vi "PRAT Test Setup.vi"(0 "Station Input":string="A", 1 "Test Sequence Input":T21[](array[typedef]) {"Time" format="%<%H:%M:%S>t"}, 3 "Washer Controls In":T9={"Test Fixture Hardware"={"Power "={"Yokogawa"={"WT210"={"Sample Rate (1: 0.25s)"=1, "A Range (12: 20A)"=12, "V Range (6: 600V)"=4, "Power VISA Yokogawa WT210"="WT210"}, "WT500"={"Power VISA Yokogawa WT500"="WT500", "V Range (8: 1000V)"=0, "I Range (7: 40A)"=0, "Update Rate (3: 500ms)"=2}, "WT310_2"={"Sample Rate (1: 0.25s)"=1, "A Range (12: 20A)"=11, "V Range (6: 600V)"=4, "Power VISA Yokogawa WT310_2"="WT310_2"}, "WT310_3"={"Sample Rate (1: 0.25s)"=1, "A Range (12: 20A)"=11, "V Range (6: 600V)"=4, "Power VISA Yokogawa WT310_3"="WT310_3"}}, "Aplus"={"Aplus IP Address"="192.168.1.101", "Remote Port"=502, "Instrument"="APLUS", "Instr Driver Revision"="1.03.0053"}, "Power Limits"={"Crest Factor"={"Upper Limit"=1.49, "Lower Limit"=1.34}, "Harmonic Content"={"Uthd"=2.0}, "Voltage"={"% Error"=2.0}, "Stability"={"<1 Watt "={"Wattage"=1.0, "Slope (mW/H)"=10.0}, ">1 Watt"={"1%Power/Hour"=1.0}}}, "Nominal Voltage"=120, "Time Limit (s)"=10800.0, "Power Variation Limit (%)"=50.0, "Power Supply"={"Chroma 61605"="CHROMA", "Use Chroma?"=FALSE}}, "Weight Scale"={"Com Options"={"IND560Scale VISA"="IND560", "IP Address"="192.168.1.50", "Remote Port"=502, "Setra Scale VISA"="COM3", "GSE 350"="GSE350"}, "Select Scale"=""}, "Flow Rates"={"Laurel Cold IP Address"="", "Laurel Hot IP Address"="34972A_2", "Hot Water Laurel VISA"="LaurelMeter_Hot", "Cold Water Laurel VISA"="LaurelMeter_Cold", "Remote Port"=0, "Laurel Communication Type"="", "Meters To Collect (Hot Cold)"="", "HOT Laurel Reference"=refnum, "COLD Laurel Reference"=refnum}, "Analog Data"={"Agilent"={"Agilent 34972_1"="34972A_1", "Agilent 34972_2"="34972A_2", "Agilent 34972_3"="34972A_3", "Agilent 34972_4"="34972A_4", "Agilent 34972_5"="34972A_5", "Agilent 34972_6"="34972A_6", "Agilent Gain"=0.0, "TC Type (K,J,T)"="", "Instrument IDN?"="", "TC Channels-List"="", "Analog Channels-List"="", "Agilent Cluster Array"=[], "TC Channels-List 2"="", "Analog Channels-List 2"=""}, "Yokogawa"={"MW100"="MW100", "Intellifaucet"=FALSE}, "Select Analog"="", "TC Coefficients"={"TC Coefficients 1"=[], "TC Coefficients 2"=[], "TC Coefficients 3"=[], "TC Coefficients 4"=[], "TC Coefficients 5"=[], "TC Coefficients 6"=[], "TC Coefficients 7"=[]}, "NI Tasks (Dryer DOE)"=["TC Temps-Module 1", "TC Temps-Module 2", "TC Temps-Module 3", "TC Temps-Module 4", "TC Temps-Module 5", "Gas and Temp-Module 6", "AC_DC Events-Module 7"], "Laurel Analog"={"Laurel IP (Water Temp)"="", "Laurel IP (Pressure)"=""}}, "ITHX-Temp Humidity"={"IP Address 1"="", "Remote Port"=0, "IP Address 2"="", "IP Address 3"=""}, "Gas Meter COM Ports"={"Gas Meter 1"="COM3", "Gas Meter 2"="COM4", "Gas Meter 3"="COM5", "Gas Meter 4"="COM6", "Gas Meter 5"="COM7", "Gas Meter 6"="COM8"}, "Barometric Pressure"={"HEISE 901A"="HEISE", "Use Barometer?"=FALSE}}, "GEA2"={"Address"=35, "Source"=228, "Viper/Hawk"=0}, "DOE Capacity Measurments"={"Weight 1"=35.0, "Model Number 1"="", "Temp 1"=0.0, "Serial Number 1"="", "Lab Number 1"="", "Lab Number 2"="", "Serial Number 2"="", "Temp 2"=0.0, "Model Number 2"="", "Weight 2"=0.0, "Lab Number 3"="", "Serial Number 3"="", "Temp 3"=0.0, "Model Number 3"="", "Weight 3"=0.0, "Lab Number 4"="", "Serial Number 4"="", "Temp 4"=0.0, "Model Number 4"="", "Weight 4"=0.0, "Capacity Measurment Output String"=[]}, "Initialize.Washer In"={"Appliance Details"={"FileVersionInfo"={"FileVersion"="", "ProductName"="", "InternalName"="", "CompanyName"="", "LegalCopyright"="", "FileDescription"=""}, "Dishwasher Info"={"Open Cup Weight (gm):"=0.0, "Auto Cup Weight (gm):"=0.0, "Detergent-Dish:"="", "Inlet Temperature-Dish:"="", "Cycle Mode-Dish:"="", "Unit Control-Dish:"="", "Manufacturer-Dish:"=""}, "Washer Info"={"Hot Water Temperature (Fahrenheit):"="", "Cold Water Temperature (Fahrenheit):"="", "Capacity (cu.ft):"=0.0, "Initial Cloth Weight:"=0.0, "Cloth Lot:"=60, "Model Family:"="", "Program Name:"="", "Cycle Selection:"="", "Wash Temperature:"="", "Rinse Temperature:"="", "Load Size:"=""}, "File Name Output Array"=[], "Calibration Output Array"=[], "Appliance Common"={"Engineer:"="", "Model Number:"="", "Serial Number:"="", "Comments:"="", "Station ID:"="", "Technician:"="", "TR Number:"="", "Lab ID:"="", "Voltage:"="", "Water Pressure (PSI):"="", "Test Date:"="", "Computer Name:"="", "IP Address:"="", "Ambient RH:"="", "Frequency:"="", "Build:"="", "Filename:"="", "Test Type:"="", "Load Run #:"=17, "Ambient Temperature (F):"="", "File Path:"=path "", "Cycles Per Year"=0}, "Water Heater"={"Heating Mode:"=""}, "Dryer"={"Heat Setting:"="", "Washer Water Temperature (60 ± 5°F):"=7, "Water Hardness (PPM):"=7, "Dryness Setting:"="", "Dryer Type:"="", "Exhaust:"="", "Drying Cycle:"="", "Load Type:"="", "Nominal Load Weight"="", "Dryer Initial IMC Data"={"Measured IMC (lbs)"=100.0, "Actual Initial RMC (%)"=7.0, "RMC (Desired %)"=5.0, "Bone Dry Wt(lbs)"=60.0, "Tolerance(%)"=0.0, "Actual Final RMC (%)"=7.0, "CEF (lbf/kWh)"=0.0, "Minimum Weight (lbf)"=0.0, "Average Weight (lbf)"=0.0, "Maximum Weight (lbf)"=0.0, "Measured IMC In Range?"=FALSE, "Moisture Reduction Factor"=55.5, "Field Use Factor"=1.04, "Empty Dryer Cold Weigth"=0.0, "Energy Standard"=enum."D2-Automatic Dryer", "Weight Cloth (lbs)"=0.0, "Relative Moisture Content (%)"=0.0, "Relative Moisture Content - Avg (%)"=0.0}}}, "Display Data (RLT)"={"Status Color"=0, "Serial Number Display"="", "Cycle Count Display"=0, "Station Label Display"="", "Current Run Start Time Display"=0.0, "Board ID Display"="", "RPM Display"=0, "Current Display"=0.0, "Current Path Display"=path "", "Saving Display"=FALSE, "Unit Type Display"=enum."", "Total Time On Display"=0.0, "UI Button"=FALSE}}} {"Initialize.Washer In"."Display Data (RLT)"."Current Display" format="%.2f"; "Initialize.Washer In"."Display Data (RLT)"."Cycle Count Display" format="%04d"; "Initialize.Washer In"."Appliance Details"."Dryer"."Dryer Initial IMC Data"."Maximum Weight (lbf)" format="%03_6g"; "Initialize.Washer In"."Appliance Details"."Dryer"."Dryer Initial IMC Data"."Average Weight (lbf)" format="%03_6g"; "Initialize.Washer In"."Appliance Details"."Dryer"."Dryer Initial IMC Data"."Minimum Weight (lbf)" format="%03_6g"; "Initialize.Washer In"."Appliance Details"."Dryer"."Dryer Initial IMC Data"."CEF (lbf/kWh)" format="%03_6g"; "Initialize.Washer In"."Appliance Details"."Dryer"."Dryer Initial IMC Data"."Actual Final RMC (%)" format="%03_6g"; "Initialize.Washer In"."Appliance Details"."Dryer"."Dryer Initial IMC Data"."Tolerance(%)" format="%0#_6g"; "Initialize.Washer In"."Appliance Details"."Dryer"."Dryer Initial IMC Data"."Bone Dry Wt(lbs)" format="%03_6g"; "Initialize.Washer In"."Appliance Details"."Dryer"."Dryer Initial IMC Data"."RMC (Desired %)" format="%0#_6g"; "Initialize.Washer In"."Appliance Details"."Dryer"."Dryer Initial IMC Data"."Actual Initial RMC (%)" format="%03_6g"; "Initialize.Washer In"."Appliance Details"."Dryer"."Dryer Initial IMC Data"."Measured IMC (lbs)" format="%0#_6g"; "GEA2"."Address" format="%x"; "GEA2"."Source" format="%x"; "GEA2"."Viper/Hawk" items=["Viper", "Hawk"]; "Test Fixture Hardware"."Power"."Yokogawa"."WT310_3"."V Range (6: 600V)" items=["Auto", "15V", "30V", "60V", "150V", "300V", "600V"]; "Test Fixture Hardware"."Power"."Yokogawa"."WT310_3"."A Range (12: 20A)" items=["Auto", "5mA", "10mA", "20mA", "50mA", "100mA", "200mA", "0.5A", "1A", "2A", "5A", "10A", "20A", "50mV", "100mV", "200mV", "2.5V", "5V", "10V"]; "Test Fixture Hardware"."Power"."Yokogawa"."WT310_3"."Sample Rate (1: 0.25s)" items=["0.1s", "0.25s", "0.5s", "1s", "2s", "5s"]; "Test Fixture Hardware"."Power"."Yokogawa"."WT310_2"."V Range (6: 600V)" items=["Auto", "15V", "30V", "60V", "150V", "300V", "600V"]; "Test Fixture Hardware"."Power"."Yokogawa"."WT310_2"."A Range (12: 20A)" items=["Auto", "5mA", "10mA", "20mA", "50mA", "100mA", "200mA", "0.5A", "1A", "2A", "5A", "10A", "20A", "50mV", "100mV", "200mV", "2.5V", "5V", "10V"]; "Test Fixture Hardware"."Power"."Yokogawa"."WT310_2"."Sample Rate (1: 0.25s)" items=["0.1s", "0.25s", "0.5s", "1s", "2s", "5s"]; "Test Fixture Hardware"."Power"."Yokogawa"."WT500"."Update Rate (3: 500ms)" items=["-", "100ms", "200ms", "500ms", "1s", "2s", "5s"]; "Test Fixture Hardware"."Power"."Yokogawa"."WT500"."I Range (7: 40A)" items=["AUTO", "500 mA", "1 A", "2 A", "5 A", "10 A", "20 A", "40 A", "S-AUTO", "50 mV", "100 mV", "200 mV", "500 mV", "1 V", "2 V", "5 V", "10 V", "250 mA", "500 mA", "1 A", "2.5 A", "5 A", "10 A", "20 A", "25 mV", "50 mV", "100 mV", "250 mV", "500 mV", "1 V", "2.5 V", "5 V"]; "Test Fixture Hardware"."Power"."Yokogawa"."WT500"."V Range (8: 1000V)" items=["AUTO", "15", "30", "60", "100", "150", "300", "600", "1000", "7.5", "15", "30", "50", "75", "150", "300", "500"]; "Test Fixture Hardware"."Power"."Yokogawa"."WT210"."V Range (6: 600V)" items=["Auto", "15V", "30V", "60V", "150V", "300V", "600V"]; "Test Fixture Hardware"."Power"."Yokogawa"."WT210"."A Range (12: 20A)" items=["Auto", "5mA", "10mA", "20mA", "50mA", "100mA", "200mA", "0.5A", "1A", "2A", "5A", "10A", "20A", "50mV", "100mV", "200mV", "2.5V", "5V", "10V"]; "Test Fixture Hardware"."Power"."Yokogawa"."WT210"."Sample Rate (1: 0.25s)" items=["0.1s", "0.25s", "0.5s", "1s", "2s", "5s"]}, 4 "Filepath In":T7={"General Setup Paths"={"Calibration File Path"=path "", "DOE Capacity Path"=path "", "Data Folder Path"=path "", "RLT Backup Data Path"=path "", "Tool Base Path"=path "C:/GE/Washer DOE", "General Startup Config Path"=path "", "File Save Previous Run Path"=path "", "File Save Configuration Data Path"=path ""}, "Data File Paths"={"Data File Path"=path "", "Debug File Path"=path "", "Bus Log Path"=path "", "Current"=path "", "Summary"=path ""}, "New Summary Created"=FALSE, "Check Location Interval (Second)"=0}, 5 "Error In":errorcluster, 6 "LV Program":T32=enum."DOE Stand") -> (7 "Cutout Delay (sec)":dbl=240.0, 9 "Unit Setpoint Out":i32, 10 "Appliance Details":T1={"FileVersionInfo"={"FileVersion"="", "ProductName"="", "InternalName"="", "CompanyName"="", "LegalCopyright"="", "FileDescription"=""}, "Dishwasher Info"={"Open Cup Weight (gm):"=0.0, "Auto Cup Weight (gm):"=0.0, "Detergent-Dish:"="", "Inlet Temperature-Dish:"="", "Cycle Mode-Dish:"="", "Unit Control-Dish:"="", "Manufacturer-Dish:"=""}, "Washer Info"={"Hot Water Temperature (Fahrenheit):"="", "Cold Water Temperature (Fahrenheit):"="", "Capacity (cu.ft):"=0.0, "Initial Cloth Weight:"=0.0, "Cloth Lot:"=0, "Model Family:"="", "Program Name:"="", "Cycle Selection:"="", "Wash Temperature:"="", "Rinse Temperature:"="", "Load Size:"=""}, "File Name Output Array"=[], "Calibration Output Array"=[], "Appliance Common"={"Engineer:"="", "Model Number:"="", "Serial Number:"="", "Comments:"="", "Station ID:"="", "Technician:"="", "TR Number:"="", "Lab ID:"="", "Voltage:"="", "Water Pressure (PSI):"="", "Test Date:"="", "Computer Name:"="", "IP Address:"="", "Ambient RH:"="", "Frequency:"="", "Build:"="", "Filename:"="", "Test Type:"="", "Load Run #:"=0, "Ambient Temperature (F):"="", "File Path:"=path "", "Cycles Per Year"=60}, "Water Heater"={"Heating Mode:"=""}, "Dryer"={"Heat Setting:"="", "Washer Water Temperature (60 ± 5°F):"=60, "Water Hardness (PPM):"=17, "Dryness Setting:"="", "Dryer Type:"="", "Exhaust:"="", "Drying Cycle:"="", "Load Type:"="", "Nominal Load Weight"="", "Dryer Initial IMC Data"={"Measured IMC (lbs)"=7.0, "Actual Initial RMC (%)"=7.0, "RMC (Desired %)"=100.0, "Bone Dry Wt(lbs)"=7.0, "Tolerance(%)"=5.0, "Actual Final RMC (%)"=0.0, "CEF (lbf/kWh)"=0.0, "Minimum Weight (lbf)"=0.0, "Average Weight (lbf)"=0.0, "Maximum Weight (lbf)"=0.0, "Measured IMC In Range?"=FALSE, "Moisture Reduction Factor"=55.5, "Field Use Factor"=1.04, "Empty Dryer Cold Weigth"=0.0, "Energy Standard"=enum."D2-Automatic Dryer", "Weight Cloth (lbs)"=0.0, "Relative Moisture Content (%)"=0.0, "Relative Moisture Content - Avg (%)"=0.0}}} {"Dryer"."Dryer Initial IMC Data"."Maximum Weight (lbf)" format="%03_6g"; "Dryer"."Dryer Initial IMC Data"."Average Weight (lbf)" format="%03_6g"; "Dryer"."Dryer Initial IMC Data"."Minimum Weight (lbf)" format="%03_6g"; "Dryer"."Dryer Initial IMC Data"."CEF (lbf/kWh)" format="%03_6g"; "Dryer"."Dryer Initial IMC Data"."Actual Final RMC (%)" format="%03_6g"; "Dryer"."Dryer Initial IMC Data"."Tolerance(%)" format="%0#_6g"; "Dryer"."Dryer Initial IMC Data"."Bone Dry Wt(lbs)" format="%03_6g"; "Dryer"."Dryer Initial IMC Data"."RMC (Desired %)" format="%0#_6g"; "Dryer"."Dryer Initial IMC Data"."Actual Initial RMC (%)" format="%03_6g"; "Dryer"."Dryer Initial IMC Data"."Measured IMC (lbs)" format="%0#_6g"}, 11 "Filepath Out":T7, 12 "Station ID":T31=enum."A", 13 "Log Data Output":bool, 14 "Final Output":T21[](array[typedef]) {"Time" format="%<%H:%M:%S>t"}, 15 "Cancel Output":bool, 16 "Test Procedure":string, 17 "Reset Cycle Count":bool, 18 "New Cycle Count Out":i32, 19 "Error Out":errorcluster)   [LabVIEW 2016]
uses:
  Type Definitions/PRAT Test.ctl
  Utility/Save File/File Setup (Public)/Type Definition/Save File HEWH Heating Control Mode.ctl
  Draw Water Specific/Type Definitions/Terminate Draw Conditions.ctl
  Type Definitions/HEWH Start Conditions.ctl
  Draw Water Specific/Type Definitions/Check Special Condtions.ctl
  Draw Water Specific/Type Definitions/HEWH Special Condition Check.ctl
  Type Definitions/HEWH Draw Flag ENUM.ctl
  Utility/Custom Pallet Controls/Custom Pallet String.ctl
  Custom Instrument Control/MW100/Type Definitions/Station ID Selector.ctl
  Utility/Save File/File Setup (Public)/Type Definition/Save File DOE File Path Control.ctl
  Utility/Save File/File Setup (Public)/Type Definition/Save File DOE Data Save Filepaths.ctl
  Utility/Save File/File Setup (Public)/Type Definition/Save File DOE LabView Program.ctl
  Washer DOE/Type Definitions/DOE Main Control.ctl
  Washer DOE/Type Definitions/DOE Test Fixture Hardware.ctl
  Utility/Type Definitions/UTILITY Power Inputs Control.ctl
  Drivers/IND560 Scale Monitor/Type Definitions/IND560 Configuration.ctl
  Type Definitions/HEWH Agilent Cluster.ctl
  Utility/Type Definitions/UTILITY TC Coefficients.ctl
  Drivers/Omega FMA-1600A Series Gas Flow Meter/Type Definitions/FMA1600A COM Ports.ctl
  Washer DOE/Configuration/GEA2.ctl
  Washer DOE/Type Definitions/DOE Capacity Measurments.ctl
  Utility/Save File/Public/Type Definitions/Save File Washer.ctl
  Utility/Save File/File Setup (Public)/Type Definition/Save File DISH Dishwasher Details.ctl
  <vilib>/Platform/fileVersionInfo.llb/FileVersionInformation.ctl
  Washer DOE/Type Definitions/DOE Appliance Common.ctl
  Utility/Save File/File Setup (Public)/Type Definition/DPT IMC Data.ctl
  Washer DOE/Type Definitions/DOE Dryer Standard.ctl
  Utility/Save File/Public/Type Definitions/Save File Appliance Display.ctl
  Utility/Save File/Public/Type Definitions/Save File Unit Type.ctl
  Draw Water Specific/Type Definitions/Unit Type.ctl
  Utility/Save File/File Setup (Public)/Type Definition/Save File DOE Configuration State.ctl
  Utility/Save File/File Setup.lvlib
  Utility/Save File/Save File.lvlib
panel:
  in  "Test Data Path":path
  in  "Log Data":bool
  out "Save File Path":path
  in  "Test Sequence Output":T21[](array[typedef])=[{"Sequence #"=1.0, "Cycles"=35, "Mode Setting"="", "Flow Rate (GPM)"=0.0, "Temperature (F)"=0.0, "Reset Timer"=FALSE, "Use Temp Decline Method"=FALSE, "Terminate Condition"=enum."C1-Terminate Draw @ Gallon Mark", "Condition Value #1"=0.0, "UE"=FALSE, "LE"=FALSE, "Comp"=FALSE, "Fan"=FALSE, "Test End Time (Sec)"=0.0, "Purge Until Cutout"=FALSE, "Start Conditions"=enum."Heat Source Cutout", "Condition Value #2"=0.0, "Remove Power"=FALSE, "Time"=0.0, "Check Special Cond."=enum."SC2-Check Heat Source (On-C2/Off-C1)", "Condition#"=enum."C1", "Draw Flags"=enum."N/A", "Data Processing Delay (FHD 15sec, UEF 5 Sec)"=0.0, "Test Complete"=FALSE}, {"Sequence #"=2.0, "Cycles"=15, "Mode Setting"="", "Flow Rate (GPM)"=0.0, "Temperature (F)"=0.0, "Reset Timer"=FALSE, "Use Temp Decline Method"=FALSE, "Terminate Condition"=enum."C1-Terminate Draw @ Gallon Mark", "Condition Value #1"=0.0, "UE"=FALSE, "LE"=FALSE, "Comp"=FALSE, "Fan"=FALSE, "Test End Time (Sec)"=0.0, "Purge Until Cutout"=FALSE, "Start Conditions"=enum."Heat Source Cutout", "Condition Value #2"=0.0, "Remove Power"=FALSE, "Time"=0.0, "Check Special Cond."=enum."SC2-Check Heat Source (On-C2/Off-C1)", "Condition#"=enum."C1", "Draw Flags"=enum."N/A", "Data Processing Delay (FHD 15sec, UEF 5 Sec)"=0.0, "Test Complete"=FALSE}, {"Sequence #"=3.0, "Cycles"=35, "Mode Setting"="", "Flow Rate (GPM)"=0.0, "Temperature (F)"=0.0, "Reset Timer"=FALSE, "Use Temp Decline Method"=FALSE, "Terminate Condition"=enum."C1-Terminate Draw @ Gallon Mark", "Condition Value #1"=0.0, "UE"=FALSE, "LE"=FALSE, "Comp"=FALSE, "Fan"=FALSE, "Test End Time (Sec)"=0.0, "Purge Until Cutout"=FALSE, "Start Conditions"=enum."Heat Source Cutout", "Condition Value #2"=0.0, "Remove Power"=FALSE, "Time"=0.0, "Check Special Cond."=enum."SC2-Check Heat Source (On-C2/Off-C1)", "Condition#"=enum."C1", "Draw Flags"=enum."N/A", "Data Processing Delay (FHD 15sec, UEF 5 Sec)"=0.0, "Test Complete"=FALSE}, {"Sequence #"=4.0, "Cycles"=15, "Mode Setting"="", "Flow Rate (GPM)"=0.0, "Temperature (F)"=0.0, "Reset Timer"=FALSE, "Use Temp Decline Method"=FALSE, "Terminate Condition"=enum."C1-Terminate Draw @ Gallon Mark", "Condition Value #1"=0.0, "UE"=FALSE, "LE"=FALSE, "Comp"=FALSE, "Fan"=FALSE, "Test End Time (Sec)"=0.0, "Purge Until Cutout"=FALSE, "Start Conditions"=enum."Heat Source Cutout", "Condition Value #2"=0.0, "Remove Power"=FALSE, "Time"=0.0, "Check Special Cond."=enum."SC2-Check Heat Source (On-C2/Off-C1)", "Condition#"=enum."C1", "Draw Flags"=enum."N/A", "Data Processing Delay (FHD 15sec, UEF 5 Sec)"=0.0, "Test Complete"=FALSE}, {"Sequence #"=5.0, "Cycles"=35, "Mode Setting"="", "Flow Rate (GPM)"=0.0, "Temperature (F)"=0.0, "Reset Timer"=FALSE, "Use Temp Decline Method"=FALSE, "Terminate Condition"=enum."C1-Terminate Draw @ Gallon Mark", "Condition Value #1"=0.0, "UE"=FALSE, "LE"=FALSE, "Comp"=FALSE, "Fan"=FALSE, "Test End Time (Sec)"=0.0, "Purge Until Cutout"=FALSE, "Start Conditions"=enum."Heat Source Cutout", "Condition Value #2"=0.0, "Remove Power"=FALSE, "Time"=0.0, "Check Special Cond."=enum."SC2-Check Heat Source (On-C2/Off-C1)", "Condition#"=enum."C1", "Draw Flags"=enum."N/A", "Data Processing Delay (FHD 15sec, UEF 5 Sec)"=0.0, "Test Complete"=FALSE}, {"Sequence #"=6.0, "Cycles"=15, "Mode Setting"="", "Flow Rate (GPM)"=0.0, "Temperature (F)"=0.0, "Reset Timer"=FALSE, "Use Temp Decline Method"=FALSE, "Terminate Condition"=enum."C1-Terminate Draw @ Gallon Mark", "Condition Value #1"=0.0, "UE"=FALSE, "LE"=FALSE, "Comp"=FALSE, "Fan"=FALSE, "Test End Time (Sec)"=0.0, "Purge Until Cutout"=FALSE, "Start Conditions"=enum."Heat Source Cutout", "Condition Value #2"=0.0, "Remove Power"=FALSE, "Time"=0.0, "Check Special Cond."=enum."SC2-Check Heat Source (On-C2/Off-C1)", "Condition#"=enum."C1", "Draw Flags"=enum."N/A", "Data Processing Delay (FHD 15sec, UEF 5 Sec)"=0.0, "Test Complete"=FALSE}, {"Sequence #"=7.0, "Cycles"=35, "Mode Setting"="", "Flow Rate (GPM)"=0.0, "Temperature (F)"=0.0, "Reset Timer"=FALSE, "Use Temp Decline Method"=FALSE, "Terminate Condition"=enum."C1-Terminate Draw @ Gallon Mark", "Condition Value #1"=0.0, "UE"=FALSE, "LE"=FALSE, "Comp"=FALSE, "Fan"=FALSE, "Test End Time (Sec)"=0.0, "Purge Until Cutout"=FALSE, "Start Conditions"=enum."Heat Source Cutout", "Condition Value #2"=0.0, "Remove Power"=FALSE, "Time"=0.0, "Check Special Cond."=enum."SC2-Check Heat Source (On-C2/Off-C1)", "Condition#"=enum."C1", "Draw Flags"=enum."N/A", "Data Processing Delay (FHD 15sec, UEF 5 Sec)"=0.0, "Test Complete"=FALSE}, {"Sequence #"=8.0, "Cycles"=15, "Mode Setting"="", "Flow Rate (GPM)"=0.0, "Temperature (F)"=0.0, "Reset Timer"=FALSE, "Use Temp Decline Method"=FALSE, "Terminate Condition"=enum."C1-Terminate Draw @ Gallon Mark", "Condition Value #1"=0.0, "UE"=FALSE, "LE"=FALSE, "Comp"=FALSE, "Fan"=FALSE, "Test End Time (Sec)"=0.0, "Purge Until Cutout"=FALSE, "Start Conditions"=enum."Heat Source Cutout", "Condition Value #2"=0.0, "Remove Power"=FALSE, "Time"=0.0, "Check Special Cond."=enum."SC2-Check Heat Source (On-C2/Off-C1)", "Condition#"=enum."C1", "Draw Flags"=enum."N/A", "Data Processing Delay (FHD 15sec, UEF 5 Sec)"=0.0, "Test Complete"=FALSE}] {"Time" format="%<%H:%M:%S>t"}
  in  "Cancel":bool
  in  "Complete/Update":bool
  out "Message":T4="Test Setup"
  in  "Tab Control 3":T28(tab)
  in  "Write 11":bool caption="Write"
  in  "Write 10":bool caption="Write"
  in  "Write 9":bool caption="Write"
  in  "Write 8":bool caption="Write"
  in  "Write 7":bool caption="Write"
  in  "Write 6":bool caption="Write"
  in  "Write 5":bool caption="Write"
  in  "Write 4":bool caption="Write"
  in  "Write 3":bool caption="Write"
  in  "Write 2":bool caption="Write"
  in  "Write":bool
  in  "24Hr High Thermostat Test":bool
  in  "24Hr Med Thermostat Test":bool
  in  "Unit Setpoint":i32=125
  in  "Unit Type":T29
  in  "Heating Mode":string(combo)="Hybrid"
  in  "Temperature Decrease (°F)":dbl=15.0 format="%#_13g"
  in  "Update":bool
  in  "1st Hour DOE":bool
  in  "Read Previous Cycle Count":bool
  in  "24 Hour DOE - Low Usage":bool
  in  "24 Hour DOE - Medium Usage":bool
  in  "24 Hour DOE - High Usage":bool
  in  "24 Hour DOE - Standard":bool
  in  "RLT":bool
  in  "PRAT 1 Year Equiv":bool
  in  "PRAT 2.5 Year Equiv":bool
  in  "Update for Northern Climate":bool
  in  "Northern Climate\nInlet Temperature (°F)":dbl=50.0 format="%#_13g"
  in  "Update Cycle Count":bool
  in  "New Cycle Count":i32
  in  "Standard Heat-Up":bool
  in  "Heat-Up Audit Test":bool
  in  "Custom Test":T21[](array[typedef])=[{"Sequence #"=1.0, "Cycles"=10, "Mode Setting"="", "Flow Rate (GPM)"=1.0, "Temperature (F)"=58.0, "Reset Timer"=FALSE, "Use Temp Decline Method"=FALSE, "Terminate Condition"=enum."C1-Terminate Draw @ Gallon Mark", "Condition Value #1"=1.0, "UE"=FALSE, "LE"=FALSE, "Comp"=FALSE, "Fan"=FALSE, "Test End Time (Sec)"=0.0, "Purge Until Cutout"=FALSE, "Start Conditions"=enum."Every X (Seconds)", "Condition Value #2"=30.0, "Remove Power"=FALSE, "Time"=0.0, "Check Special Cond."=enum."SC2-Check Heat Source (On-C2/Off-C1)", "Condition#"=enum."N/A", "Draw Flags"=enum."N/A", "Data Processing Delay (FHD 15sec, UEF 5 Sec)"=0.0, "Test Complete"=FALSE}] {"Time" format="%<%H:%M:%S>t"}
  in  "Custom Test":bool
  out "Seconds Conv2":i32 caption="Seconds"
  in  "Time Conv2":i32 caption="Time" format="%<%H:%M:%S>t"
  in  "Seconds":dbl
  out "Time":string
  in  "Enable Standard Test Override":bool
  in  "Tab Control 2":T30(tab)
  in  "24Hr High Thermostat Test Profile":T21[](array[typedef])=[{"Sequence #"=1.0, "Cycles"=1, "Mode Setting"="", "Flow Rate (GPM)"=3.0, "Temperature (F)"=58.0, "Reset Timer"=FALSE, "Use Temp Decline Method"=FALSE, "Terminate Condition"=enum."C9-Do Nothing", "Condition Value #1"=0.0, "UE"=FALSE, "LE"=FALSE, "Comp"=FALSE, "Fan"=FALSE, "Test End Time (Sec)"=0.0, "Purge Until Cutout"=FALSE, "Start Conditions"=enum."Heat Source Cutout", "Condition Value #2"=0.0, "Remove Power"=FALSE, "Time"=82800.0, "Check Special Cond."=enum."SC1-Do Nothing", "Condition#"=enum."N/A", "Draw Flags"=enum."N/A", "Data Processing Delay (FHD 15sec, UEF 5 Sec)"=5.0, "Test Complete"=FALSE}, {"Sequence #"=2.0, "Cycles"=1, "Mode Setting"="", "Flow Rate (GPM)"=3.0, "Temperature (F)"=58.0, "Reset Timer"=FALSE, "Use Temp Decline Method"=FALSE, "Terminate Condition"=enum."C9-Do Nothing", "Condition Value #1"=0.0, "UE"=FALSE, "LE"=FALSE, "Comp"=FALSE, "Fan"=FALSE, "Test End Time (Sec)"=0.0, "Purge Until Cutout"=FALSE, "Start Conditions"=enum."Heat Source Cutout", "Condition Value #2"=0.0, "Remove Power"=FALSE, "Time"=82800.0, "Check Special Cond."=enum."SC1-Do Nothing", "Condition#"=enum."N/A", "Draw Flags"=enum."N/A", "Data Processing Delay (FHD 15sec, UEF 5 Sec)"=5.0, "Test Complete"=FALSE}, {"Sequence #"=3.0, "Cycles"=1, "Mode Setting"="", "Flow Rate (GPM)"=3.0, "Temperature (F)"=58.0, "Reset Timer"=FALSE, "Use Temp Decline Method"=FALSE, "Terminate Condition"=enum."C9-Do Nothing", "Condition Value #1"=0.0, "UE"=FALSE, "LE"=FALSE, "Comp"=FALSE, "Fan"=FALSE, "Test End Time (Sec)"=0.0, "Purge Until Cutout"=FALSE, "Start Conditions"=enum."Every X (Seconds)", "Condition Value #2"=3600.0, "Remove Power"=FALSE, "Time"=82800.0, "Check Special Cond."=enum."SC1-Do Nothing", "Condition#"=enum."N/A", "Draw Flags"=enum."N/A", "Data Processing Delay (FHD 15sec, UEF 5 Sec)"=5.0, "Test Complete"=FALSE}, {"Sequence #"=4.0, "Cycles"=1, "Mode Setting"="", "Flow Rate (GPM)"=3.0, "Temperature (F)"=58.0, "Reset Timer"=TRUE, "Use Temp Decline Method"=TRUE, "Terminate Condition"=enum."C1-Terminate Draw @ Gallon Mark", "Condition Value #1"=27.0, "UE"=FALSE, "LE"=FALSE, "Comp"=FALSE, "Fan"=FALSE, "Test End Time (Sec)"=0.0, "Purge Until Cutout"=FALSE, "Start Conditions"=enum."At Time (Seconds)", "Condition Value #2"=0.0, "Remove Power"=FALSE, "Time"=82800.0, "Check Special Cond."=enum."SC1-Do Nothing", "Condition#"=enum."N/A", "Draw Flags"=enum."N/A", "Data Processing Delay (FHD 15sec, UEF 5 Sec)"=5.0, "Test Complete"=FALSE}, {"Sequence #"=5.0, "Cycles"=1, "Mode Setting"="", "Flow Rate (GPM)"=1.0, "Temperature (F)"=58.0, "Reset Timer"=FALSE, "Use Temp Decline Method"=FALSE, "Terminate Condition"=enum."C1-Terminate Draw @ Gallon Mark", "Condition Value #1"=2.0, "UE"=FALSE, "LE"=FALSE, "Comp"=FALSE, "Fan"=FALSE, "Test End Time (Sec)"=0.0, "Purge Until Cutout"=FALSE, "Start Conditions"=enum."At Time (Seconds)", "Condition Value #2"=1800.0, "Remove Power"=FALSE, "Time"=82800.0, "Check Special Cond."=enum."SC1-Do Nothing", "Condition#"=enum."N/A", "Draw Flags"=enum."N/A", "Data Processing Delay (FHD 15sec, UEF 5 Sec)"=5.0, "Test Complete"=FALSE}, {"Sequence #"=6.0, "Cycles"=1, "Mode Setting"="", "Flow Rate (GPM)"=1.0, "Temperature (F)"=58.0, "Reset Timer"=FALSE, "Use Temp Decline Method"=FALSE, "Terminate Condition"=enum."C1-Terminate Draw @ Gallon Mark", "Condition Value #1"=1.0, "UE"=FALSE, "LE"=FALSE, "Comp"=FALSE, "Fan"=FALSE, "Test End Time (Sec)"=0.0, "Purge Until Cutout"=FALSE, "Start Conditions"=enum."At Time (Seconds)", "Condition Value #2"=2400.0, "Remove Power"=FALSE, "Time"=82800.0, "Check Special Cond."=enum."SC1-Do Nothing", "Condition#"=enum."N/A", "Draw Flags"=enum."N/A", "Data Processing Delay (FHD 15sec, UEF 5 Sec)"=5.0, "Test Complete"=FALSE}, {"Sequence #"=7.0, "Cycles"=1, "Mode Setting"="", "Flow Rate (GPM)"=1.7, "Temperature (F)"=58.0, "Reset Timer"=FALSE, "Use Temp Decline Method"=FALSE, "Terminate Condition"=enum."C1-Terminate Draw @ Gallon Mark", "Condition Value #1"=9.0, "UE"=FALSE, "LE"=FALSE, "Comp"=FALSE, "Fan"=FALSE, "Test End Time (Sec)"=0.0, "Purge Until Cutout"=FALSE, "Start Conditions"=enum."At Time (Seconds)", "Condition Value #2"=6000.0, "Remove Power"=TRUE, "Time"=5700.0, "Check Special Cond."=enum."SC1-Do Nothing", "Condition#"=enum."N/A", "Draw Flags"=enum."N/A", "Data Processing Delay (FHD 15sec, UEF 5 Sec)"=5.0, "Test Complete"=FALSE}, {"Sequence #"=8.0, "Cycles"=1, "Mode Setting"="", "Flow Rate (GPM)"=3.0, "Temperature (F)"=58.0, "Reset Timer"=FALSE, "Use Temp Decline Method"=FALSE, "Terminate Condition"=enum."C1-Terminate Draw @ Gallon Mark", "Condition Value #1"=15.0, "UE"=FALSE, "LE"=FALSE, "Comp"=FALSE, "Fan"=FALSE, "Test End Time (Sec)"=0.0, "Purge Until Cutout"=FALSE, "Start Conditions"=enum."At Time (Seconds)", "Condition Value #2"=37800.0, "Remove Power"=FALSE, "Time"=37500.0, "Check Special Cond."=enum."SC1-Do Nothing", "Condition#"=enum."N/A", "Draw Flags"=enum."N/A", "Data Processing Delay (FHD 15sec, UEF 5 Sec)"=5.0, "Test Complete"=FALSE}, {"Sequence #"=9.0, "Cycles"=1, "Mode Setting"="", "Flow Rate (GPM)"=1.7, "Temperature (F)"=58.0, "Reset Timer"=FALSE, "Use Temp Decline Method"=FALSE, "Terminate Condition"=enum."C1-Terminate Draw @ Gallon Mark", "Condition Value #1"=5.0, "UE"=FALSE, "LE"=FALSE, "Comp"=FALSE, "Fan"=FALSE, "Test End Time (Sec)"=0.0, "Purge Until Cutout"=FALSE, "Start Conditions"=enum."At Time (Seconds)", "Condition Value #2"=41400.0, "Remove Power"=TRUE, "Time"=41100.0, "Check Special Cond."=enum."SC1-Do Nothing", "Condition#"=enum."N/A", "Draw Flags"=enum."N/A", "Data Processing Delay (FHD 15sec, UEF 5 Sec)"=5.0, "Test Complete"=FALSE}, {"Sequence #"=10.0, "Cycles"=1, "Mode Setting"="", "Flow Rate (GPM)"=1.0, "Temperature (F)"=58.0, "Reset Timer"=FALSE, "Use Temp Decline Method"=FALSE, "Terminate Condition"=enum."C1-Terminate Draw @ Gallon Mark", "Condition Value #1"=1.0, "UE"=FALSE, "LE"=FALSE, "Comp"=FALSE, "Fan"=FALSE, "Test End Time (Sec)"=0.0, "Purge Until Cutout"=FALSE, "Start Conditions"=enum."At Time (Seconds)", "Condition Value #2"=43200.0, "Remove Power"=TRUE, "Time"=0.0, "Check Special Cond."=enum."SC1-Do Nothing", "Condition#"=enum."N/A", "Draw Flags"=enum."N/A", "Data Processing Delay (FHD 15sec, UEF 5 Sec)"=5.0, "Test Complete"=FALSE}, {"Sequence #"=11.0, "Cycles"=1, "Mode Setting"="", "Flow Rate (GPM)"=1.0, "Temperature (F)"=58.0, "Reset Timer"=FALSE, "Use Temp Decline Method"=FALSE, "Terminate Condition"=enum."C1-Terminate Draw @ Gallon Mark", "Condition Value #1"=1.0, "UE"=FALSE, "LE"=FALSE, "Comp"=FALSE, "Fan"=FALSE, "Test End Time (Sec)"=0.0, "Purge Until Cutout"=FALSE, "Start Conditions"=enum."At Time (Seconds)", "Condition Value #2"=45900.0, "Remove Power"=TRUE, "Time"=0.0, "Check Special Cond."=enum."SC1-Do Nothing", "Condition#"=enum."N/A", "Draw Flags"=enum."N/A", "Data Processing Delay (FHD 15sec, UEF 5 Sec)"=5.0, "Test Complete"=FALSE}, {"Sequence #"=12.0, "Cycles"=1, "Mode Setting"="", "Flow Rate (GPM)"=1.0, "Temperature (F)"=58.0, "Reset Timer"=FALSE, "Use Temp Decline Method"=FALSE, "Terminate Condition"=enum."C1-Terminate Draw @ Gallon Mark", "Condition Value #1"=1.0, "UE"=FALSE, "LE"=FALSE, "Comp"=FALSE, "Fan"=FALSE, "Test End Time (Sec)"=0.0, "Purge Until Cutout"=FALSE, "Start Conditions"=enum."At Time (Seconds)", "Condition Value #2"=46200.0, "Remove Power"=TRUE, "Time"=0.0, "Check Special Cond."=enum."SC1-Do Nothing", "Condition#"=enum."N/A", "Draw Flags"=enum."N/A", "Data Processing Delay (FHD 15sec, UEF 5 Sec)"=5.0, "Test Complete"=FALSE}, {"Sequence #"=13.0, "Cycles"=1, "Mode Setting"="", "Flow Rate (GPM)"=1.0, "Temperature (F)"=58.0, "Reset Timer"=FALSE, "Use Temp Decline Method"=FALSE, "Terminate Condition"=enum."C1-Terminate Draw @ Gallon Mark", "Condition Value #1"=2.0, "UE"=FALSE, "LE"=FALSE, "Comp"=FALSE, "Fan"=FALSE, "Test End Time (Sec)"=0.0, "Purge Until Cutout"=FALSE, "Start Conditions"=enum."At Time (Seconds)", "Condition Value #2"=57600.0, "Remove Power"=TRUE, "Time"=0.0, "Check Special Cond."=enum."SC1-Do Nothing", "Condition#"=enum."N/A", "Draw Flags"=enum."N/A", "Data Processing Delay (FHD 15sec, UEF 5 Sec)"=5.0, "Test Complete"=FALSE}, {"Sequence #"=14.0, "Cycles"=1, "Mode Setting"="", "Flow Rate (GPM)"=1.0, "Temperature (F)"=58.0, "Reset Timer"=FALSE, "Use Temp Decline Method"=FALSE, "Terminate Condition"=enum."C1-Terminate Draw @ Gallon Mark", "Condition Value #1"=2.0, "UE"=FALSE, "LE"=FALSE, "Comp"=FALSE, "Fan"=FALSE, "Test End Time (Sec)"=0.0, "Purge Until Cutout"=FALSE, "Start Conditions"=enum."At Time (Seconds)", "Condition Value #2"=58500.0, "Remove Power"=TRUE, "Time"=0.0, "Check Special Cond."=enum."SC1-Do Nothing", "Condition#"=enum."N/A", "Draw Flags"=enum."N/A", "Data Processing Delay (FHD 15sec, UEF 5 Sec)"=5.0, "Test Complete"=FALSE}, {"Sequence #"=15.0, "Cycles"=1, "Mode Setting"="", "Flow Rate (GPM)"=1.7, "Temperature (F)"=58.0, "Reset Timer"=FALSE, "Use Temp Decline Method"=FALSE, "Terminate Condition"=enum."C1-Terminate Draw @ Gallon Mark", "Condition Value #1"=2.0, "UE"=FALSE, "LE"=FALSE, "Comp"=FALSE, "Fan"=FALSE, "Test End Time (Sec)"=0.0, "Purge Until Cutout"=FALSE, "Start Conditions"=enum."At Time (Seconds)", "Condition Value #2"=59400.0, "Remove Power"=FALSE, "Time"=59100.0, "Check Special Cond."=enum."SC1-Do Nothing", "Condition#"=enum."N/A", "Draw Flags"=enum."N/A", "Data Processing Delay (FHD 15sec, UEF 5 Sec)"=5.0, "Test Complete"=FALSE}, {"Sequence #"=16.0, "Cycles"=1, "Mode Setting"="", "Flow Rate (GPM)"=1.7, "Temperature (F)"=58.0, "Reset Timer"=FALSE, "Use Temp Decline Method"=FALSE, "Terminate Condition"=enum."C1-Terminate Draw @ Gallon Mark", "Condition Value #1"=2.0, "UE"=FALSE, "LE"=FALSE, "Comp"=FALSE, "Fan"=FALSE, "Test End Time (Sec)"=0.0, "Purge Until Cutout"=FALSE, "Start Conditions"=enum."At Time (Seconds)", "Condition Value #2"=60300.0, "Remove Power"=FALSE, "Time"=0.0, "Check Special Cond."=enum."SC1-Do Nothing", "Condition#"=enum."N/A", "Draw Flags"=enum."N/A", "Data Processing Delay (FHD 15sec, UEF 5 Sec)"=5.0, "Test Complete"=FALSE}, {"Sequence #"=17.0, "Cycles"=1, "Mode Setting"="", "Flow Rate (GPM)"=3.0, "Temperature (F)"=58.0, "Reset Timer"=FALSE, "Use Temp Decline Method"=FALSE, "Terminate Condition"=enum."C1-Terminate Draw @ Gallon Mark", "Condition Value #1"=14.0, "UE"=FALSE, "LE"=FALSE, "Comp"=FALSE, "Fan"=FALSE, "Test End Time (Sec)"=86400.0, "Purge Until Cutout"=FALSE, "Start Conditions"=enum."At Time (Seconds)", "Condition Value #2"=61200.0, "Remove Power"=TRUE, "Time"=68400.0, "Check Special Cond."=enum."SC1-Do Nothing", "Condition#"=enum."N/A", "Draw Flags"=enum."N/A", "Data Processing Delay (FHD 15sec, UEF 5 Sec)"=5.0, "Test Complete"=FALSE}] {"Time" format="%<%H:%M:%S>t"}
  in  "24HR Medium Thermostat Test":T21[](array[typedef])=[{"Sequence #"=1.0, "Cycles"=1, "Mode Setting"="", "Flow Rate (GPM)"=3.0, "Temperature (F)"=58.0, "Reset Timer"=FALSE, "Use Temp Decline Method"=FALSE, "Terminate Condition"=enum."C9-Do Nothing", "Condition Value #1"=0.0, "UE"=FALSE, "LE"=FALSE, "Comp"=FALSE, "Fan"=FALSE, "Test End Time (Sec)"=0.0, "Purge Until Cutout"=FALSE, "Start Conditions"=enum."Heat Source Cutout", "Condition Value #2"=0.0, "Remove Power"=FALSE, "Time"=0.0, "Check Special Cond."=enum."SC1-Do Nothing", "Condition#"=enum."N/A", "Draw Flags"=enum."N/A", "Data Processing Delay (FHD 15sec, UEF 5 Sec)"=5.0, "Test Complete"=FALSE}, {"Sequence #"=2.0, "Cycles"=1, "Mode Setting"="", "Flow Rate (GPM)"=3.0, "Temperature (F)"=58.0, "Reset Timer"=FALSE, "Use Temp Decline Method"=FALSE, "Terminate Condition"=enum."C9-Do Nothing", "Condition Value #1"=0.0, "UE"=FALSE, "LE"=FALSE, "Comp"=FALSE, "Fan"=FALSE, "Test End Time (Sec)"=0.0, "Purge Until Cutout"=FALSE, "Start Conditions"=enum."Heat Source Cutout", "Condition Value #2"=0.0, "Remove Power"=FALSE, "Time"=0.0, "Check Special Cond."=enum."SC1-Do Nothing", "Condition#"=enum."N/A", "Draw Flags"=enum."N/A", "Data Processing Delay (FHD 15sec, UEF 5 Sec)"=5.0, "Test Complete"=FALSE}, {"Sequence #"=3.0, "Cycles"=1, "Mode Setting"="", "Flow Rate (GPM)"=3.0, "Temperature (F)"=58.0, "Reset Timer"=FALSE, "Use Temp Decline Method"=FALSE, "Terminate Condition"=enum."C9-Do Nothing", "Condition Value #1"=0.0, "UE"=FALSE, "LE"=FALSE, "Comp"=FALSE, "Fan"=FALSE, "Test End Time (Sec)"=0.0, "Purge Until Cutout"=FALSE, "Start Conditions"=enum."Every X (Seconds)", "Condition Value #2"=3600.0, "Remove Power"=FALSE, "Time"=0.0, "Check Special Cond."=enum."SC1-Do Nothing", "Condition#"=enum."N/A", "Draw Flags"=enum."N/A", "Data Processing Delay (FHD 15sec, UEF 5 Sec)"=5.0, "Test Complete"=FALSE}, {"Sequence #"=4.0, "Cycles"=1, "Mode Setting"="", "Flow Rate (GPM)"=1.7, "Temperature (F)"=58.0, "Reset Timer"=TRUE, "Use Temp Decline Method"=TRUE, "Terminate Condition"=enum."C1-Terminate Draw @ Gallon Mark", "Condition Value #1"=15.0, "UE"=FALSE, "LE"=FALSE, "Comp"=FALSE, "Fan"=FALSE, "Test End Time (Sec)"=0.0, "Purge Until Cutout"=FALSE, "Start Conditions"=enum."At Time (Seconds)", "Condition Value #2"=0.0, "Remove Power"=FALSE, "Time"=0.0, "Check Special Cond."=enum."SC1-Do Nothing", "Condition#"=enum."N/A", "Draw Flags"=enum."N/A", "Data Processing Delay (FHD 15sec, UEF 5 Sec)"=5.0, "Test Complete"=FALSE}, {"Sequence #"=5.0, "Cycles"=1, "Mode Setting"="", "Flow Rate (GPM)"=1.0, "Temperature (F)"=58.0, "Reset Timer"=FALSE, "Use Temp Decline Method"=FALSE, "Terminate Condition"=enum."C1-Terminate Draw @ Gallon Mark", "Condition Value #1"=2.0, "UE"=FALSE, "LE"=FALSE, "Comp"=FALSE, "Fan"=FALSE, "Test End Time (Sec)"=0.0, "Purge Until Cutout"=FALSE, "Start Conditions"=enum."At Time (Seconds)", "Condition Value #2"=1800.0, "Remove Power"=FALSE, "Time"=1800.0, "Check Special Cond."=enum."SC1-Do Nothing", "Condition#"=enum."N/A", "Draw Flags"=enum."N/A", "Data Processing Delay (FHD 15sec, UEF 5 Sec)"=5.0, "Test Complete"=FALSE}, {"Sequence #"=6.0, "Cycles"=1, "Mode Setting"="", "Flow Rate (GPM)"=1.7, "Temperature (F)"=58.0, "Reset Timer"=FALSE, "Use Temp Decline Method"=FALSE, "Terminate Condition"=enum."C1-Terminate Draw @ Gallon Mark", "Condition Value #1"=9.0, "UE"=FALSE, "LE"=FALSE, "Comp"=FALSE, "Fan"=FALSE, "Test End Time (Sec)"=0.0, "Purge Until Cutout"=FALSE, "Start Conditions"=enum."At Time (Seconds)", "Condition Value #2"=6000.0, "Remove Power"=TRUE, "Time"=5700.0, "Check Special Cond."=enum."SC1-Do Nothing", "Condition#"=enum."N/A", "Draw Flags"=enum."N/A", "Data Processing Delay (FHD 15sec, UEF 5 Sec)"=5.0, "Test Complete"=FALSE}, {"Sequence #"=7.0, "Cycles"=1, "Mode Setting"="", "Flow Rate (GPM)"=1.7, "Temperature (F)"=58.0, "Reset Timer"=FALSE, "Use Temp Decline Method"=FALSE, "Terminate Condition"=enum."C1-Terminate Draw @ Gallon Mark", "Condition Value #1"=9.0, "UE"=FALSE, "LE"=FALSE, "Comp"=FALSE, "Fan"=FALSE, "Test End Time (Sec)"=0.0, "Purge Until Cutout"=FALSE, "Start Conditions"=enum."At Time (Seconds)", "Condition Value #2"=37800.0, "Remove Power"=FALSE, "Time"=37800.0, "Check Special Cond."=enum."SC1-Do Nothing", "Condition#"=enum."N/A", "Draw Flags"=enum."N/A", "Data Processing Delay (FHD 15sec, UEF 5 Sec)"=5.0, "Test Complete"=FALSE}, {"Sequence #"=8.0, "Cycles"=1, "Mode Setting"="", "Flow Rate (GPM)"=1.7, "Temperature (F)"=58.0, "Reset Timer"=FALSE, "Use Temp Decline Method"=FALSE, "Terminate Condition"=enum."C1-Terminate Draw @ Gallon Mark", "Condition Value #1"=5.0, "UE"=FALSE, "LE"=FALSE, "Comp"=FALSE, "Fan"=FALSE, "Test End Time (Sec)"=0.0, "Purge Until Cutout"=FALSE, "Start Conditions"=enum."At Time (Seconds)", "Condition Value #2"=41400.0, "Remove Power"=TRUE, "Time"=41280.0, "Check Special Cond."=enum."SC1-Do Nothing", "Condition#"=enum."N/A", "Draw Flags"=enum."N/A", "Data Processing Delay (FHD 15sec, UEF 5 Sec)"=5.0, "Test Complete"=FALSE}, {"Sequence #"=9.0, "Cycles"=1, "Mode Setting"="", "Flow Rate (GPM)"=1.0, "Temperature (F)"=58.0, "Reset Timer"=FALSE, "Use Temp Decline Method"=FALSE, "Terminate Condition"=enum."C1-Terminate Draw @ Gallon Mark", "Condition Value #1"=1.0, "UE"=FALSE, "LE"=FALSE, "Comp"=FALSE, "Fan"=FALSE, "Test End Time (Sec)"=0.0, "Purge Until Cutout"=FALSE, "Start Conditions"=enum."At Time (Seconds)", "Condition Value #2"=43200.0, "Remove Power"=TRUE, "Time"=0.0, "Check Special Cond."=enum."SC1-Do Nothing", "Condition#"=enum."N/A", "Draw Flags"=enum."N/A", "Data Processing Delay (FHD 15sec, UEF 5 Sec)"=5.0, "Test Complete"=FALSE}, {"Sequence #"=10.0, "Cycles"=1, "Mode Setting"="", "Flow Rate (GPM)"=1.0, "Temperature (F)"=58.0, "Reset Timer"=FALSE, "Use Temp Decline Method"=FALSE, "Terminate Condition"=enum."C1-Terminate Draw @ Gallon Mark", "Condition Value #1"=1.0, "UE"=FALSE, "LE"=FALSE, "Comp"=FALSE, "Fan"=FALSE, "Test End Time (Sec)"=0.0, "Purge Until Cutout"=FALSE, "Start Conditions"=enum."At Time (Seconds)", "Condition Value #2"=45900.0, "Remove Power"=TRUE, "Time"=0.0, "Check Special Cond."=enum."SC1-Do Nothing", "Condition#"=enum."N/A", "Draw Flags"=enum."N/A", "Data Processing Delay (FHD 15sec, UEF 5 Sec)"=5.0, "Test Complete"=FALSE}, {"Sequence #"=11.0, "Cycles"=1, "Mode Setting"="", "Flow Rate (GPM)"=1.0, "Temperature (F)"=58.0, "Reset Timer"=FALSE, "Use Temp Decline Method"=FALSE, "Terminate Condition"=enum."C1-Terminate Draw @ Gallon Mark", "Condition Value #1"=1.0, "UE"=FALSE, "LE"=FALSE, "Comp"=FALSE, "Fan"=FALSE, "Test End Time (Sec)"=0.0, "Purge Until Cutout"=FALSE, "Start Conditions"=enum."At Time (Seconds)", "Condition Value #2"=46200.0, "Remove Power"=TRUE, "Time"=0.0, "Check Special Cond."=enum."SC1-Do Nothing", "Condition#"=enum."N/A", "Draw Flags"=enum."N/A", "Data Processing Delay (FHD 15sec, UEF 5 Sec)"=5.0, "Test Complete"=FALSE}, {"Sequence #"=12.0, "Cycles"=1, "Mode Setting"="", "Flow Rate (GPM)"=1.0, "Temperature (F)"=58.0, "Reset Timer"=FALSE, "Use Temp Decline Method"=FALSE, "Terminate Condition"=enum."C1-Terminate Draw @ Gallon Mark", "Condition Value #1"=1.0, "UE"=FALSE, "LE"=FALSE, "Comp"=FALSE, "Fan"=FALSE, "Test End Time (Sec)"=0.0, "Purge Until Cutout"=FALSE, "Start Conditions"=enum."At Time (Seconds)", "Condition Value #2"=57600.0, "Remove Power"=TRUE, "Time"=0.0, "Check Special Cond."=enum."SC1-Do Nothing", "Condition#"=enum."N/A", "Draw Flags"=enum."N/A", "Data Processing Delay (FHD 15sec, UEF 5 Sec)"=5.0, "Test Complete"=FALSE}, {"Sequence #"=13.0, "Cycles"=1, "Mode Setting"="", "Flow Rate (GPM)"=1.0, "Temperature (F)"=58.0, "Reset Timer"=FALSE, "Use Temp Decline Method"=FALSE, "Terminate Condition"=enum."C1-Terminate Draw @ Gallon Mark", "Condition Value #1"=2.0, "UE"=FALSE, "LE"=FALSE, "Comp"=FALSE, "Fan"=FALSE, "Test End Time (Sec)"=0.0, "Purge Until Cutout"=FALSE, "Start Conditions"=enum."At Time (Seconds)", "Condition Value #2"=58500.0, "Remove Power"=TRUE, "Time"=0.0, "Check Special Cond."=enum."SC1-Do Nothing", "Condition#"=enum."N/A", "Draw Flags"=enum."N/A", "Data Processing Delay (FHD 15sec, UEF 5 Sec)"=5.0, "Test Complete"=FALSE}, {"Sequence #"=14.0, "Cycles"=1, "Mode Setting"="", "Flow Rate (GPM)"=1.7, "Temperature (F)"=58.0, "Reset Timer"=FALSE, "Use Temp Decline Method"=FALSE, "Terminate Condition"=enum."C1-Terminate Draw @ Gallon Mark", "Condition Value #1"=2.0, "UE"=FALSE, "LE"=FALSE, "Comp"=FALSE, "Fan"=FALSE, "Test End Time (Sec)"=0.0, "Purge Until Cutout"=FALSE, "Start Conditions"=enum."At Time (Seconds)", "Condition Value #2"=60300.0, "Remove Power"=TRUE, "Time"=0.0, "Check Special Cond."=enum."SC1-Do Nothing", "Condition#"=enum."N/A", "Draw Flags"=enum."N/A", "Data Processing Delay (FHD 15sec, UEF 5 Sec)"=5.0, "Test Complete"=FALSE}, {"Sequence #"=15.0, "Cycles"=1, "Mode Setting"="", "Flow Rate (GPM)"=1.7, "Temperature (F)"=58.0, "Reset Timer"=FALSE, "Use Temp Decline Method"=FALSE, "Terminate Condition"=enum."C1-Terminate Draw @ Gallon Mark", "Condition Value #1"=7.0, "UE"=FALSE, "LE"=FALSE, "Comp"=FALSE, "Fan"=FALSE, "Test End Time (Sec)"=0.0, "Purge Until Cutout"=FALSE, "Start Conditions"=enum."At Time (Seconds)", "Condition Value #2"=61200.0, "Remove Power"=FALSE, "Time"=60780.0, "Check Special Cond."=enum."SC1-Do Nothing", "Condition#"=enum."N/A", "Draw Flags"=enum."N/A", "Data Processing Delay (FHD 15sec, UEF 5 Sec)"=5.0, "Test Complete"=FALSE}, {"Sequence #"=16.0, "Cycles"=1, "Mode Setting"="", "Flow Rate (GPM)"=1.7, "Temperature (F)"=58.0, "Reset Timer"=FALSE, "Use Temp Decline Method"=FALSE, "Terminate Condition"=enum."C9-Do Nothing", "Condition Value #1"=0.0, "UE"=FALSE, "LE"=FALSE, "Comp"=FALSE, "Fan"=FALSE, "Test End Time (Sec)"=86400.0, "Purge Until Cutout"=FALSE, "Start Conditions"=enum."Every X (Seconds)", "Condition Value #2"=86400.0, "Remove Power"=TRUE, "Time"=68400.0, "Check Special Cond."=enum."SC1-Do Nothing", "Condition#"=enum."N/A", "Draw Flags"=enum."N/A", "Data Processing Delay (FHD 15sec, UEF 5 Sec)"=5.0, "Test Complete"=FALSE}] {"Time" format="%<%H:%M:%S>t"}
  in  "24HR Test - Standard":T21[](array[typedef])=[{"Sequence #"=1.0, "Cycles"=1, "Mode Setting"="", "Flow Rate (GPM)"=3.0, "Temperature (F)"=58.0, "Reset Timer"=FALSE, "Use Temp Decline Method"=FALSE, "Terminate Condition"=enum."C9-Do Nothing", "Condition Value #1"=0.0, "UE"=FALSE, "LE"=FALSE, "Comp"=FALSE, "Fan"=FALSE, "Test End Time (Sec)"=0.0, "Purge Until Cutout"=FALSE, "Start Conditions"=enum."Heat Source Cutout", "Condition Value #2"=0.0, "Remove Power"=FALSE, "Time"=82800.0, "Check Special Cond."=enum."SC1-Do Nothing", "Condition#"=enum."N/A", "Draw Flags"=enum."N/A", "Data Processing Delay (FHD 15sec, UEF 5 Sec)"=5.0, "Test Complete"=FALSE}, {"Sequence #"=2.0, "Cycles"=1, "Mode Setting"="", "Flow Rate (GPM)"=3.0, "Temperature (F)"=58.0, "Reset Timer"=TRUE, "Use Temp Decline Method"=TRUE, "Terminate Condition"=enum."C1-Terminate Draw @ Gallon Mark", "Condition Value #1"=10.72, "UE"=FALSE, "LE"=FALSE, "Comp"=FALSE, "Fan"=FALSE, "Test End Time (Sec)"=0.0, "Purge Until Cutout"=FALSE, "Start Conditions"=enum."At Time (Seconds)", "Condition Value #2"=0.0, "Remove Power"=FALSE, "Time"=82800.0, "Check Special Cond."=enum."SC1-Do Nothing", "Condition#"=enum."N/A", "Draw Flags"=enum."N/A", "Data Processing Delay (FHD 15sec, UEF 5 Sec)"=5.0, "Test Complete"=FALSE}, {"Sequence #"=3.0, "Cycles"=1, "Mode Setting"="", "Flow Rate (GPM)"=3.0, "Temperature (F)"=58.0, "Reset Timer"=FALSE, "Use Temp Decline Method"=FALSE, "Terminate Condition"=enum."C1-Terminate Draw @ Gallon Mark", "Condition Value #1"=10.72, "UE"=FALSE, "LE"=FALSE, "Comp"=FALSE, "Fan"=FALSE, "Test End Time (Sec)"=0.0, "Purge Until Cutout"=FALSE, "Start Conditions"=enum."At Time (Seconds)", "Condition Value #2"=3600.0, "Remove Power"=FALSE, "Time"=82800.0, "Check Special Cond."=enum."SC1-Do Nothing", "Condition#"=enum."N/A", "Draw Flags"=enum."N/A", "Data Processing Delay (FHD 15sec, UEF 5 Sec)"=5.0, "Test Complete"=FALSE}, {"Sequence #"=4.0, "Cycles"=1, "Mode Setting"="", "Flow Rate (GPM)"=3.0, "Temperature (F)"=58.0, "Reset Timer"=FALSE, "Use Temp Decline Method"=FALSE, "Terminate Condition"=enum."C1-Terminate Draw @ Gallon Mark", "Condition Value #1"=10.72, "UE"=FALSE, "LE"=FALSE, "Comp"=FALSE, "Fan"=FALSE, "Test End Time (Sec)"=0.0, "Purge Until Cutout"=FALSE, "Start Conditions"=enum."At Time (Seconds)", "Condition Value #2"=7200.0, "Remove Power"=FALSE, "Time"=82800.0, "Check Special Cond."=enum."SC1-Do Nothing", "Condition#"=enum."N/A", "Draw Flags"=enum."N/A", "Data Processing Delay (FHD 15sec, UEF 5 Sec)"=5.0, "Test Complete"=FALSE}, {"Sequence #"=5.0, "Cycles"=1, "Mode Setting"="", "Flow Rate (GPM)"=3.0, "Temperature (F)"=58.0, "Reset Timer"=FALSE, "Use Temp Decline Method"=FALSE, "Terminate Condition"=enum."C1-Terminate Draw @ Gallon Mark", "Condition Value #1"=10.72, "UE"=FALSE, "LE"=FALSE, "Comp"=FALSE, "Fan"=FALSE, "Test End Time (Sec)"=0.0, "Purge Until Cutout"=FALSE, "Start Conditions"=enum."At Time (Seconds)", "Condition Value #2"=10800.0, "Remove Power"=FALSE, "Time"=82800.0, "Check Special Cond."=enum."SC1-Do Nothing", "Condition#"=enum."N/A", "Draw Flags"=enum."N/A", "Data Processing Delay (FHD 15sec, UEF 5 Sec)"=5.0, "Test Complete"=FALSE}, {"Sequence #"=6.0, "Cycles"=1, "Mode Setting"="", "Flow Rate (GPM)"=3.0, "Temperature (F)"=58.0, "Reset Timer"=FALSE, "Use Temp Decline Method"=FALSE, "Terminate Condition"=enum."C1-Terminate Draw @ Gallon Mark", "Condition Value #1"=10.72, "UE"=FALSE, "LE"=FALSE, "Comp"=FALSE, "Fan"=FALSE, "Test End Time (Sec)"=0.0, "Purge Until Cutout"=FALSE, "Start Conditions"=enum."At Time (Seconds)", "Condition Value #2"=14400.0, "Remove Power"=FALSE, "Time"=82800.0, "Check Special Cond."=enum."SC1-Do Nothing", "Condition#"=enum."N/A", "Draw Flags"=enum."N/A", "Data Processing Delay (FHD 15sec, UEF 5 Sec)"=5.0, "Test Complete"=FALSE}, {"Sequence #"=7.0, "Cycles"=1, "Mode Setting"="", "Flow Rate (GPM)"=3.0, "Temperature (F)"=58.0, "Reset Timer"=FALSE, "Use Temp Decline Method"=FALSE, "Terminate Condition"=enum."C1-Terminate Draw @ Gallon Mark", "Condition Value #1"=10.72, "UE"=FALSE, "LE"=FALSE, "Comp"=FALSE, "Fan"=FALSE, "Test End Time (Sec)"=86400.0, "Purge Until Cutout"=FALSE, "Start Conditions"=enum."At Time (Seconds)", "Condition Value #2"=18000.0, "Remove Power"=TRUE, "Time"=82800.0, "Check Special Cond."=enum."SC1-Do Nothing", "Condition#"=enum."N/A", "Draw Flags"=enum."N/A", "Data Processing Delay (FHD 15sec, UEF 5 Sec)"=5.0, "Test Complete"=FALSE}] {"Time" format="%<%H:%M:%S>t"}
  in  "1st HR Test":T21[](array[typedef])=[{"Sequence #"=1.0, "Cycles"=1, "Mode Setting"="", "Flow Rate (GPM)"=3.0, "Temperature (F)"=58.0, "Reset Timer"=FALSE, "Use Temp Decline Method"=FALSE, "Terminate Condition"=enum."C7-Until Any Heat Source", "Condition Value #1"=0.0, "UE"=FALSE, "LE"=FALSE, "Comp"=FALSE, "Fan"=FALSE, "Test End Time (Sec)"=0.0, "Purge Until Cutout"=FALSE, "Start Conditions"=enum."Heat Source Cutout", "Condition Value #2"=0.0, "Remove Power"=FALSE, "Time"=3600.0, "Check Special Cond."=enum."SC1-Do Nothing", "Condition#"=enum."N/A", "Draw Flags"=enum."N/A", "Data Processing Delay (FHD 15sec, UEF 5 Sec)"=15.0, "Test Complete"=FALSE}, {"Sequence #"=2.0, "Cycles"=1, "Mode Setting"="", "Flow Rate (GPM)"=3.0, "Temperature (F)"=58.0, "Reset Timer"=TRUE, "Use Temp Decline Method"=TRUE, "Terminate Condition"=enum."C5-Decrease RTD Out (Deg F)", "Condition Value #1"=15.0, "UE"=FALSE, "LE"=FALSE, "Comp"=FALSE, "Fan"=FALSE, "Test End Time (Sec)"=0.0, "Purge Until Cutout"=FALSE, "Start Conditions"=enum."Heat Source Cutout", "Condition Value #2"=0.0, "Remove Power"=FALSE, "Time"=3600.0, "Check Special Cond."=enum."SC1-Do Nothing", "Condition#"=enum."N/A", "Draw Flags"=enum."N/A", "Data Processing Delay (FHD 15sec, UEF 5 Sec)"=15.0, "Test Complete"=FALSE}, {"Sequence #"=3.0, "Cycles"=5, "Mode Setting"="", "Flow Rate (GPM)"=3.0, "Temperature (F)"=58.0, "Reset Timer"=FALSE, "Use Temp Decline Method"=FALSE, "Terminate Condition"=enum."C5-Decrease RTD Out (Deg F)", "Condition Value #1"=15.0, "UE"=TRUE, "LE"=TRUE, "Comp"=FALSE, "Fan"=FALSE, "Test End Time (Sec)"=0.0, "Purge Until Cutout"=TRUE, "Start Conditions"=enum."T2 >= X° Below Setpoint", "Condition Value #2"=8.0, "Remove Power"=FALSE, "Time"=3600.0, "Check Special Cond."=enum."SC1-Do Nothing", "Condition#"=enum."N/A", "Draw Flags"=enum."N/A", "Data Processing Delay (FHD 15sec, UEF 5 Sec)"=15.0, "Test Complete"=FALSE}, {"Sequence #"=4.0, "Cycles"=1, "Mode Setting"="", "Flow Rate (GPM)"=3.0, "Temperature (F)"=58.0, "Reset Timer"=FALSE, "Use Temp Decline Method"=FALSE, "Terminate Condition"=enum."C2-Special Last Draw (HU Test)", "Condition Value #1"=0.0, "UE"=FALSE, "LE"=FALSE, "Comp"=FALSE, "Fan"=FALSE, "Test End Time (Sec)"=3600.0, "Purge Until Cutout"=TRUE, "Start Conditions"=enum."Seconds From Complete", "Condition Value #2"=180.0, "Remove Power"=TRUE, "Time"=3600.0, "Check Special Cond."=enum."SC1-Do Nothing", "Condition#"=enum."N/A", "Draw Flags"=enum."N/A", "Data Processing Delay (FHD 15sec, UEF 5 Sec)"=15.0, "Test Complete"=FALSE}] {"Time" format="%<%H:%M:%S>t"}
  in  "24HR Test - High Usage":T21[](array[typedef])=[{"Sequence #"=1.0, "Cycles"=1, "Mode Setting"="", "Flow Rate (GPM)"=3.0, "Temperature (F)"=58.0, "Reset Timer"=FALSE, "Use Temp Decline Method"=FALSE, "Terminate Condition"=enum."C9-Do Nothing", "Condition Value #1"=0.0, "UE"=FALSE, "LE"=FALSE, "Comp"=FALSE, "Fan"=FALSE, "Test End Time (Sec)"=0.0, "Purge Until Cutout"=FALSE, "Start Conditions"=enum."Heat Source Cutout", "Condition Value #2"=0.0, "Remove Power"=FALSE, "Time"=82800.0, "Check Special Cond."=enum."SC1-Do Nothing", "Condition#"=enum."N/A", "Draw Flags"=enum."N/A", "Data Processing Delay (FHD 15sec, UEF 5 Sec)"=0.0, "Test Complete"=FALSE}, {"Sequence #"=2.0, "Cycles"=1, "Mode Setting"="", "Flow Rate (GPM)"=3.0, "Temperature (F)"=58.0, "Reset Timer"=FALSE, "Use Temp Decline Method"=FALSE, "Terminate Condition"=enum."C9-Do Nothing", "Condition Value #1"=0.0, "UE"=FALSE, "LE"=FALSE, "Comp"=FALSE, "Fan"=FALSE, "Test End Time (Sec)"=0.0, "Purge Until Cutout"=FALSE, "Start Conditions"=enum."Heat Source Cutout", "Condition Value #2"=0.0, "Remove Power"=FALSE, "Time"=82800.0, "Check Special Cond."=enum."SC1-Do Nothing", "Condition#"=enum."N/A", "Draw Flags"=enum."N/A", "Data Processing Delay (FHD 15sec, UEF 5 Sec)"=0.0, "Test Complete"=FALSE}, {"Sequence #"=3.0, "Cycles"=1, "Mode Setting"="", "Flow Rate (GPM)"=3.0, "Temperature (F)"=58.0, "Reset Timer"=FALSE, "Use Temp Decline Method"=FALSE, "Terminate Condition"=enum."C9-Do Nothing", "Condition Value #1"=0.0, "UE"=FALSE, "LE"=FALSE, "Comp"=FALSE, "Fan"=FALSE, "Test End Time (Sec)"=0.0, "Purge Until Cutout"=FALSE, "Start Conditions"=enum."Every X (Seconds)", "Condition Value #2"=3600.0, "Remove Power"=FALSE, "Time"=82800.0, "Check Special Cond."=enum."SC1-Do Nothing", "Condition#"=enum."N/A", "Draw Flags"=enum."N/A", "Data Processing Delay (FHD 15sec, UEF 5 Sec)"=0.0, "Test Complete"=FALSE}, {"Sequence #"=4.0, "Cycles"=1, "Mode Setting"="", "Flow Rate (GPM)"=3.0, "Temperature (F)"=58.0, "Reset Timer"=TRUE, "Use Temp Decline Method"=TRUE, "Terminate Condition"=enum."C1-Terminate Draw @ Gallon Mark", "Condition Value #1"=27.0, "UE"=FALSE, "LE"=FALSE, "Comp"=FALSE, "Fan"=FALSE, "Test End Time (Sec)"=0.0, "Purge Until Cutout"=FALSE, "Start Conditions"=enum."At Time (Seconds)", "Condition Value #2"=0.0, "Remove Power"=FALSE, "Time"=82800.0, "Check Special Cond."=enum."SC1-Do Nothing", "Condition#"=enum."N/A", "Draw Flags"=enum."N/A", "Data Processing Delay (FHD 15sec, UEF 5 Sec)"=0.0, "Test Complete"=FALSE}, {"Sequence #"=5.0, "Cycles"=1, "Mode Setting"="", "Flow Rate (GPM)"=1.0, "Temperature (F)"=58.0, "Reset Timer"=FALSE, "Use Temp Decline Method"=FALSE, "Terminate Condition"=enum."C1-Terminate Draw @ Gallon Mark", "Condition Value #1"=2.0, "UE"=FALSE, "LE"=FALSE, "Comp"=FALSE, "Fan"=FALSE, "Test End Time (Sec)"=0.0, "Purge Until Cutout"=FALSE, "Start Conditions"=enum."At Time (Seconds)", "Condition Value #2"=1800.0, "Remove Power"=FALSE, "Time"=82800.0, "Check Special Cond."=enum."SC1-Do Nothing", "Condition#"=enum."N/A", "Draw Flags"=enum."N/A", "Data Processing Delay (FHD 15sec, UEF 5 Sec)"=0.0, "Test Complete"=FALSE}, {"Sequence #"=6.0, "Cycles"=1, "Mode Setting"="", "Flow Rate (GPM)"=1.0, "Temperature (F)"=58.0, "Reset Timer"=FALSE, "Use Temp Decline Method"=FALSE, "Terminate Condition"=enum."C1-Terminate Draw @ Gallon Mark", "Condition Value #1"=1.0, "UE"=FALSE, "LE"=FALSE, "Comp"=FALSE, "Fan"=FALSE, "Test End Time (Sec)"=0.0, "Purge Until Cutout"=FALSE, "Start Conditions"=enum."At Time (Seconds)", "Condition Value #2"=2400.0, "Remove Power"=FALSE, "Time"=82800.0, "Check Special Cond."=enum."SC1-Do Nothing", "Condition#"=enum."N/A", "Draw Flags"=enum."N/A", "Data Processing Delay (FHD 15sec, UEF 5 Sec)"=0.0, "Test Complete"=FALSE}, {"Sequence #"=7.0, "Cycles"=1, "Mode Setting"="", "Flow Rate (GPM)"=1.7, "Temperature (F)"=58.0, "Reset Timer"=FALSE, "Use Temp Decline Method"=FALSE, "Terminate Condition"=enum."C1-Terminate Draw @ Gallon Mark", "Condition Value #1"=9.0, "UE"=FALSE, "LE"=FALSE, "Comp"=FALSE, "Fan"=FALSE, "Test End Time (Sec)"=0.0, "Purge Until Cutout"=FALSE, "Start Conditions"=enum."At Time (Seconds)", "Condition Value #2"=6000.0, "Remove Power"=FALSE, "Time"=82800.0, "Check Special Cond."=enum."SC1-Do Nothing", "Condition#"=enum."N/A", "Draw Flags"=enum."N/A", "Data Processing Delay (FHD 15sec, UEF 5 Sec)"=0.0, "Test Complete"=FALSE}, {"Sequence #"=8.0, "Cycles"=1, "Mode Setting"="", "Flow Rate (GPM)"=3.0, "Temperature (F)"=58.0, "Reset Timer"=FALSE, "Use Temp Decline Method"=FALSE, "Terminate Condition"=enum."C1-Terminate Draw @ Gallon Mark", "Condition Value #1"=15.0, "UE"=FALSE, "LE"=FALSE, "Comp"=FALSE, "Fan"=FALSE, "Test End Time (Sec)"=0.0, "Purge Until Cutout"=FALSE, "Start Conditions"=enum."At Time (Seconds)", "Condition Value #2"=37800.0, "Remove Power"=FALSE, "Time"=82800.0, "Check Special Cond."=enum."SC1-Do Nothing", "Condition#"=enum."N/A", "Draw Flags"=enum."N/A", "Data Processing Delay (FHD 15sec, UEF 5 Sec)"=0.0, "Test Complete"=FALSE}, {"Sequence #"=9.0, "Cycles"=1, "Mode Setting"="", "Flow Rate (GPM)"=1.7, "Temperature (F)"=58.0, "Reset Timer"=FALSE, "Use Temp Decline Method"=FALSE, "Terminate Condition"=enum."C1-Terminate Draw @ Gallon Mark", "Condition Value #1"=5.0, "UE"=FALSE, "LE"=FALSE, "Comp"=FALSE, "Fan"=FALSE, "Test End Time (Sec)"=0.0, "Purge Until Cutout"=FALSE, "Start Conditions"=enum."At Time (Seconds)", "Condition Value #2"=41400.0, "Remove Power"=FALSE, "Time"=82800.0, "Check Special Cond."=enum."SC1-Do Nothing", "Condition#"=enum."N/A", "Draw Flags"=enum."N/A", "Data Processing Delay (FHD 15sec, UEF 5 Sec)"=0.0, "Test Complete"=FALSE}, {"Sequence #"=10.0, "Cycles"=1, "Mode Setting"="", "Flow Rate (GPM)"=1.0, "Temperature (F)"=58.0, "Reset Timer"=FALSE, "Use Temp Decline Method"=FALSE, "Terminate Condition"=enum."C1-Terminate Draw @ Gallon Mark", "Condition Value #1"=1.0, "UE"=FALSE, "LE"=FALSE, "Comp"=FALSE, "Fan"=FALSE, "Test End Time (Sec)"=0.0, "Purge Until Cutout"=FALSE, "Start Conditions"=enum."At Time (Seconds)", "Condition Value #2"=43200.0, "Remove Power"=FALSE, "Time"=82800.0, "Check Special Cond."=enum."SC1-Do Nothing", "Condition#"=enum."N/A", "Draw Flags"=enum."N/A", "Data Processing Delay (FHD 15sec, UEF 5 Sec)"=0.0, "Test Complete"=FALSE}, {"Sequence #"=11.0, "Cycles"=1, "Mode Setting"="", "Flow Rate (GPM)"=1.0, "Temperature (F)"=58.0, "Reset Timer"=FALSE, "Use Temp Decline Method"=FALSE, "Terminate Condition"=enum."C1-Terminate Draw @ Gallon Mark", "Condition Value #1"=1.0, "UE"=FALSE, "LE"=FALSE, "Comp"=FALSE, "Fan"=FALSE, "Test End Time (Sec)"=0.0, "Purge Until Cutout"=FALSE, "Start Conditions"=enum."At Time (Seconds)", "Condition Value #2"=45900.0, "Remove Power"=FALSE, "Time"=82800.0, "Check Special Cond."=enum."SC1-Do Nothing", "Condition#"=enum."N/A", "Draw Flags"=enum."N/A", "Data Processing Delay (FHD 15sec, UEF 5 Sec)"=0.0, "Test Complete"=FALSE}, {"Sequence #"=12.0, "Cycles"=1, "Mode Setting"="", "Flow Rate (GPM)"=1.0, "Temperature (F)"=58.0, "Reset Timer"=FALSE, "Use Temp Decline Method"=FALSE, "Terminate Condition"=enum."C1-Terminate Draw @ Gallon Mark", "Condition Value #1"=1.0, "UE"=FALSE, "LE"=FALSE, "Comp"=FALSE, "Fan"=FALSE, "Test End Time (Sec)"=0.0, "Purge Until Cutout"=FALSE, "Start Conditions"=enum."At Time (Seconds)", "Condition Value #2"=46200.0, "Remove Power"=FALSE, "Time"=82800.0, "Check Special Cond."=enum."SC1-Do Nothing", "Condition#"=enum."N/A", "Draw Flags"=enum."N/A", "Data Processing Delay (FHD 15sec, UEF 5 Sec)"=0.0, "Test Complete"=FALSE}, {"Sequence #"=13.0, "Cycles"=1, "Mode Setting"="", "Flow Rate (GPM)"=1.0, "Temperature (F)"=58.0, "Reset Timer"=FALSE, "Use Temp Decline Method"=FALSE, "Terminate Condition"=enum."C1-Terminate Draw @ Gallon Mark", "Condition Value #1"=2.0, "UE"=FALSE, "LE"=FALSE, "Comp"=FALSE, "Fan"=FALSE, "Test End Time (Sec)"=0.0, "Purge Until Cutout"=FALSE, "Start Conditions"=enum."At Time (Seconds)", "Condition Value #2"=57600.0, "Remove Power"=FALSE, "Time"=82800.0, "Check Special Cond."=enum."SC1-Do Nothing", "Condition#"=enum."N/A", "Draw Flags"=enum."N/A", "Data Processing Delay (FHD 15sec, UEF 5 Sec)"=0.0, "Test Complete"=FALSE}, {"Sequence #"=14.0, "Cycles"=1, "Mode Setting"="", "Flow Rate (GPM)"=1.0, "Temperature (F)"=58.0, "Reset Timer"=FALSE, "Use Temp Decline Method"=FALSE, "Terminate Condition"=enum."C1-Terminate Draw @ Gallon Mark", "Condition Value #1"=2.0, "UE"=FALSE, "LE"=FALSE, "Comp"=FALSE, "Fan"=FALSE, "Test End Time (Sec)"=0.0, "Purge Until Cutout"=FALSE, "Start Conditions"=enum."At Time (Seconds)", "Condition Value #2"=58500.0, "Remove Power"=FALSE, "Time"=82800.0, "Check Special Cond."=enum."SC1-Do Nothing", "Condition#"=enum."N/A", "Draw Flags"=enum."N/A", "Data Processing Delay (FHD 15sec, UEF 5 Sec)"=0.0, "Test Complete"=FALSE}, {"Sequence #"=15.0, "Cycles"=1, "Mode Setting"="", "Flow Rate (GPM)"=1.7, "Temperature (F)"=58.0, "Reset Timer"=FALSE, "Use Temp Decline Method"=FALSE, "Terminate Condition"=enum."C1-Terminate Draw @ Gallon Mark", "Condition Value #1"=2.0, "UE"=FALSE, "LE"=FALSE, "Comp"=FALSE, "Fan"=FALSE, "Test End Time (Sec)"=0.0, "Purge Until Cutout"=FALSE, "Start Conditions"=enum."At Time (Seconds)", "Condition Value #2"=59400.0, "Remove Power"=FALSE, "Time"=82800.0, "Check Special Cond."=enum."SC1-Do Nothing", "Condition#"=enum."N/A", "Draw Flags"=enum."N/A", "Data Processing Delay (FHD 15sec, UEF 5 Sec)"=0.0, "Test Complete"=FALSE}, {"Sequence #"=16.0, "Cycles"=1, "Mode Setting"="", "Flow Rate (GPM)"=1.7, "Temperature (F)"=58.0, "Reset Timer"=FALSE, "Use Temp Decline Method"=FALSE, "Terminate Condition"=enum."C1-Terminate Draw @ Gallon Mark", "Condition Value #1"=2.0, "UE"=FALSE, "LE"=FALSE, "Comp"=FALSE, "Fan"=FALSE, "Test End Time (Sec)"=0.0, "Purge Until Cutout"=FALSE, "Start Conditions"=enum."At Time (Seconds)", "Condition Value #2"=60300.0, "Remove Power"=FALSE, "Time"=82800.0, "Check Special Cond."=enum."SC1-Do Nothing", "Condition#"=enum."N/A", "Draw Flags"=enum."N/A", "Data Processing Delay (FHD 15sec, UEF 5 Sec)"=0.0, "Test Complete"=FALSE}, {"Sequence #"=17.0, "Cycles"=1, "Mode Setting"="", "Flow Rate (GPM)"=3.0, "Temperature (F)"=58.0, "Reset Timer"=FALSE, "Use Temp Decline Method"=FALSE, "Terminate Condition"=enum."C1-Terminate Draw @ Gallon Mark", "Condition Value #1"=14.0, "UE"=FALSE, "LE"=FALSE, "Comp"=FALSE, "Fan"=FALSE, "Test End Time (Sec)"=86400.0, "Purge Until Cutout"=FALSE, "Start Conditions"=enum."At Time (Seconds)", "Condition Value #2"=61200.0, "Remove Power"=TRUE, "Time"=82800.0, "Check Special Cond."=enum."SC1-Do Nothing", "Condition#"=enum."N/A", "Draw Flags"=enum."N/A", "Data Processing Delay (FHD 15sec, UEF 5 Sec)"=0.0, "Test Complete"=FALSE}] {"Time" format="%<%H:%M:%S>t"}
  in  "24HR Test - Medium Usage":T21[](array[typedef])=[{"Sequence #"=1.0, "Cycles"=1, "Mode Setting"="", "Flow Rate (GPM)"=3.0, "Temperature (F)"=58.0, "Reset Timer"=FALSE, "Use Temp Decline Method"=FALSE, "Terminate Condition"=enum."C9-Do Nothing", "Condition Value #1"=0.0, "UE"=FALSE, "LE"=FALSE, "Comp"=FALSE, "Fan"=FALSE, "Test End Time (Sec)"=0.0, "Purge Until Cutout"=FALSE, "Start Conditions"=enum."Heat Source Cutout", "Condition Value #2"=0.0, "Remove Power"=FALSE, "Time"=82800.0, "Check Special Cond."=enum."SC1-Do Nothing", "Condition#"=enum."N/A", "Draw Flags"=enum."N/A", "Data Processing Delay (FHD 15sec, UEF 5 Sec)"=0.0, "Test Complete"=FALSE}, {"Sequence #"=2.0, "Cycles"=1, "Mode Setting"="", "Flow Rate (GPM)"=3.0, "Temperature (F)"=58.0, "Reset Timer"=FALSE, "Use Temp Decline Method"=FALSE, "Terminate Condition"=enum."C9-Do Nothing", "Condition Value #1"=0.0, "UE"=FALSE, "LE"=FALSE, "Comp"=FALSE, "Fan"=FALSE, "Test End Time (Sec)"=0.0, "Purge Until Cutout"=FALSE, "Start Conditions"=enum."Heat Source Cutout", "Condition Value #2"=0.0, "Remove Power"=FALSE, "Time"=82800.0, "Check Special Cond."=enum."SC1-Do Nothing", "Condition#"=enum."N/A", "Draw Flags"=enum."N/A", "Data Processing Delay (FHD 15sec, UEF 5 Sec)"=0.0, "Test Complete"=FALSE}, {"Sequence #"=3.0, "Cycles"=1, "Mode Setting"="", "Flow Rate (GPM)"=3.0, "Temperature (F)"=58.0, "Reset Timer"=FALSE, "Use Temp Decline Method"=FALSE, "Terminate Condition"=enum."C9-Do Nothing", "Condition Value #1"=0.0, "UE"=FALSE, "LE"=FALSE, "Comp"=FALSE, "Fan"=FALSE, "Test End Time (Sec)"=0.0, "Purge Until Cutout"=FALSE, "Start Conditions"=enum."Every X (Seconds)", "Condition Value #2"=3600.0, "Remove Power"=FALSE, "Time"=82800.0, "Check Special Cond."=enum."SC1-Do Nothing", "Condition#"=enum."N/A", "Draw Flags"=enum."N/A", "Data Processing Delay (FHD 15sec, UEF 5 Sec)"=0.0, "Test Complete"=FALSE}, {"Sequence #"=4.0, "Cycles"=1, "Mode Setting"="", "Flow Rate (GPM)"=1.7, "Temperature (F)"=58.0, "Reset Timer"=TRUE, "Use Temp Decline Method"=TRUE, "Terminate Condition"=enum."C1-Terminate Draw @ Gallon Mark", "Condition Value #1"=15.0, "UE"=FALSE, "LE"=FALSE, "Comp"=FALSE, "Fan"=FALSE, "Test End Time (Sec)"=0.0, "Purge Until Cutout"=FALSE, "Start Conditions"=enum."At Time (Seconds)", "Condition Value #2"=0.0, "Remove Power"=FALSE, "Time"=82800.0, "Check Special Cond."=enum."SC1-Do Nothing", "Condition#"=enum."N/A", "Draw Flags"=enum."N/A", "Data Processing Delay (FHD 15sec, UEF 5 Sec)"=0.0, "Test Complete"=FALSE}, {"Sequence #"=5.0, "Cycles"=1, "Mode Setting"="", "Flow Rate (GPM)"=1.0, "Temperature (F)"=58.0, "Reset Timer"=FALSE, "Use Temp Decline Method"=FALSE, "Terminate Condition"=enum."C1-Terminate Draw @ Gallon Mark", "Condition Value #1"=2.0, "UE"=FALSE, "LE"=FALSE, "Comp"=FALSE, "Fan"=FALSE, "Test End Time (Sec)"=0.0, "Purge Until Cutout"=FALSE, "Start Conditions"=enum."At Time (Seconds)", "Condition Value #2"=1800.0, "Remove Power"=FALSE, "Time"=82800.0, "Check Special Cond."=enum."SC1-Do Nothing", "Condition#"=enum."N/A", "Draw Flags"=enum."N/A", "Data Processing Delay (FHD 15sec, UEF 5 Sec)"=0.0, "Test Complete"=FALSE}, {"Sequence #"=6.0, "Cycles"=1, "Mode Setting"="", "Flow Rate (GPM)"=1.7, "Temperature (F)"=58.0, "Reset Timer"=FALSE, "Use Temp Decline Method"=FALSE, "Terminate Condition"=enum."C1-Terminate Draw @ Gallon Mark", "Condition Value #1"=9.0, "UE"=FALSE, "LE"=FALSE, "Comp"=FALSE, "Fan"=FALSE, "Test End Time (Sec)"=0.0, "Purge Until Cutout"=FALSE, "Start Conditions"=enum."At Time (Seconds)", "Condition Value #2"=6000.0, "Remove Power"=FALSE, "Time"=82800.0, "Check Special Cond."=enum."SC1-Do Nothing", "Condition#"=enum."N/A", "Draw Flags"=enum."N/A", "Data Processing Delay (FHD 15sec, UEF 5 Sec)"=0.0, "Test Complete"=FALSE}, {"Sequence #"=7.0, "Cycles"=1, "Mode Setting"="", "Flow Rate (GPM)"=1.7, "Temperature (F)"=58.0, "Reset Timer"=FALSE, "Use Temp Decline Method"=FALSE, "Terminate Condition"=enum."C1-Terminate Draw @ Gallon Mark", "Condition Value #1"=9.0, "UE"=FALSE, "LE"=FALSE, "Comp"=FALSE, "Fan"=FALSE, "Test End Time (Sec)"=0.0, "Purge Until Cutout"=FALSE, "Start Conditions"=enum."At Time (Seconds)", "Condition Value #2"=37800.0, "Remove Power"=FALSE, "Time"=82800.0, "Check Special Cond."=enum."SC1-Do Nothing", "Condition#"=enum."N/A", "Draw Flags"=enum."N/A", "Data Processing Delay (FHD 15sec, UEF 5 Sec)"=0.0, "Test Complete"=FALSE}, {"Sequence #"=8.0, "Cycles"=1, "Mode Setting"="", "Flow Rate (GPM)"=1.7, "Temperature (F)"=58.0, "Reset Timer"=FALSE, "Use Temp Decline Method"=FALSE, "Terminate Condition"=enum."C1-Terminate Draw @ Gallon Mark", "Condition Value #1"=5.0, "UE"=FALSE, "LE"=FALSE, "Comp"=FALSE, "Fan"=FALSE, "Test End Time (Sec)"=0.0, "Purge Until Cutout"=FALSE, "Start Conditions"=enum."At Time (Seconds)", "Condition Value #2"=41400.0, "Remove Power"=FALSE, "Time"=82800.0, "Check Special Cond."=enum."SC1-Do Nothing", "Condition#"=enum."N/A", "Draw Flags"=enum."N/A", "Data Processing Delay (FHD 15sec, UEF 5 Sec)"=0.0, "Test Complete"=FALSE}, {"Sequence #"=9.0, "Cycles"=1, "Mode Setting"="", "Flow Rate (GPM)"=1.0, "Temperature (F)"=58.0, "Reset Timer"=FALSE, "Use Temp Decline Method"=FALSE, "Terminate Condition"=enum."C1-Terminate Draw @ Gallon Mark", "Condition Value #1"=1.0, "UE"=FALSE, "LE"=FALSE, "Comp"=FALSE, "Fan"=FALSE, "Test End Time (Sec)"=0.0, "Purge Until Cutout"=FALSE, "Start Conditions"=enum."At Time (Seconds)", "Condition Value #2"=43200.0, "Remove Power"=FALSE, "Time"=82800.0, "Check Special Cond."=enum."SC1-Do Nothing", "Condition#"=enum."N/A", "Draw Flags"=enum."N/A", "Data Processing Delay (FHD 15sec, UEF 5 Sec)"=0.0, "Test Complete"=FALSE}, {"Sequence #"=10.0, "Cycles"=1, "Mode Setting"="", "Flow Rate (GPM)"=1.0, "Temperature (F)"=58.0, "Reset Timer"=FALSE, "Use Temp Decline Method"=FALSE, "Terminate Condition"=enum."C1-Terminate Draw @ Gallon Mark", "Condition Value #1"=1.0, "UE"=FALSE, "LE"=FALSE, "Comp"=FALSE, "Fan"=FALSE, "Test End Time (Sec)"=0.0, "Purge Until Cutout"=FALSE, "Start Conditions"=enum."At Time (Seconds)", "Condition Value #2"=45900.0, "Remove Power"=FALSE, "Time"=82800.0, "Check Special Cond."=enum."SC1-Do Nothing", "Condition#"=enum."N/A", "Draw Flags"=enum."N/A", "Data Processing Delay (FHD 15sec, UEF 5 Sec)"=0.0, "Test Complete"=FALSE}, {"Sequence #"=11.0, "Cycles"=1, "Mode Setting"="", "Flow Rate (GPM)"=1.0, "Temperature (F)"=58.0, "Reset Timer"=FALSE, "Use Temp Decline Method"=FALSE, "Terminate Condition"=enum."C1-Terminate Draw @ Gallon Mark", "Condition Value #1"=1.0, "UE"=FALSE, "LE"=FALSE, "Comp"=FALSE, "Fan"=FALSE, "Test End Time (Sec)"=0.0, "Purge Until Cutout"=FALSE, "Start Conditions"=enum."At Time (Seconds)", "Condition Value #2"=46200.0, "Remove Power"=FALSE, "Time"=82800.0, "Check Special Cond."=enum."SC1-Do Nothing", "Condition#"=enum."N/A", "Draw Flags"=enum."N/A", "Data Processing Delay (FHD 15sec, UEF 5 Sec)"=0.0, "Test Complete"=FALSE}, {"Sequence #"=12.0, "Cycles"=1, "Mode Setting"="", "Flow Rate (GPM)"=1.0, "Temperature (F)"=58.0, "Reset Timer"=FALSE, "Use Temp Decline Method"=FALSE, "Terminate Condition"=enum."C1-Terminate Draw @ Gallon Mark", "Condition Value #1"=1.0, "UE"=FALSE, "LE"=FALSE, "Comp"=FALSE, "Fan"=FALSE, "Test End Time (Sec)"=0.0, "Purge Until Cutout"=FALSE, "Start Conditions"=enum."At Time (Seconds)", "Condition Value #2"=57600.0, "Remove Power"=FALSE, "Time"=82800.0, "Check Special Cond."=enum."SC1-Do Nothing", "Condition#"=enum."N/A", "Draw Flags"=enum."N/A", "Data Processing Delay (FHD 15sec, UEF 5 Sec)"=0.0, "Test Complete"=FALSE}, {"Sequence #"=13.0, "Cycles"=1, "Mode Setting"="", "Flow Rate (GPM)"=1.0, "Temperature (F)"=58.0, "Reset Timer"=FALSE, "Use Temp Decline Method"=FALSE, "Terminate Condition"=enum."C1-Terminate Draw @ Gallon Mark", "Condition Value #1"=2.0, "UE"=FALSE, "LE"=FALSE, "Comp"=FALSE, "Fan"=FALSE, "Test End Time (Sec)"=0.0, "Purge Until Cutout"=FALSE, "Start Conditions"=enum."At Time (Seconds)", "Condition Value #2"=58500.0, "Remove Power"=FALSE, "Time"=82800.0, "Check Special Cond."=enum."SC1-Do Nothing", "Condition#"=enum."N/A", "Draw Flags"=enum."N/A", "Data Processing Delay (FHD 15sec, UEF 5 Sec)"=0.0, "Test Complete"=FALSE}, {"Sequence #"=14.0, "Cycles"=1, "Mode Setting"="", "Flow Rate (GPM)"=1.7, "Temperature (F)"=58.0, "Reset Timer"=FALSE, "Use Temp Decline Method"=FALSE, "Terminate Condition"=enum."C1-Terminate Draw @ Gallon Mark", "Condition Value #1"=2.0, "UE"=FALSE, "LE"=FALSE, "Comp"=FALSE, "Fan"=FALSE, "Test End Time (Sec)"=0.0, "Purge Until Cutout"=FALSE, "Start Conditions"=enum."At Time (Seconds)", "Condition Value #2"=60300.0, "Remove Power"=FALSE, "Time"=82800.0, "Check Special Cond."=enum."SC1-Do Nothing", "Condition#"=enum."N/A", "Draw Flags"=enum."N/A", "Data Processing Delay (FHD 15sec, UEF 5 Sec)"=0.0, "Test Complete"=FALSE}, {"Sequence #"=15.0, "Cycles"=1, "Mode Setting"="", "Flow Rate (GPM)"=1.7, "Temperature (F)"=58.0, "Reset Timer"=FALSE, "Use Temp Decline Method"=FALSE, "Terminate Condition"=enum."C1-Terminate Draw @ Gallon Mark", "Condition Value #1"=7.0, "UE"=FALSE, "LE"=FALSE, "Comp"=FALSE, "Fan"=FALSE, "Test End Time (Sec)"=86400.0, "Purge Until Cutout"=FALSE, "Start Conditions"=enum."At Time (Seconds)", "Condition Value #2"=61200.0, "Remove Power"=TRUE, "Time"=82800.0, "Check Special Cond."=enum."SC1-Do Nothing", "Condition#"=enum."N/A", "Draw Flags"=enum."N/A", "Data Processing Delay (FHD 15sec, UEF 5 Sec)"=0.0, "Test Complete"=FALSE}] {"Time" format="%<%H:%M:%S>t"}
  in  "24HR Test - Low Usage":T21[](array[typedef])=[{"Sequence #"=1.0, "Cycles"=1, "Mode Setting"="", "Flow Rate (GPM)"=3.0, "Temperature (F)"=58.0, "Reset Timer"=FALSE, "Use Temp Decline Method"=FALSE, "Terminate Condition"=enum."C9-Do Nothing", "Condition Value #1"=0.0, "UE"=FALSE, "LE"=FALSE, "Comp"=FALSE, "Fan"=FALSE, "Test End Time (Sec)"=0.0, "Purge Until Cutout"=FALSE, "Start Conditions"=enum."Heat Source Cutout", "Condition Value #2"=0.0, "Remove Power"=FALSE, "Time"=82800.0, "Check Special Cond."=enum."SC1-Do Nothing", "Condition#"=enum."N/A", "Draw Flags"=enum."N/A", "Data Processing Delay (FHD 15sec, UEF 5 Sec)"=0.0, "Test Complete"=FALSE}, {"Sequence #"=2.0, "Cycles"=1, "Mode Setting"="", "Flow Rate (GPM)"=3.0, "Temperature (F)"=58.0, "Reset Timer"=FALSE, "Use Temp Decline Method"=FALSE, "Terminate Condition"=enum."C9-Do Nothing", "Condition Value #1"=0.0, "UE"=FALSE, "LE"=FALSE, "Comp"=FALSE, "Fan"=FALSE, "Test End Time (Sec)"=0.0, "Purge Until Cutout"=FALSE, "Start Conditions"=enum."Heat Source Cutout", "Condition Value #2"=0.0, "Remove Power"=FALSE, "Time"=82800.0, "Check Special Cond."=enum."SC1-Do Nothing", "Condition#"=enum."N/A", "Draw Flags"=enum."N/A", "Data Processing Delay (FHD 15sec, UEF 5 Sec)"=0.0, "Test Complete"=FALSE}, {"Sequence #"=3.0, "Cycles"=1, "Mode Setting"="", "Flow Rate (GPM)"=3.0, "Temperature (F)"=58.0, "Reset Timer"=FALSE, "Use Temp Decline Method"=FALSE, "Terminate Condition"=enum."C9-Do Nothing", "Condition Value #1"=0.0, "UE"=FALSE, "LE"=FALSE, "Comp"=FALSE, "Fan"=FALSE, "Test End Time (Sec)"=0.0, "Purge Until Cutout"=FALSE, "Start Conditions"=enum."Every X (Seconds)", "Condition Value #2"=3600.0, "Remove Power"=FALSE, "Time"=82800.0, "Check Special Cond."=enum."SC1-Do Nothing", "Condition#"=enum."N/A", "Draw Flags"=enum."N/A", "Data Processing Delay (FHD 15sec, UEF 5 Sec)"=0.0, "Test Complete"=FALSE}, {"Sequence #"=4.0, "Cycles"=1, "Mode Setting"="", "Flow Rate (GPM)"=1.7, "Temperature (F)"=58.0, "Reset Timer"=TRUE, "Use Temp Decline Method"=TRUE, "Terminate Condition"=enum."C1-Terminate Draw @ Gallon Mark", "Condition Value #1"=15.0, "UE"=FALSE, "LE"=FALSE, "Comp"=FALSE, "Fan"=FALSE, "Test End Time (Sec)"=0.0, "Purge Until Cutout"=FALSE, "Start Conditions"=enum."At Time (Seconds)", "Condition Value #2"=0.0, "Remove Power"=FALSE, "Time"=82800.0, "Check Special Cond."=enum."SC1-Do Nothing", "Condition#"=enum."N/A", "Draw Flags"=enum."N/A", "Data Processing Delay (FHD 15sec, UEF 5 Sec)"=0.0, "Test Complete"=FALSE}, {"Sequence #"=5.0, "Cycles"=1, "Mode Setting"="", "Flow Rate (GPM)"=1.0, "Temperature (F)"=58.0, "Reset Timer"=FALSE, "Use Temp Decline Method"=FALSE, "Terminate Condition"=enum."C1-Terminate Draw @ Gallon Mark", "Condition Value #1"=2.0, "UE"=FALSE, "LE"=FALSE, "Comp"=FALSE, "Fan"=FALSE, "Test End Time (Sec)"=0.0, "Purge Until Cutout"=FALSE, "Start Conditions"=enum."At Time (Seconds)", "Condition Value #2"=1800.0, "Remove Power"=FALSE, "Time"=82800.0, "Check Special Cond."=enum."SC1-Do Nothing", "Condition#"=enum."N/A", "Draw Flags"=enum."N/A", "Data Processing Delay (FHD 15sec, UEF 5 Sec)"=0.0, "Test Complete"=FALSE}, {"Sequence #"=6.0, "Cycles"=1, "Mode Setting"="", "Flow Rate (GPM)"=1.0, "Temperature (F)"=58.0, "Reset Timer"=FALSE, "Use Temp Decline Method"=FALSE, "Terminate Condition"=enum."C1-Terminate Draw @ Gallon Mark", "Condition Value #1"=1.0, "UE"=FALSE, "LE"=FALSE, "Comp"=FALSE, "Fan"=FALSE, "Test End Time (Sec)"=0.0, "Purge Until Cutout"=FALSE, "Start Conditions"=enum."At Time (Seconds)", "Condition Value #2"=3600.0, "Remove Power"=FALSE, "Time"=82800.0, "Check Special Cond."=enum."SC1-Do Nothing", "Condition#"=enum."N/A", "Draw Flags"=enum."N/A", "Data Processing Delay (FHD 15sec, UEF 5 Sec)"=0.0, "Test Complete"=FALSE}, {"Sequence #"=7.0, "Cycles"=1, "Mode Setting"="", "Flow Rate (GPM)"=1.7, "Temperature (F)"=58.0, "Reset Timer"=FALSE, "Use Temp Decline Method"=FALSE, "Terminate Condition"=enum."C1-Terminate Draw @ Gallon Mark", "Condition Value #1"=6.0, "UE"=FALSE, "LE"=FALSE, "Comp"=FALSE, "Fan"=FALSE, "Test End Time (Sec)"=0.0, "Purge Until Cutout"=FALSE, "Start Conditions"=enum."At Time (Seconds)", "Condition Value #2"=37800.0, "Remove Power"=FALSE, "Time"=82800.0, "Check Special Cond."=enum."SC1-Do Nothing", "Condition#"=enum."N/A", "Draw Flags"=enum."N/A", "Data Processing Delay (FHD 15sec, UEF 5 Sec)"=0.0, "Test Complete"=FALSE}, {"Sequence #"=8.0, "Cycles"=1, "Mode Setting"="", "Flow Rate (GPM)"=1.7, "Temperature (F)"=58.0, "Reset Timer"=FALSE, "Use Temp Decline Method"=FALSE, "Terminate Condition"=enum."C1-Terminate Draw @ Gallon Mark", "Condition Value #1"=4.0, "UE"=FALSE, "LE"=FALSE, "Comp"=FALSE, "Fan"=FALSE, "Test End Time (Sec)"=0.0, "Purge Until Cutout"=FALSE, "Start Conditions"=enum."At Time (Seconds)", "Condition Value #2"=41400.0, "Remove Power"=FALSE, "Time"=82800.0, "Check Special Cond."=enum."SC1-Do Nothing", "Condition#"=enum."N/A", "Draw Flags"=enum."N/A", "Data Processing Delay (FHD 15sec, UEF 5 Sec)"=0.0, "Test Complete"=FALSE}, {"Sequence #"=9.0, "Cycles"=1, "Mode Setting"="", "Flow Rate (GPM)"=1.0, "Temperature (F)"=58.0, "Reset Timer"=FALSE, "Use Temp Decline Method"=FALSE, "Terminate Condition"=enum."C1-Terminate Draw @ Gallon Mark", "Condition Value #1"=1.0, "UE"=FALSE, "LE"=FALSE, "Comp"=FALSE, "Fan"=FALSE, "Test End Time (Sec)"=0.0, "Purge Until Cutout"=FALSE, "Start Conditions"=enum."At Time (Seconds)", "Condition Value #2"=43200.0, "Remove Power"=FALSE, "Time"=82800.0, "Check Special Cond."=enum."SC1-Do Nothing", "Condition#"=enum."N/A", "Draw Flags"=enum."N/A", "Data Processing Delay (FHD 15sec, UEF 5 Sec)"=0.0, "Test Complete"=FALSE}, {"Sequence #"=10.0, "Cycles"=1, "Mode Setting"="", "Flow Rate (GPM)"=1.0, "Temperature (F)"=58.0, "Reset Timer"=FALSE, "Use Temp Decline Method"=FALSE, "Terminate Condition"=enum."C1-Terminate Draw @ Gallon Mark", "Condition Value #1"=1.0, "UE"=FALSE, "LE"=FALSE, "Comp"=FALSE, "Fan"=FALSE, "Test End Time (Sec)"=0.0, "Purge Until Cutout"=FALSE, "Start Conditions"=enum."At Time (Seconds)", "Condition Value #2"=45900.0, "Remove Power"=FALSE, "Time"=82800.0, "Check Special Cond."=enum."SC1-Do Nothing", "Condition#"=enum."N/A", "Draw Flags"=enum."N/A", "Data Processing Delay (FHD 15sec, UEF 5 Sec)"=0.0, "Test Complete"=FALSE}, {"Sequence #"=11.0, "Cycles"=1, "Mode Setting"="", "Flow Rate (GPM)"=1.0, "Temperature (F)"=58.0, "Reset Timer"=FALSE, "Use Temp Decline Method"=FALSE, "Terminate Condition"=enum."C1-Terminate Draw @ Gallon Mark", "Condition Value #1"=1.0, "UE"=FALSE, "LE"=FALSE, "Comp"=FALSE, "Fan"=FALSE, "Test End Time (Sec)"=0.0, "Purge Until Cutout"=FALSE, "Start Conditions"=enum."At Time (Seconds)", "Condition Value #2"=46200.0, "Remove Power"=FALSE, "Time"=82800.0, "Check Special Cond."=enum."SC1-Do Nothing", "Condition#"=enum."N/A", "Draw Flags"=enum."N/A", "Data Processing Delay (FHD 15sec, UEF 5 Sec)"=0.0, "Test Complete"=FALSE}, {"Sequence #"=12.0, "Cycles"=1, "Mode Setting"="", "Flow Rate (GPM)"=1.0, "Temperature (F)"=58.0, "Reset Timer"=FALSE, "Use Temp Decline Method"=FALSE, "Terminate Condition"=enum."C1-Terminate Draw @ Gallon Mark", "Condition Value #1"=2.0, "UE"=FALSE, "LE"=FALSE, "Comp"=FALSE, "Fan"=FALSE, "Test End Time (Sec)"=0.0, "Purge Until Cutout"=FALSE, "Start Conditions"=enum."At Time (Seconds)", "Condition Value #2"=58500.0, "Remove Power"=FALSE, "Time"=82800.0, "Check Special Cond."=enum."SC1-Do Nothing", "Condition#"=enum."N/A", "Draw Flags"=enum."N/A", "Data Processing Delay (FHD 15sec, UEF 5 Sec)"=0.0, "Test Complete"=FALSE}, {"Sequence #"=13.0, "Cycles"=1, "Mode Setting"="", "Flow Rate (GPM)"=1.7, "Temperature (F)"=58.0, "Reset Timer"=FALSE, "Use Temp Decline Method"=FALSE, "Terminate Condition"=enum."C1-Terminate Draw @ Gallon Mark", "Condition Value #1"=2.0, "UE"=FALSE, "LE"=FALSE, "Comp"=FALSE, "Fan"=FALSE, "Test End Time (Sec)"=0.0, "Purge Until Cutout"=FALSE, "Start Conditions"=enum."At Time (Seconds)", "Condition Value #2"=60300.0, "Remove Power"=FALSE, "Time"=82800.0, "Check Special Cond."=enum."SC1-Do Nothing", "Condition#"=enum."N/A", "Draw Flags"=enum."N/A", "Data Processing Delay (FHD 15sec, UEF 5 Sec)"=0.0, "Test Complete"=FALSE}, {"Sequence #"=14.0, "Cycles"=1, "Mode Setting"="", "Flow Rate (GPM)"=1.7, "Temperature (F)"=58.0, "Reset Timer"=FALSE, "Use Temp Decline Method"=FALSE, "Terminate Condition"=enum."C1-Terminate Draw @ Gallon Mark", "Condition Value #1"=3.0, "UE"=FALSE, "LE"=FALSE, "Comp"=FALSE, "Fan"=FALSE, "Test End Time (Sec)"=86400.0, "Purge Until Cutout"=FALSE, "Start Conditions"=enum."At Time (Seconds)", "Condition Value #2"=61200.0, "Remove Power"=TRUE, "Time"=82800.0, "Check Special Cond."=enum."SC1-Do Nothing", "Condition#"=enum."N/A", "Draw Flags"=enum."N/A", "Data Processing Delay (FHD 15sec, UEF 5 Sec)"=0.0, "Test Complete"=FALSE}] {"Time" format="%<%H:%M:%S>t"}
  in  "Standard Heat-Up (80 Gallon) Heat Pump":T21[](array[typedef])=[{"Sequence #"=1.0, "Cycles"=1, "Mode Setting"="", "Flow Rate (GPM)"=3.0, "Temperature (F)"=58.0, "Reset Timer"=FALSE, "Use Temp Decline Method"=FALSE, "Terminate Condition"=enum."C7-Until Any Heat Source", "Condition Value #1"=0.0, "UE"=FALSE, "LE"=FALSE, "Comp"=FALSE, "Fan"=FALSE, "Test End Time (Sec)"=0.0, "Purge Until Cutout"=FALSE, "Start Conditions"=enum."Heat Source Cutout", "Condition Value #2"=0.0, "Remove Power"=FALSE, "Time"=0.0, "Check Special Cond."=enum."SC1-Do Nothing", "Condition#"=enum."N/A", "Draw Flags"=enum."N/A", "Data Processing Delay (FHD 15sec, UEF 5 Sec)"=15.0, "Test Complete"=FALSE}, {"Sequence #"=2.0, "Cycles"=1, "Mode Setting"="", "Flow Rate (GPM)"=3.0, "Temperature (F)"=58.0, "Reset Timer"=TRUE, "Use Temp Decline Method"=FALSE, "Terminate Condition"=enum."C9-Do Nothing", "Condition Value #1"=0.0, "UE"=FALSE, "LE"=FALSE, "Comp"=FALSE, "Fan"=FALSE, "Test End Time (Sec)"=0.0, "Purge Until Cutout"=FALSE, "Start Conditions"=enum."Heat Source Cutout", "Condition Value #2"=0.0, "Remove Power"=FALSE, "Time"=0.0, "Check Special Cond."=enum."SC1-Do Nothing", "Condition#"=enum."N/A", "Draw Flags"=enum."N/A", "Data Processing Delay (FHD 15sec, UEF 5 Sec)"=15.0, "Test Complete"=FALSE}, {"Sequence #"=3.0, "Cycles"=1, "Mode Setting"="", "Flow Rate (GPM)"=3.0, "Temperature (F)"=58.0, "Reset Timer"=FALSE, "Use Temp Decline Method"=FALSE, "Terminate Condition"=enum."C1-Terminate Draw @ Gallon Mark", "Condition Value #1"=10.72, "UE"=FALSE, "LE"=FALSE, "Comp"=FALSE, "Fan"=FALSE, "Test End Time (Sec)"=0.0, "Purge Until Cutout"=FALSE, "Start Conditions"=enum."Every X (Seconds)", "Condition Value #2"=1800.0, "Remove Power"=FALSE, "Time"=0.0, "Check Special Cond."=enum."SC1-Do Nothing", "Condition#"=enum."N/A", "Draw Flags"=enum."N/A", "Data Processing Delay (FHD 15sec, UEF 5 Sec)"=15.0, "Test Complete"=FALSE}, {"Sequence #"=4.0, "Cycles"=1, "Mode Setting"="", "Flow Rate (GPM)"=3.0, "Temperature (F)"=58.0, "Reset Timer"=FALSE, "Use Temp Decline Method"=FALSE, "Terminate Condition"=enum."C1-Terminate Draw @ Gallon Mark", "Condition Value #1"=10.72, "UE"=FALSE, "LE"=FALSE, "Comp"=FALSE, "Fan"=FALSE, "Test End Time (Sec)"=0.0, "Purge Until Cutout"=FALSE, "Start Conditions"=enum."Every X (Seconds)", "Condition Value #2"=3600.0, "Remove Power"=FALSE, "Time"=0.0, "Check Special Cond."=enum."SC1-Do Nothing", "Condition#"=enum."N/A", "Draw Flags"=enum."N/A", "Data Processing Delay (FHD 15sec, UEF 5 Sec)"=15.0, "Test Complete"=FALSE}, {"Sequence #"=5.0, "Cycles"=1, "Mode Setting"="", "Flow Rate (GPM)"=3.0, "Temperature (F)"=58.0, "Reset Timer"=FALSE, "Use Temp Decline Method"=FALSE, "Terminate Condition"=enum."C9-Do Nothing", "Condition Value #1"=0.0, "UE"=FALSE, "LE"=FALSE, "Comp"=FALSE, "Fan"=FALSE, "Test End Time (Sec)"=0.0, "Purge Until Cutout"=FALSE, "Start Conditions"=enum."Every X (Seconds)", "Condition Value #2"=5.0, "Remove Power"=FALSE, "Time"=0.0, "Check Special Cond."=enum."SC2-Check Heat Source (On-C2/Off-C1)", "Condition#"=enum."N/A", "Draw Flags"=enum."N/A", "Data Processing Delay (FHD 15sec, UEF 5 Sec)"=15.0, "Test Complete"=FALSE}, {"Sequence #"=6.0, "Cycles"=1, "Mode Setting"="", "Flow Rate (GPM)"=3.0, "Temperature (F)"=58.0, "Reset Timer"=FALSE, "Use Temp Decline Method"=FALSE, "Terminate Condition"=enum."C9-Do Nothing", "Condition Value #1"=0.0, "UE"=FALSE, "LE"=FALSE, "Comp"=FALSE, "Fan"=FALSE, "Test End Time (Sec)"=0.0, "Purge Until Cutout"=FALSE, "Start Conditions"=enum."Every X (Seconds)", "Condition Value #2"=600.0, "Remove Power"=FALSE, "Time"=0.0, "Check Special Cond."=enum."SC4-Check Heat Source ON/Fail", "Condition#"=enum."C1", "Draw Flags"=enum."N/A", "Data Processing Delay (FHD 15sec, UEF 5 Sec)"=15.0, "Test Complete"=FALSE}, {"Sequence #"=7.0, "Cycles"=1, "Mode Setting"="", "Flow Rate (GPM)"=3.0, "Temperature (F)"=58.0, "Reset Timer"=FALSE, "Use Temp Decline Method"=FALSE, "Terminate Condition"=enum."C9-Do Nothing", "Condition Value #1"=0.0, "UE"=FALSE, "LE"=FALSE, "Comp"=FALSE, "Fan"=FALSE, "Test End Time (Sec)"=0.0, "Purge Until Cutout"=FALSE, "Start Conditions"=enum."Heat Source Cutout", "Condition Value #2"=0.0, "Remove Power"=FALSE, "Time"=0.0, "Check Special Cond."=enum."SC1-Do Nothing", "Condition#"=enum."C1", "Draw Flags"=enum."N/A", "Data Processing Delay (FHD 15sec, UEF 5 Sec)"=15.0, "Test Complete"=FALSE}, {"Sequence #"=8.0, "Cycles"=1, "Mode Setting"="", "Flow Rate (GPM)"=3.0, "Temperature (F)"=58.0, "Reset Timer"=FALSE, "Use Temp Decline Method"=FALSE, "Terminate Condition"=enum."C1-Terminate Draw @ Gallon Mark", "Condition Value #1"=40.0, "UE"=FALSE, "LE"=FALSE, "Comp"=FALSE, "Fan"=FALSE, "Test End Time (Sec)"=0.0, "Purge Until Cutout"=FALSE, "Start Conditions"=enum."Every X (Seconds)", "Condition Value #2"=600.0, "Remove Power"=FALSE, "Time"=0.0, "Check Special Cond."=enum."SC1-Do Nothing", "Condition#"=enum."C1", "Draw Flags"=enum."SmlMedLrg(7)", "Data Processing Delay (FHD 15sec, UEF 5 Sec)"=15.0, "Test Complete"=FALSE}, {"Sequence #"=9.0, "Cycles"=1, "Mode Setting"="", "Flow Rate (GPM)"=3.0, "Temperature (F)"=58.0, "Reset Timer"=FALSE, "Use Temp Decline Method"=FALSE, "Terminate Condition"=enum."C1-Terminate Draw @ Gallon Mark", "Condition Value #1"=40.0, "UE"=FALSE, "LE"=FALSE, "Comp"=FALSE, "Fan"=FALSE, "Test End Time (Sec)"=0.0, "Purge Until Cutout"=FALSE, "Start Conditions"=enum."Every X (Seconds)", "Condition Value #2"=5.0, "Remove Power"=FALSE, "Time"=0.0, "Check Special Cond."=enum."SC1-Do Nothing", "Condition#"=enum."C2", "Draw Flags"=enum."SmlMedLrg(7)", "Data Processing Delay (FHD 15sec, UEF 5 Sec)"=15.0, "Test Complete"=FALSE}, {"Sequence #"=10.0, "Cycles"=1, "Mode Setting"="Heat Pump", "Flow Rate (GPM)"=3.0, "Temperature (F)"=58.0, "Reset Timer"=FALSE, "Use Temp Decline Method"=FALSE, "Terminate Condition"=enum."C9-Do Nothing", "Condition Value #1"=0.0, "UE"=FALSE, "LE"=FALSE, "Comp"=FALSE, "Fan"=FALSE, "Test End Time (Sec)"=0.0, "Purge Until Cutout"=FALSE, "Start Conditions"=enum."Heat Source Cutout", "Condition Value #2"=0.0, "Remove Power"=FALSE, "Time"=0.0, "Check Special Cond."=enum."SC1-Do Nothing", "Condition#"=enum."N/A", "Draw Flags"=enum."N/A", "Data Processing Delay (FHD 15sec, UEF 5 Sec)"=15.0, "Test Complete"=FALSE}, {"Sequence #"=11.0, "Cycles"=1, "Mode Setting"="", "Flow Rate (GPM)"=3.0, "Temperature (F)"=58.0, "Reset Timer"=FALSE, "Use Temp Decline Method"=FALSE, "Terminate Condition"=enum."C9-Do Nothing", "Condition Value #1"=0.0, "UE"=FALSE, "LE"=FALSE, "Comp"=FALSE, "Fan"=FALSE, "Test End Time (Sec)"=0.0, "Purge Until Cutout"=FALSE, "Start Conditions"=enum."Heat Source Cutout", "Condition Value #2"=0.0, "Remove Power"=FALSE, "Time"=0.0, "Check Special Cond."=enum."SC1-Do Nothing", "Condition#"=enum."N/A", "Draw Flags"=enum."N/A", "Data Processing Delay (FHD 15sec, UEF 5 Sec)"=15.0, "Test Complete"=FALSE}, {"Sequence #"=12.0, "Cycles"=1, "Mode Setting"="", "Flow Rate (GPM)"=3.0, "Temperature (F)"=58.0, "Reset Timer"=FALSE, "Use Temp Decline Method"=FALSE, "Terminate Condition"=enum."C9-Do Nothing", "Condition Value #1"=0.0, "UE"=FALSE, "LE"=FALSE, "Comp"=FALSE, "Fan"=FALSE, "Test End Time (Sec)"=0.0, "Purge Until Cutout"=FALSE, "Start Conditions"=enum."Every X (Seconds)", "Condition Value #2"=1800.0, "Remove Power"=FALSE, "Time"=0.0, "Check Special Cond."=enum."SC1-Do Nothing", "Condition#"=enum."N/A", "Draw Flags"=enum."N/A", "Data Processing Delay (FHD 15sec, UEF 5 Sec)"=15.0, "Test Complete"=FALSE}, {"Sequence #"=13.0, "Cycles"=1, "Mode Setting"="", "Flow Rate (GPM)"=3.0, "Temperature (F)"=58.0, "Reset Timer"=FALSE, "Use Temp Decline Method"=FALSE, "Terminate Condition"=enum."C9-Do Nothing", "Condition Value #1"=0.0, "UE"=FALSE, "LE"=FALSE, "Comp"=FALSE, "Fan"=FALSE, "Test End Time (Sec)"=0.0, "Purge Until Cutout"=FALSE, "Start Conditions"=enum."Heat Source Cutout", "Condition Value #2"=0.0, "Remove Power"=FALSE, "Time"=0.0, "Check Special Cond."=enum."SC1-Do Nothing", "Condition#"=enum."N/A", "Draw Flags"=enum."N/A", "Data Processing Delay (FHD 15sec, UEF 5 Sec)"=15.0, "Test Complete"=TRUE}] {"Time" format="%<%H:%M:%S>t"}
  in  "Standard Heat-Up (80 Gallon)":T21[](array[typedef])=[{"Sequence #"=1.0, "Cycles"=1, "Mode Setting"="", "Flow Rate (GPM)"=3.0, "Temperature (F)"=58.0, "Reset Timer"=FALSE, "Use Temp Decline Method"=FALSE, "Terminate Condition"=enum."C7-Until Any Heat Source", "Condition Value #1"=0.0, "UE"=FALSE, "LE"=FALSE, "Comp"=FALSE, "Fan"=FALSE, "Test End Time (Sec)"=0.0, "Purge Until Cutout"=FALSE, "Start Conditions"=enum."Heat Source Cutout", "Condition Value #2"=0.0, "Remove Power"=FALSE, "Time"=0.0, "Check Special Cond."=enum."SC1-Do Nothing", "Condition#"=enum."N/A", "Draw Flags"=enum."N/A", "Data Processing Delay (FHD 15sec, UEF 5 Sec)"=15.0, "Test Complete"=FALSE}, {"Sequence #"=2.0, "Cycles"=1, "Mode Setting"="", "Flow Rate (GPM)"=3.0, "Temperature (F)"=58.0, "Reset Timer"=TRUE, "Use Temp Decline Method"=FALSE, "Terminate Condition"=enum."C9-Do Nothing", "Condition Value #1"=0.0, "UE"=FALSE, "LE"=FALSE, "Comp"=FALSE, "Fan"=FALSE, "Test End Time (Sec)"=0.0, "Purge Until Cutout"=FALSE, "Start Conditions"=enum."Heat Source Cutout", "Condition Value #2"=0.0, "Remove Power"=FALSE, "Time"=0.0, "Check Special Cond."=enum."SC1-Do Nothing", "Condition#"=enum."N/A", "Draw Flags"=enum."N/A", "Data Processing Delay (FHD 15sec, UEF 5 Sec)"=15.0, "Test Complete"=FALSE}, {"Sequence #"=3.0, "Cycles"=1, "Mode Setting"="", "Flow Rate (GPM)"=3.0, "Temperature (F)"=58.0, "Reset Timer"=FALSE, "Use Temp Decline Method"=FALSE, "Terminate Condition"=enum."C1-Terminate Draw @ Gallon Mark", "Condition Value #1"=10.72, "UE"=FALSE, "LE"=FALSE, "Comp"=FALSE, "Fan"=FALSE, "Test End Time (Sec)"=0.0, "Purge Until Cutout"=FALSE, "Start Conditions"=enum."Every X (Seconds)", "Condition Value #2"=1800.0, "Remove Power"=FALSE, "Time"=0.0, "Check Special Cond."=enum."SC1-Do Nothing", "Condition#"=enum."N/A", "Draw Flags"=enum."N/A", "Data Processing Delay (FHD 15sec, UEF 5 Sec)"=15.0, "Test Complete"=FALSE}, {"Sequence #"=4.0, "Cycles"=1, "Mode Setting"="", "Flow Rate (GPM)"=3.0, "Temperature (F)"=58.0, "Reset Timer"=FALSE, "Use Temp Decline Method"=FALSE, "Terminate Condition"=enum."C1-Terminate Draw @ Gallon Mark", "Condition Value #1"=10.72, "UE"=FALSE, "LE"=FALSE, "Comp"=FALSE, "Fan"=FALSE, "Test End Time (Sec)"=0.0, "Purge Until Cutout"=FALSE, "Start Conditions"=enum."Every X (Seconds)", "Condition Value #2"=3600.0, "Remove Power"=FALSE, "Time"=0.0, "Check Special Cond."=enum."SC1-Do Nothing", "Condition#"=enum."N/A", "Draw Flags"=enum."N/A", "Data Processing Delay (FHD 15sec, UEF 5 Sec)"=15.0, "Test Complete"=FALSE}, {"Sequence #"=5.0, "Cycles"=1, "Mode Setting"="", "Flow Rate (GPM)"=3.0, "Temperature (F)"=58.0, "Reset Timer"=FALSE, "Use Temp Decline Method"=FALSE, "Terminate Condition"=enum."C9-Do Nothing", "Condition Value #1"=0.0, "UE"=FALSE, "LE"=FALSE, "Comp"=FALSE, "Fan"=FALSE, "Test End Time (Sec)"=0.0, "Purge Until Cutout"=FALSE, "Start Conditions"=enum."Every X (Seconds)", "Condition Value #2"=5.0, "Remove Power"=FALSE, "Time"=0.0, "Check Special Cond."=enum."SC2-Check Heat Source (On-C2/Off-C1)", "Condition#"=enum."N/A", "Draw Flags"=enum."N/A", "Data Processing Delay (FHD 15sec, UEF 5 Sec)"=15.0, "Test Complete"=FALSE}, {"Sequence #"=6.0, "Cycles"=1, "Mode Setting"="", "Flow Rate (GPM)"=3.0, "Temperature (F)"=58.0, "Reset Timer"=FALSE, "Use Temp Decline Method"=FALSE, "Terminate Condition"=enum."C9-Do Nothing", "Condition Value #1"=0.0, "UE"=FALSE, "LE"=FALSE, "Comp"=FALSE, "Fan"=FALSE, "Test End Time (Sec)"=0.0, "Purge Until Cutout"=FALSE, "Start Conditions"=enum."Every X (Seconds)", "Condition Value #2"=600.0, "Remove Power"=FALSE, "Time"=0.0, "Check Special Cond."=enum."SC4-Check Heat Source ON/Fail", "Condition#"=enum."C1", "Draw Flags"=enum."N/A", "Data Processing Delay (FHD 15sec, UEF 5 Sec)"=15.0, "Test Complete"=FALSE}, {"Sequence #"=7.0, "Cycles"=1, "Mode Setting"="", "Flow Rate (GPM)"=3.0, "Temperature (F)"=58.0, "Reset Timer"=FALSE, "Use Temp Decline Method"=FALSE, "Terminate Condition"=enum."C9-Do Nothing", "Condition Value #1"=0.0, "UE"=FALSE, "LE"=FALSE, "Comp"=FALSE, "Fan"=FALSE, "Test End Time (Sec)"=0.0, "Purge Until Cutout"=FALSE, "Start Conditions"=enum."Heat Source Cutout", "Condition Value #2"=0.0, "Remove Power"=FALSE, "Time"=0.0, "Check Special Cond."=enum."SC1-Do Nothing", "Condition#"=enum."C1", "Draw Flags"=enum."N/A", "Data Processing Delay (FHD 15sec, UEF 5 Sec)"=15.0, "Test Complete"=FALSE}, {"Sequence #"=8.0, "Cycles"=1, "Mode Setting"="", "Flow Rate (GPM)"=3.0, "Temperature (F)"=58.0, "Reset Timer"=FALSE, "Use Temp Decline Method"=FALSE, "Terminate Condition"=enum."C8-Specific Heat Source", "Condition Value #1"=0.0, "UE"=TRUE, "LE"=FALSE, "Comp"=FALSE, "Fan"=FALSE, "Test End Time (Sec)"=0.0, "Purge Until Cutout"=FALSE, "Start Conditions"=enum."Every X (Seconds)", "Condition Value #2"=600.0, "Remove Power"=FALSE, "Time"=0.0, "Check Special Cond."=enum."SC1-Do Nothing", "Condition#"=enum."C1", "Draw Flags"=enum."SmlMedLrg(7)", "Data Processing Delay (FHD 15sec, UEF 5 Sec)"=15.0, "Test Complete"=FALSE}, {"Sequence #"=9.0, "Cycles"=1, "Mode Setting"="", "Flow Rate (GPM)"=3.0, "Temperature (F)"=58.0, "Reset Timer"=FALSE, "Use Temp Decline Method"=FALSE, "Terminate Condition"=enum."C8-Specific Heat Source", "Condition Value #1"=0.0, "UE"=TRUE, "LE"=FALSE, "Comp"=FALSE, "Fan"=FALSE, "Test End Time (Sec)"=0.0, "Purge Until Cutout"=FALSE, "Start Conditions"=enum."Every X (Seconds)", "Condition Value #2"=0.0, "Remove Power"=FALSE, "Time"=0.0, "Check Special Cond."=enum."SC1-Do Nothing", "Condition#"=enum."C2", "Draw Flags"=enum."SmlMedLrg(7)", "Data Processing Delay (FHD 15sec, UEF 5 Sec)"=15.0, "Test Complete"=FALSE}, {"Sequence #"=10.0, "Cycles"=1, "Mode Setting"="Heat Pump", "Flow Rate (GPM)"=3.0, "Temperature (F)"=58.0, "Reset Timer"=FALSE, "Use Temp Decline Method"=FALSE, "Terminate Condition"=enum."C9-Do Nothing", "Condition Value #1"=0.0, "UE"=FALSE, "LE"=FALSE, "Comp"=FALSE, "Fan"=FALSE, "Test End Time (Sec)"=0.0, "Purge Until Cutout"=FALSE, "Start Conditions"=enum."Wait for UE Cutout", "Condition Value #2"=0.0, "Remove Power"=FALSE, "Time"=0.0, "Check Special Cond."=enum."SC1-Do Nothing", "Condition#"=enum."N/A", "Draw Flags"=enum."N/A", "Data Processing Delay (FHD 15sec, UEF 5 Sec)"=15.0, "Test Complete"=FALSE}, {"Sequence #"=11.0, "Cycles"=1, "Mode Setting"="", "Flow Rate (GPM)"=3.0, "Temperature (F)"=58.0, "Reset Timer"=FALSE, "Use Temp Decline Method"=FALSE, "Terminate Condition"=enum."C9-Do Nothing", "Condition Value #1"=0.0, "UE"=FALSE, "LE"=FALSE, "Comp"=FALSE, "Fan"=FALSE, "Test End Time (Sec)"=0.0, "Purge Until Cutout"=FALSE, "Start Conditions"=enum."Heat Source Cutout", "Condition Value #2"=0.0, "Remove Power"=FALSE, "Time"=0.0, "Check Special Cond."=enum."SC1-Do Nothing", "Condition#"=enum."N/A", "Draw Flags"=enum."N/A", "Data Processing Delay (FHD 15sec, UEF 5 Sec)"=15.0, "Test Complete"=FALSE}, {"Sequence #"=12.0, "Cycles"=1, "Mode Setting"="", "Flow Rate (GPM)"=3.0, "Temperature (F)"=58.0, "Reset Timer"=FALSE, "Use Temp Decline Method"=FALSE, "Terminate Condition"=enum."C9-Do Nothing", "Condition Value #1"=0.0, "UE"=FALSE, "LE"=FALSE, "Comp"=FALSE, "Fan"=FALSE, "Test End Time (Sec)"=0.0, "Purge Until Cutout"=FALSE, "Start Conditions"=enum."Every X (Seconds)", "Condition Value #2"=1800.0, "Remove Power"=FALSE, "Time"=0.0, "Check Special Cond."=enum."SC1-Do Nothing", "Condition#"=enum."N/A", "Draw Flags"=enum."N/A", "Data Processing Delay (FHD 15sec, UEF 5 Sec)"=15.0, "Test Complete"=FALSE}, {"Sequence #"=13.0, "Cycles"=1, "Mode Setting"="", "Flow Rate (GPM)"=3.0, "Temperature (F)"=58.0, "Reset Timer"=FALSE, "Use Temp Decline Method"=FALSE, "Terminate Condition"=enum."C9-Do Nothing", "Condition Value #1"=0.0, "UE"=FALSE, "LE"=FALSE, "Comp"=FALSE, "Fan"=FALSE, "Test End Time (Sec)"=0.0, "Purge Until Cutout"=FALSE, "Start Conditions"=enum."Heat Source Cutout", "Condition Value #2"=0.0, "Remove Power"=FALSE, "Time"=0.0, "Check Special Cond."=enum."SC1-Do Nothing", "Condition#"=enum."N/A", "Draw Flags"=enum."N/A", "Data Processing Delay (FHD 15sec, UEF 5 Sec)"=15.0, "Test Complete"=TRUE}] {"Time" format="%<%H:%M:%S>t"}
  in  "Standard Heat-Up (50 Gallon) Heat Pump":T21[](array[typedef])=[{"Sequence #"=1.0, "Cycles"=1, "Mode Setting"="", "Flow Rate (GPM)"=3.0, "Temperature (F)"=58.0, "Reset Timer"=FALSE, "Use Temp Decline Method"=FALSE, "Terminate Condition"=enum."C7-Until Any Heat Source", "Condition Value #1"=0.0, "UE"=FALSE, "LE"=FALSE, "Comp"=FALSE, "Fan"=FALSE, "Test End Time (Sec)"=0.0, "Purge Until Cutout"=FALSE, "Start Conditions"=enum."Heat Source Cutout", "Condition Value #2"=0.0, "Remove Power"=FALSE, "Time"=3600.0, "Check Special Cond."=enum."SC1-Do Nothing", "Condition#"=enum."N/A", "Draw Flags"=enum."N/A", "Data Processing Delay (FHD 15sec, UEF 5 Sec)"=15.0, "Test Complete"=FALSE}, {"Sequence #"=2.0, "Cycles"=1, "Mode Setting"="", "Flow Rate (GPM)"=3.0, "Temperature (F)"=58.0, "Reset Timer"=TRUE, "Use Temp Decline Method"=FALSE, "Terminate Condition"=enum."C9-Do Nothing", "Condition Value #1"=0.0, "UE"=FALSE, "LE"=FALSE, "Comp"=FALSE, "Fan"=FALSE, "Test End Time (Sec)"=0.0, "Purge Until Cutout"=FALSE, "Start Conditions"=enum."Heat Source Cutout", "Condition Value #2"=0.0, "Remove Power"=FALSE, "Time"=3600.0, "Check Special Cond."=enum."SC1-Do Nothing", "Condition#"=enum."N/A", "Draw Flags"=enum."N/A", "Data Processing Delay (FHD 15sec, UEF 5 Sec)"=15.0, "Test Complete"=FALSE}, {"Sequence #"=3.0, "Cycles"=1, "Mode Setting"="", "Flow Rate (GPM)"=3.0, "Temperature (F)"=58.0, "Reset Timer"=FALSE, "Use Temp Decline Method"=FALSE, "Terminate Condition"=enum."C1-Terminate Draw @ Gallon Mark", "Condition Value #1"=10.72, "UE"=FALSE, "LE"=FALSE, "Comp"=FALSE, "Fan"=FALSE, "Test End Time (Sec)"=0.0, "Purge Until Cutout"=FALSE, "Start Conditions"=enum."Every X (Seconds)", "Condition Value #2"=1800.0, "Remove Power"=FALSE, "Time"=3600.0, "Check Special Cond."=enum."SC1-Do Nothing", "Condition#"=enum."N/A", "Draw Flags"=enum."N/A", "Data Processing Delay (FHD 15sec, UEF 5 Sec)"=15.0, "Test Complete"=FALSE}, {"Sequence #"=4.0, "Cycles"=1, "Mode Setting"="", "Flow Rate (GPM)"=3.0, "Temperature (F)"=58.0, "Reset Timer"=FALSE, "Use Temp Decline Method"=FALSE, "Terminate Condition"=enum."C9-Do Nothing", "Condition Value #1"=0.0, "UE"=FALSE, "LE"=FALSE, "Comp"=FALSE, "Fan"=FALSE, "Test End Time (Sec)"=0.0, "Purge Until Cutout"=FALSE, "Start Conditions"=enum."Every X (Seconds)", "Condition Value #2"=5.0, "Remove Power"=FALSE, "Time"=3600.0, "Check Special Cond."=enum."SC2-Check Heat Source (On-C2/Off-C1)", "Condition#"=enum."N/A", "Draw Flags"=enum."N/A", "Data Processing Delay (FHD 15sec, UEF 5 Sec)"=15.0, "Test Complete"=FALSE}, {"Sequence #"=5.0, "Cycles"=1, "Mode Setting"="", "Flow Rate (GPM)"=3.0, "Temperature (F)"=58.0, "Reset Timer"=FALSE, "Use Temp Decline Method"=FALSE, "Terminate Condition"=enum."C9-Do Nothing", "Condition Value #1"=0.0, "UE"=FALSE, "LE"=FALSE, "Comp"=FALSE, "Fan"=FALSE, "Test End Time (Sec)"=0.0, "Purge Until Cutout"=FALSE, "Start Conditions"=enum."Every X (Seconds)", "Condition Value #2"=600.0, "Remove Power"=FALSE, "Time"=3600.0, "Check Special Cond."=enum."SC4-Check Heat Source ON/Fail", "Condition#"=enum."C1", "Draw Flags"=enum."N/A", "Data Processing Delay (FHD 15sec, UEF 5 Sec)"=15.0, "Test Complete"=FALSE}, {"Sequence #"=6.0, "Cycles"=1, "Mode Setting"="", "Flow Rate (GPM)"=3.0, "Temperature (F)"=58.0, "Reset Timer"=FALSE, "Use Temp Decline Method"=FALSE, "Terminate Condition"=enum."C9-Do Nothing", "Condition Value #1"=0.0, "UE"=FALSE, "LE"=FALSE, "Comp"=FALSE, "Fan"=FALSE, "Test End Time (Sec)"=0.0, "Purge Until Cutout"=FALSE, "Start Conditions"=enum."Heat Source Cutout", "Condition Value #2"=0.0, "Remove Power"=FALSE, "Time"=3600.0, "Check Special Cond."=enum."SC1-Do Nothing", "Condition#"=enum."C1", "Draw Flags"=enum."N/A", "Data Processing Delay (FHD 15sec, UEF 5 Sec)"=15.0, "Test Complete"=FALSE}, {"Sequence #"=7.0, "Cycles"=1, "Mode Setting"="", "Flow Rate (GPM)"=3.0, "Temperature (F)"=58.0, "Reset Timer"=FALSE, "Use Temp Decline Method"=FALSE, "Terminate Condition"=enum."C1-Terminate Draw @ Gallon Mark", "Condition Value #1"=40.0, "UE"=FALSE, "LE"=FALSE, "Comp"=FALSE, "Fan"=FALSE, "Test End Time (Sec)"=0.0, "Purge Until Cutout"=FALSE, "Start Conditions"=enum."Every X (Seconds)", "Condition Value #2"=600.0, "Remove Power"=FALSE, "Time"=3600.0, "Check Special Cond."=enum."SC1-Do Nothing", "Condition#"=enum."C1", "Draw Flags"=enum."SmlMedLrg(7)", "Data Processing Delay (FHD 15sec, UEF 5 Sec)"=15.0, "Test Complete"=FALSE}, {"Sequence #"=8.0, "Cycles"=1, "Mode Setting"="", "Flow Rate (GPM)"=3.0, "Temperature (F)"=58.0, "Reset Timer"=FALSE, "Use Temp Decline Method"=FALSE, "Terminate Condition"=enum."C1-Terminate Draw @ Gallon Mark", "Condition Value #1"=40.0, "UE"=FALSE, "LE"=FALSE, "Comp"=FALSE, "Fan"=FALSE, "Test End Time (Sec)"=0.0, "Purge Until Cutout"=FALSE, "Start Conditions"=enum."Every X (Seconds)", "Condition Value #2"=5.0, "Remove Power"=FALSE, "Time"=3600.0, "Check Special Cond."=enum."SC1-Do Nothing", "Condition#"=enum."C2", "Draw Flags"=enum."SmlMedLrg(7)", "Data Processing Delay (FHD 15sec, UEF 5 Sec)"=15.0, "Test Complete"=FALSE}, {"Sequence #"=9.0, "Cycles"=1, "Mode Setting"="Heat Pump", "Flow Rate (GPM)"=3.0, "Temperature (F)"=58.0, "Reset Timer"=FALSE, "Use Temp Decline Method"=FALSE, "Terminate Condition"=enum."C9-Do Nothing", "Condition Value #1"=0.0, "UE"=FALSE, "LE"=FALSE, "Comp"=FALSE, "Fan"=FALSE, "Test End Time (Sec)"=0.0, "Purge Until Cutout"=FALSE, "Start Conditions"=enum."Heat Source Cutout", "Condition Value #2"=0.0, "Remove Power"=FALSE, "Time"=3600.0, "Check Special Cond."=enum."SC1-Do Nothing", "Condition#"=enum."N/A", "Draw Flags"=enum."N/A", "Data Processing Delay (FHD 15sec, UEF 5 Sec)"=15.0, "Test Complete"=FALSE}, {"Sequence #"=10.0, "Cycles"=1, "Mode Setting"="", "Flow Rate (GPM)"=3.0, "Temperature (F)"=58.0, "Reset Timer"=FALSE, "Use Temp Decline Method"=FALSE, "Terminate Condition"=enum."C9-Do Nothing", "Condition Value #1"=0.0, "UE"=FALSE, "LE"=FALSE, "Comp"=FALSE, "Fan"=FALSE, "Test End Time (Sec)"=0.0, "Purge Until Cutout"=FALSE, "Start Conditions"=enum."Every X (Seconds)", "Condition Value #2"=300.0, "Remove Power"=FALSE, "Time"=3600.0, "Check Special Cond."=enum."SC1-Do Nothing", "Condition#"=enum."N/A", "Draw Flags"=enum."N/A", "Data Processing Delay (FHD 15sec, UEF 5 Sec)"=15.0, "Test Complete"=FALSE}, {"Sequence #"=11.0, "Cycles"=1, "Mode Setting"="", "Flow Rate (GPM)"=3.0, "Temperature (F)"=58.0, "Reset Timer"=FALSE, "Use Temp Decline Method"=FALSE, "Terminate Condition"=enum."C9-Do Nothing", "Condition Value #1"=0.0, "UE"=FALSE, "LE"=FALSE, "Comp"=FALSE, "Fan"=FALSE, "Test End Time (Sec)"=0.0, "Purge Until Cutout"=FALSE, "Start Conditions"=enum."Heat Source Cutout", "Condition Value #2"=0.0, "Remove Power"=FALSE, "Time"=3600.0, "Check Special Cond."=enum."SC1-Do Nothing", "Condition#"=enum."N/A", "Draw Flags"=enum."N/A", "Data Processing Delay (FHD 15sec, UEF 5 Sec)"=15.0, "Test Complete"=FALSE}, {"Sequence #"=12.0, "Cycles"=1, "Mode Setting"="", "Flow Rate (GPM)"=3.0, "Temperature (F)"=58.0, "Reset Timer"=FALSE, "Use Temp Decline Method"=FALSE, "Terminate Condition"=enum."C9-Do Nothing", "Condition Value #1"=0.0, "UE"=FALSE, "LE"=FALSE, "Comp"=FALSE, "Fan"=FALSE, "Test End Time (Sec)"=0.0, "Purge Until Cutout"=FALSE, "Start Conditions"=enum."Every X (Seconds)", "Condition Value #2"=1800.0, "Remove Power"=FALSE, "Time"=3600.0, "Check Special Cond."=enum."SC1-Do Nothing", "Condition#"=enum."N/A", "Draw Flags"=enum."N/A", "Data Processing Delay (FHD 15sec, UEF 5 Sec)"=15.0, "Test Complete"=FALSE}, {"Sequence #"=13.0, "Cycles"=1, "Mode Setting"="", "Flow Rate (GPM)"=3.0, "Temperature (F)"=58.0, "Reset Timer"=FALSE, "Use Temp Decline Method"=FALSE, "Terminate Condition"=enum."C9-Do Nothing", "Condition Value #1"=0.0, "UE"=FALSE, "LE"=FALSE, "Comp"=FALSE, "Fan"=FALSE, "Test End Time (Sec)"=0.0, "Purge Until Cutout"=FALSE, "Start Conditions"=enum."Heat Source Cutout", "Condition Value #2"=0.0, "Remove Power"=FALSE, "Time"=3600.0, "Check Special Cond."=enum."SC1-Do Nothing", "Condition#"=enum."N/A", "Draw Flags"=enum."N/A", "Data Processing Delay (FHD 15sec, UEF 5 Sec)"=15.0, "Test Complete"=TRUE}] {"Time" format="%<%H:%M:%S>t"}
  in  "Standard Heat-Up (50 Gallon)":T21[](array[typedef])=[{"Sequence #"=1.0, "Cycles"=1, "Mode Setting"="", "Flow Rate (GPM)"=3.0, "Temperature (F)"=58.0, "Reset Timer"=FALSE, "Use Temp Decline Method"=FALSE, "Terminate Condition"=enum."C7-Until Any Heat Source", "Condition Value #1"=0.0, "UE"=FALSE, "LE"=FALSE, "Comp"=FALSE, "Fan"=FALSE, "Test End Time (Sec)"=0.0, "Purge Until Cutout"=FALSE, "Start Conditions"=enum."Heat Source Cutout", "Condition Value #2"=0.0, "Remove Power"=FALSE, "Time"=3600.0, "Check Special Cond."=enum."SC1-Do Nothing", "Condition#"=enum."N/A", "Draw Flags"=enum."N/A", "Data Processing Delay (FHD 15sec, UEF 5 Sec)"=15.0, "Test Complete"=FALSE}, {"Sequence #"=2.0, "Cycles"=1, "Mode Setting"="", "Flow Rate (GPM)"=3.0, "Temperature (F)"=58.0, "Reset Timer"=TRUE, "Use Temp Decline Method"=FALSE, "Terminate Condition"=enum."C9-Do Nothing", "Condition Value #1"=0.0, "UE"=FALSE, "LE"=FALSE, "Comp"=FALSE, "Fan"=FALSE, "Test End Time (Sec)"=0.0, "Purge Until Cutout"=FALSE, "Start Conditions"=enum."Heat Source Cutout", "Condition Value #2"=0.0, "Remove Power"=FALSE, "Time"=3600.0, "Check Special Cond."=enum."SC1-Do Nothing", "Condition#"=enum."N/A", "Draw Flags"=enum."N/A", "Data Processing Delay (FHD 15sec, UEF 5 Sec)"=15.0, "Test Complete"=FALSE}, {"Sequence #"=3.0, "Cycles"=1, "Mode Setting"="", "Flow Rate (GPM)"=3.0, "Temperature (F)"=58.0, "Reset Timer"=FALSE, "Use Temp Decline Method"=FALSE, "Terminate Condition"=enum."C1-Terminate Draw @ Gallon Mark", "Condition Value #1"=10.72, "UE"=FALSE, "LE"=FALSE, "Comp"=FALSE, "Fan"=FALSE, "Test End Time (Sec)"=0.0, "Purge Until Cutout"=FALSE, "Start Conditions"=enum."Every X (Seconds)", "Condition Value #2"=1800.0, "Remove Power"=FALSE, "Time"=3600.0, "Check Special Cond."=enum."SC1-Do Nothing", "Condition#"=enum."N/A", "Draw Flags"=enum."N/A", "Data Processing Delay (FHD 15sec, UEF 5 Sec)"=15.0, "Test Complete"=FALSE}, {"Sequence #"=4.0, "Cycles"=1, "Mode Setting"="", "Flow Rate (GPM)"=3.0, "Temperature (F)"=58.0, "Reset Timer"=FALSE, "Use Temp Decline Method"=FALSE, "Terminate Condition"=enum."C9-Do Nothing", "Condition Value #1"=0.0, "UE"=FALSE, "LE"=FALSE, "Comp"=FALSE, "Fan"=FALSE, "Test End Time (Sec)"=0.0, "Purge Until Cutout"=FALSE, "Start Conditions"=enum."Every X (Seconds)", "Condition Value #2"=5.0, "Remove Power"=FALSE, "Time"=3600.0, "Check Special Cond."=enum."SC2-Check Heat Source (On-C2/Off-C1)", "Condition#"=enum."N/A", "Draw Flags"=enum."N/A", "Data Processing Delay (FHD 15sec, UEF 5 Sec)"=15.0, "Test Complete"=FALSE}, {"Sequence #"=5.0, "Cycles"=1, "Mode Setting"="", "Flow Rate (GPM)"=3.0, "Temperature (F)"=58.0, "Reset Timer"=FALSE, "Use Temp Decline Method"=FALSE, "Terminate Condition"=enum."C9-Do Nothing", "Condition Value #1"=0.0, "UE"=FALSE, "LE"=FALSE, "Comp"=FALSE, "Fan"=FALSE, "Test End Time (Sec)"=0.0, "Purge Until Cutout"=FALSE, "Start Conditions"=enum."Every X (Seconds)", "Condition Value #2"=600.0, "Remove Power"=FALSE, "Time"=3600.0, "Check Special Cond."=enum."SC4-Check Heat Source ON/Fail", "Condition#"=enum."C1", "Draw Flags"=enum."N/A", "Data Processing Delay (FHD 15sec, UEF 5 Sec)"=15.0, "Test Complete"=FALSE}, {"Sequence #"=6.0, "Cycles"=1, "Mode Setting"="", "Flow Rate (GPM)"=3.0, "Temperature (F)"=58.0, "Reset Timer"=FALSE, "Use Temp Decline Method"=FALSE, "Terminate Condition"=enum."C9-Do Nothing", "Condition Value #1"=0.0, "UE"=FALSE, "LE"=FALSE, "Comp"=FALSE, "Fan"=FALSE, "Test End Time (Sec)"=0.0, "Purge Until Cutout"=FALSE, "Start Conditions"=enum."Heat Source Cutout", "Condition Value #2"=0.0, "Remove Power"=FALSE, "Time"=3600.0, "Check Special Cond."=enum."SC1-Do Nothing", "Condition#"=enum."C1", "Draw Flags"=enum."N/A", "Data Processing Delay (FHD 15sec, UEF 5 Sec)"=15.0, "Test Complete"=FALSE}, {"Sequence #"=7.0, "Cycles"=1, "Mode Setting"="", "Flow Rate (GPM)"=3.0, "Temperature (F)"=58.0, "Reset Timer"=FALSE, "Use Temp Decline Method"=FALSE, "Terminate Condition"=enum."C8-Specific Heat Source", "Condition Value #1"=0.0, "UE"=TRUE, "LE"=FALSE, "Comp"=FALSE, "Fan"=FALSE, "Test End Time (Sec)"=0.0, "Purge Until Cutout"=FALSE, "Start Conditions"=enum."Every X (Seconds)", "Condition Value #2"=0.0, "Remove Power"=FALSE, "Time"=3600.0, "Check Special Cond."=enum."SC1-Do Nothing", "Condition#"=enum."C1", "Draw Flags"=enum."SmlMedLrg(7)", "Data Processing Delay (FHD 15sec, UEF 5 Sec)"=15.0, "Test Complete"=FALSE}, {"Sequence #"=8.0, "Cycles"=1, "Mode Setting"="", "Flow Rate (GPM)"=3.0, "Temperature (F)"=58.0, "Reset Timer"=FALSE, "Use Temp Decline Method"=FALSE, "Terminate Condition"=enum."C8-Specific Heat Source", "Condition Value #1"=0.0, "UE"=TRUE, "LE"=FALSE, "Comp"=FALSE, "Fan"=FALSE, "Test End Time (Sec)"=0.0, "Purge Until Cutout"=FALSE, "Start Conditions"=enum."Every X (Seconds)", "Condition Value #2"=5.0, "Remove Power"=FALSE, "Time"=3600.0, "Check Special Cond."=enum."SC1-Do Nothing", "Condition#"=enum."C2", "Draw Flags"=enum."SmlMedLrg(7)", "Data Processing Delay (FHD 15sec, UEF 5 Sec)"=15.0, "Test Complete"=FALSE}, {"Sequence #"=9.0, "Cycles"=1, "Mode Setting"="Heat Pump", "Flow Rate (GPM)"=3.0, "Temperature (F)"=58.0, "Reset Timer"=FALSE, "Use Temp Decline Method"=FALSE, "Terminate Condition"=enum."C9-Do Nothing", "Condition Value #1"=0.0, "UE"=FALSE, "LE"=FALSE, "Comp"=FALSE, "Fan"=FALSE, "Test End Time (Sec)"=0.0, "Purge Until Cutout"=FALSE, "Start Conditions"=enum."Wait for UE Cutout", "Condition Value #2"=0.0, "Remove Power"=FALSE, "Time"=3600.0, "Check Special Cond."=enum."SC1-Do Nothing", "Condition#"=enum."N/A", "Draw Flags"=enum."N/A", "Data Processing Delay (FHD 15sec, UEF 5 Sec)"=15.0, "Test Complete"=FALSE}, {"Sequence #"=10.0, "Cycles"=1, "Mode Setting"="", "Flow Rate (GPM)"=3.0, "Temperature (F)"=58.0, "Reset Timer"=FALSE, "Use Temp Decline Method"=FALSE, "Terminate Condition"=enum."C9-Do Nothing", "Condition Value #1"=0.0, "UE"=FALSE, "LE"=FALSE, "Comp"=FALSE, "Fan"=FALSE, "Test End Time (Sec)"=0.0, "Purge Until Cutout"=FALSE, "Start Conditions"=enum."Every X (Seconds)", "Condition Value #2"=300.0, "Remove Power"=FALSE, "Time"=3600.0, "Check Special Cond."=enum."SC1-Do Nothing", "Condition#"=enum."N/A", "Draw Flags"=enum."N/A", "Data Processing Delay (FHD 15sec, UEF 5 Sec)"=15.0, "Test Complete"=FALSE}, {"Sequence #"=11.0, "Cycles"=1, "Mode Setting"="", "Flow Rate (GPM)"=3.0, "Temperature (F)"=58.0, "Reset Timer"=FALSE, "Use Temp Decline Method"=FALSE, "Terminate Condition"=enum."C9-Do Nothing", "Condition Value #1"=0.0, "UE"=FALSE, "LE"=FALSE, "Comp"=FALSE, "Fan"=FALSE, "Test End Time (Sec)"=0.0, "Purge Until Cutout"=FALSE, "Start Conditions"=enum."Heat Source Cutout", "Condition Value #2"=0.0, "Remove Power"=FALSE, "Time"=3600.0, "Check Special Cond."=enum."SC1-Do Nothing", "Condition#"=enum."N/A", "Draw Flags"=enum."N/A", "Data Processing Delay (FHD 15sec, UEF 5 Sec)"=15.0, "Test Complete"=FALSE}, {"Sequence #"=12.0, "Cycles"=1, "Mode Setting"="", "Flow Rate (GPM)"=3.0, "Temperature (F)"=58.0, "Reset Timer"=FALSE, "Use Temp Decline Method"=FALSE, "Terminate Condition"=enum."C9-Do Nothing", "Condition Value #1"=0.0, "UE"=FALSE, "LE"=FALSE, "Comp"=FALSE, "Fan"=FALSE, "Test End Time (Sec)"=0.0, "Purge Until Cutout"=FALSE, "Start Conditions"=enum."Every X (Seconds)", "Condition Value #2"=1800.0, "Remove Power"=FALSE, "Time"=3600.0, "Check Special Cond."=enum."SC1-Do Nothing", "Condition#"=enum."N/A", "Draw Flags"=enum."N/A", "Data Processing Delay (FHD 15sec, UEF 5 Sec)"=15.0, "Test Complete"=FALSE}, {"Sequence #"=13.0, "Cycles"=1, "Mode Setting"="", "Flow Rate (GPM)"=3.0, "Temperature (F)"=58.0, "Reset Timer"=FALSE, "Use Temp Decline Method"=FALSE, "Terminate Condition"=enum."C9-Do Nothing", "Condition Value #1"=0.0, "UE"=FALSE, "LE"=FALSE, "Comp"=FALSE, "Fan"=FALSE, "Test End Time (Sec)"=0.0, "Purge Until Cutout"=FALSE, "Start Conditions"=enum."Heat Source Cutout", "Condition Value #2"=0.0, "Remove Power"=FALSE, "Time"=3600.0, "Check Special Cond."=enum."SC1-Do Nothing", "Condition#"=enum."N/A", "Draw Flags"=enum."N/A", "Data Processing Delay (FHD 15sec, UEF 5 Sec)"=15.0, "Test Complete"=TRUE}] {"Time" format="%<%H:%M:%S>t"}
  in  "Heat-Up Audit Test (50 Gallon)":T21[](array[typedef])=[{"Sequence #"=1.0, "Cycles"=1, "Mode Setting"="Heat Pump", "Flow Rate (GPM)"=3.0, "Temperature (F)"=120.0, "Reset Timer"=FALSE, "Use Temp Decline Method"=FALSE, "Terminate Condition"=enum."C1-Terminate Draw @ Gallon Mark", "Condition Value #1"=100.0, "UE"=FALSE, "LE"=FALSE, "Comp"=FALSE, "Fan"=FALSE, "Test End Time (Sec)"=0.0, "Purge Until Cutout"=FALSE, "Start Conditions"=enum."Heat Source Cutout", "Condition Value #2"=0.0, "Remove Power"=FALSE, "Time"=0.0, "Check Special Cond."=enum."SC1-Do Nothing", "Condition#"=enum."N/A", "Draw Flags"=enum."N/A", "Data Processing Delay (FHD 15sec, UEF 5 Sec)"=15.0, "Test Complete"=FALSE}, {"Sequence #"=2.0, "Cycles"=1, "Mode Setting"="Hybrid", "Flow Rate (GPM)"=1.7, "Temperature (F)"=58.0, "Reset Timer"=TRUE, "Use Temp Decline Method"=TRUE, "Terminate Condition"=enum."C1-Terminate Draw @ Gallon Mark", "Condition Value #1"=15.0, "UE"=FALSE, "LE"=FALSE, "Comp"=FALSE, "Fan"=FALSE, "Test End Time (Sec)"=0.0, "Purge Until Cutout"=FALSE, "Start Conditions"=enum."Heat Source Cutout", "Condition Value #2"=0.0, "Remove Power"=FALSE, "Time"=0.0, "Check Special Cond."=enum."SC1-Do Nothing", "Condition#"=enum."N/A", "Draw Flags"=enum."N/A", "Data Processing Delay (FHD 15sec, UEF 5 Sec)"=15.0, "Test Complete"=FALSE}, {"Sequence #"=3.0, "Cycles"=1, "Mode Setting"="", "Flow Rate (GPM)"=1.0, "Temperature (F)"=58.0, "Reset Timer"=FALSE, "Use Temp Decline Method"=FALSE, "Terminate Condition"=enum."C1-Terminate Draw @ Gallon Mark", "Condition Value #1"=2.0, "UE"=FALSE, "LE"=FALSE, "Comp"=FALSE, "Fan"=FALSE, "Test End Time (Sec)"=0.0, "Purge Until Cutout"=FALSE, "Start Conditions"=enum."At Time (Seconds)", "Condition Value #2"=1800.0, "Remove Power"=FALSE, "Time"=0.0, "Check Special Cond."=enum."SC1-Do Nothing", "Condition#"=enum."N/A", "Draw Flags"=enum."N/A", "Data Processing Delay (FHD 15sec, UEF 5 Sec)"=15.0, "Test Complete"=FALSE}, {"Sequence #"=4.0, "Cycles"=1, "Mode Setting"="", "Flow Rate (GPM)"=1.7, "Temperature (F)"=58.0, "Reset Timer"=FALSE, "Use Temp Decline Method"=FALSE, "Terminate Condition"=enum."C1-Terminate Draw @ Gallon Mark", "Condition Value #1"=9.0, "UE"=FALSE, "LE"=FALSE, "Comp"=FALSE, "Fan"=FALSE, "Test End Time (Sec)"=0.0, "Purge Until Cutout"=FALSE, "Start Conditions"=enum."At Time (Seconds)", "Condition Value #2"=6000.0, "Remove Power"=FALSE, "Time"=0.0, "Check Special Cond."=enum."SC1-Do Nothing", "Condition#"=enum."N/A", "Draw Flags"=enum."N/A", "Data Processing Delay (FHD 15sec, UEF 5 Sec)"=15.0, "Test Complete"=FALSE}, {"Sequence #"=5.0, "Cycles"=1, "Mode Setting"="", "Flow Rate (GPM)"=3.0, "Temperature (F)"=58.0, "Reset Timer"=FALSE, "Use Temp Decline Method"=FALSE, "Terminate Condition"=enum."C9-Do Nothing", "Condition Value #1"=0.0, "UE"=FALSE, "LE"=FALSE, "Comp"=FALSE, "Fan"=FALSE, "Test End Time (Sec)"=0.0, "Purge Until Cutout"=FALSE, "Start Conditions"=enum."Heat Source Cutout", "Condition Value #2"=0.0, "Remove Power"=FALSE, "Time"=0.0, "Check Special Cond."=enum."SC1-Do Nothing", "Condition#"=enum."N/A", "Draw Flags"=enum."N/A", "Data Processing Delay (FHD 15sec, UEF 5 Sec)"=15.0, "Test Complete"=FALSE}, {"Sequence #"=6.0, "Cycles"=1, "Mode Setting"="", "Flow Rate (GPM)"=3.0, "Temperature (F)"=58.0, "Reset Timer"=FALSE, "Use Temp Decline Method"=FALSE, "Terminate Condition"=enum."C8-Specific Heat Source", "Condition Value #1"=0.0, "UE"=TRUE, "LE"=FALSE, "Comp"=FALSE, "Fan"=FALSE, "Test End Time (Sec)"=0.0, "Purge Until Cutout"=FALSE, "Start Conditions"=enum."Every X (Seconds)", "Condition Value #2"=600.0, "Remove Power"=FALSE, "Time"=0.0, "Check Special Cond."=enum."SC1-Do Nothing", "Condition#"=enum."N/A", "Draw Flags"=enum."SmlMedLrg(7)", "Data Processing Delay (FHD 15sec, UEF 5 Sec)"=15.0, "Test Complete"=FALSE}, {"Sequence #"=7.0, "Cycles"=1, "Mode Setting"="", "Flow Rate (GPM)"=3.0, "Temperature (F)"=58.0, "Reset Timer"=FALSE, "Use Temp Decline Method"=FALSE, "Terminate Condition"=enum."C9-Do Nothing", "Condition Value #1"=0.0, "UE"=FALSE, "LE"=FALSE, "Comp"=FALSE, "Fan"=FALSE, "Test End Time (Sec)"=0.0, "Purge Until Cutout"=FALSE, "Start Conditions"=enum."Wait for UE Cutout", "Condition Value #2"=0.0, "Remove Power"=FALSE, "Time"=0.0, "Check Special Cond."=enum."SC1-Do Nothing", "Condition#"=enum."N/A", "Draw Flags"=enum."N/A", "Data Processing Delay (FHD 15sec, UEF 5 Sec)"=15.0, "Test Complete"=FALSE}, {"Sequence #"=8.0, "Cycles"=1, "Mode Setting"="", "Flow Rate (GPM)"=3.0, "Temperature (F)"=58.0, "Reset Timer"=FALSE, "Use Temp Decline Method"=FALSE, "Terminate Condition"=enum."C9-Do Nothing", "Condition Value #1"=0.0, "UE"=FALSE, "LE"=FALSE, "Comp"=FALSE, "Fan"=FALSE, "Test End Time (Sec)"=0.0, "Purge Until Cutout"=FALSE, "Start Conditions"=enum."Every X (Seconds)", "Condition Value #2"=300.0, "Remove Power"=FALSE, "Time"=0.0, "Check Special Cond."=enum."SC1-Do Nothing", "Condition#"=enum."N/A", "Draw Flags"=enum."N/A", "Data Processing Delay (FHD 15sec, UEF 5 Sec)"=15.0, "Test Complete"=FALSE}, {"Sequence #"=9.0, "Cycles"=1, "Mode Setting"="", "Flow Rate (GPM)"=3.0, "Temperature (F)"=58.0, "Reset Timer"=FALSE, "Use Temp Decline Method"=FALSE, "Terminate Condition"=enum."C9-Do Nothing", "Condition Value #1"=0.0, "UE"=FALSE, "LE"=FALSE, "Comp"=FALSE, "Fan"=FALSE, "Test End Time (Sec)"=0.0, "Purge Until Cutout"=FALSE, "Start Conditions"=enum."Heat Source Cutout", "Condition Value #2"=0.0, "Remove Power"=FALSE, "Time"=0.0, "Check Special Cond."=enum."SC1-Do Nothing", "Condition#"=enum."N/A", "Draw Flags"=enum."N/A", "Data Processing Delay (FHD 15sec, UEF 5 Sec)"=15.0, "Test Complete"=FALSE}, {"Sequence #"=10.0, "Cycles"=1, "Mode Setting"="", "Flow Rate (GPM)"=3.0, "Temperature (F)"=58.0, "Reset Timer"=FALSE, "Use Temp Decline Method"=FALSE, "Terminate Condition"=enum."C9-Do Nothing", "Condition Value #1"=0.0, "UE"=FALSE, "LE"=FALSE, "Comp"=FALSE, "Fan"=FALSE, "Test End Time (Sec)"=0.0, "Purge Until Cutout"=FALSE, "Start Conditions"=enum."Every X (Seconds)", "Condition Value #2"=1800.0, "Remove Power"=FALSE, "Time"=0.0, "Check Special Cond."=enum."SC1-Do Nothing", "Condition#"=enum."N/A", "Draw Flags"=enum."N/A", "Data Processing Delay (FHD 15sec, UEF 5 Sec)"=15.0, "Test Complete"=FALSE}, {"Sequence #"=11.0, "Cycles"=1, "Mode Setting"="", "Flow Rate (GPM)"=3.0, "Temperature (F)"=58.0, "Reset Timer"=FALSE, "Use Temp Decline Method"=FALSE, "Terminate Condition"=enum."C9-Do Nothing", "Condition Value #1"=0.0, "UE"=FALSE, "LE"=FALSE, "Comp"=FALSE, "Fan"=FALSE, "Test End Time (Sec)"=0.0, "Purge Until Cutout"=FALSE, "Start Conditions"=enum."Heat Source Cutout", "Condition Value #2"=0.0, "Remove Power"=FALSE, "Time"=0.0, "Check Special Cond."=enum."SC1-Do Nothing", "Condition#"=enum."N/A", "Draw Flags"=enum."N/A", "Data Processing Delay (FHD 15sec, UEF 5 Sec)"=15.0, "Test Complete"=TRUE}] {"Time" format="%<%H:%M:%S>t"}
  in  "Heat-Up Audit Test (50 Gallon) Heat Pump":T21[](array[typedef])=[{"Sequence #"=1.0, "Cycles"=1, "Mode Setting"="Heat Pump", "Flow Rate (GPM)"=3.0, "Temperature (F)"=120.0, "Reset Timer"=FALSE, "Use Temp Decline Method"=FALSE, "Terminate Condition"=enum."C1-Terminate Draw @ Gallon Mark", "Condition Value #1"=100.0, "UE"=FALSE, "LE"=FALSE, "Comp"=FALSE, "Fan"=FALSE, "Test End Time (Sec)"=0.0, "Purge Until Cutout"=FALSE, "Start Conditions"=enum."Heat Source Cutout", "Condition Value #2"=0.0, "Remove Power"=FALSE, "Time"=0.0, "Check Special Cond."=enum."SC1-Do Nothing", "Condition#"=enum."N/A", "Draw Flags"=enum."N/A", "Data Processing Delay (FHD 15sec, UEF 5 Sec)"=15.0, "Test Complete"=FALSE}, {"Sequence #"=2.0, "Cycles"=1, "Mode Setting"="Hybrid", "Flow Rate (GPM)"=1.7, "Temperature (F)"=58.0, "Reset Timer"=TRUE, "Use Temp Decline Method"=TRUE, "Terminate Condition"=enum."C1-Terminate Draw @ Gallon Mark", "Condition Value #1"=15.0, "UE"=FALSE, "LE"=FALSE, "Comp"=FALSE, "Fan"=FALSE, "Test End Time (Sec)"=0.0, "Purge Until Cutout"=FALSE, "Start Conditions"=enum."Heat Source Cutout", "Condition Value #2"=0.0, "Remove Power"=FALSE, "Time"=0.0, "Check Special Cond."=enum."SC1-Do Nothing", "Condition#"=enum."N/A", "Draw Flags"=enum."N/A", "Data Processing Delay (FHD 15sec, UEF 5 Sec)"=15.0, "Test Complete"=FALSE}, {"Sequence #"=3.0, "Cycles"=1, "Mode Setting"="", "Flow Rate (GPM)"=1.0, "Temperature (F)"=58.0, "Reset Timer"=FALSE, "Use Temp Decline Method"=FALSE, "Terminate Condition"=enum."C1-Terminate Draw @ Gallon Mark", "Condition Value #1"=2.0, "UE"=FALSE, "LE"=FALSE, "Comp"=FALSE, "Fan"=FALSE, "Test End Time (Sec)"=0.0, "Purge Until Cutout"=FALSE, "Start Conditions"=enum."At Time (Seconds)", "Condition Value #2"=1800.0, "Remove Power"=FALSE, "Time"=0.0, "Check Special Cond."=enum."SC1-Do Nothing", "Condition#"=enum."N/A", "Draw Flags"=enum."N/A", "Data Processing Delay (FHD 15sec, UEF 5 Sec)"=15.0, "Test Complete"=FALSE}, {"Sequence #"=4.0, "Cycles"=1, "Mode Setting"="", "Flow Rate (GPM)"=1.7, "Temperature (F)"=58.0, "Reset Timer"=FALSE, "Use Temp Decline Method"=FALSE, "Terminate Condition"=enum."C1-Terminate Draw @ Gallon Mark", "Condition Value #1"=9.0, "UE"=FALSE, "LE"=FALSE, "Comp"=FALSE, "Fan"=FALSE, "Test End Time (Sec)"=0.0, "Purge Until Cutout"=FALSE, "Start Conditions"=enum."At Time (Seconds)", "Condition Value #2"=6000.0, "Remove Power"=FALSE, "Time"=0.0, "Check Special Cond."=enum."SC1-Do Nothing", "Condition#"=enum."N/A", "Draw Flags"=enum."N/A", "Data Processing Delay (FHD 15sec, UEF 5 Sec)"=15.0, "Test Complete"=FALSE}, {"Sequence #"=5.0, "Cycles"=1, "Mode Setting"="", "Flow Rate (GPM)"=3.0, "Temperature (F)"=58.0, "Reset Timer"=FALSE, "Use Temp Decline Method"=FALSE, "Terminate Condition"=enum."C9-Do Nothing", "Condition Value #1"=0.0, "UE"=FALSE, "LE"=FALSE, "Comp"=FALSE, "Fan"=FALSE, "Test End Time (Sec)"=0.0, "Purge Until Cutout"=FALSE, "Start Conditions"=enum."Heat Source Cutout", "Condition Value #2"=0.0, "Remove Power"=FALSE, "Time"=0.0, "Check Special Cond."=enum."SC1-Do Nothing", "Condition#"=enum."N/A", "Draw Flags"=enum."N/A", "Data Processing Delay (FHD 15sec, UEF 5 Sec)"=15.0, "Test Complete"=FALSE}, {"Sequence #"=6.0, "Cycles"=1, "Mode Setting"="", "Flow Rate (GPM)"=3.0, "Temperature (F)"=58.0, "Reset Timer"=FALSE, "Use Temp Decline Method"=FALSE, "Terminate Condition"=enum."C1-Terminate Draw @ Gallon Mark", "Condition Value #1"=40.0, "UE"=FALSE, "LE"=FALSE, "Comp"=FALSE, "Fan"=FALSE, "Test End Time (Sec)"=0.0, "Purge Until Cutout"=FALSE, "Start Conditions"=enum."Every X (Seconds)", "Condition Value #2"=600.0, "Remove Power"=FALSE, "Time"=0.0, "Check Special Cond."=enum."SC1-Do Nothing", "Condition#"=enum."N/A", "Draw Flags"=enum."N/A", "Data Processing Delay (FHD 15sec, UEF 5 Sec)"=15.0, "Test Complete"=FALSE}, {"Sequence #"=7.0, "Cycles"=1, "Mode Setting"="", "Flow Rate (GPM)"=3.0, "Temperature (F)"=58.0, "Reset Timer"=FALSE, "Use Temp Decline Method"=FALSE, "Terminate Condition"=enum."C9-Do Nothing", "Condition Value #1"=0.0, "UE"=FALSE, "LE"=FALSE, "Comp"=FALSE, "Fan"=FALSE, "Test End Time (Sec)"=0.0, "Purge Until Cutout"=FALSE, "Start Conditions"=enum."Heat Source Cutout", "Condition Value #2"=0.0, "Remove Power"=FALSE, "Time"=0.0, "Check Special Cond."=enum."SC1-Do Nothing", "Condition#"=enum."N/A", "Draw Flags"=enum."N/A", "Data Processing Delay (FHD 15sec, UEF 5 Sec)"=15.0, "Test Complete"=FALSE}, {"Sequence #"=8.0, "Cycles"=1, "Mode Setting"="", "Flow Rate (GPM)"=3.0, "Temperature (F)"=58.0, "Reset Timer"=FALSE, "Use Temp Decline Method"=FALSE, "Terminate Condition"=enum."C9-Do Nothing", "Condition Value #1"=0.0, "UE"=FALSE, "LE"=FALSE, "Comp"=FALSE, "Fan"=FALSE, "Test End Time (Sec)"=0.0, "Purge Until Cutout"=FALSE, "Start Conditions"=enum."Every X (Seconds)", "Condition Value #2"=300.0, "Remove Power"=FALSE, "Time"=0.0, "Check Special Cond."=enum."SC1-Do Nothing", "Condition#"=enum."N/A", "Draw Flags"=enum."N/A", "Data Processing Delay (FHD 15sec, UEF 5 Sec)"=15.0, "Test Complete"=FALSE}, {"Sequence #"=9.0, "Cycles"=1, "Mode Setting"="", "Flow Rate (GPM)"=3.0, "Temperature (F)"=58.0, "Reset Timer"=FALSE, "Use Temp Decline Method"=FALSE, "Terminate Condition"=enum."C9-Do Nothing", "Condition Value #1"=0.0, "UE"=FALSE, "LE"=FALSE, "Comp"=FALSE, "Fan"=FALSE, "Test End Time (Sec)"=0.0, "Purge Until Cutout"=FALSE, "Start Conditions"=enum."Every X (Seconds)", "Condition Value #2"=1800.0, "Remove Power"=FALSE, "Time"=0.0, "Check Special Cond."=enum."SC1-Do Nothing", "Condition#"=enum."N/A", "Draw Flags"=enum."N/A", "Data Processing Delay (FHD 15sec, UEF 5 Sec)"=15.0, "Test Complete"=FALSE}, {"Sequence #"=10.0, "Cycles"=1, "Mode Setting"="", "Flow Rate (GPM)"=3.0, "Temperature (F)"=58.0, "Reset Timer"=FALSE, "Use Temp Decline Method"=FALSE, "Terminate Condition"=enum."C9-Do Nothing", "Condition Value #1"=0.0, "UE"=FALSE, "LE"=FALSE, "Comp"=FALSE, "Fan"=FALSE, "Test End Time (Sec)"=0.0, "Purge Until Cutout"=FALSE, "Start Conditions"=enum."Heat Source Cutout", "Condition Value #2"=0.0, "Remove Power"=FALSE, "Time"=0.0, "Check Special Cond."=enum."SC1-Do Nothing", "Condition#"=enum."N/A", "Draw Flags"=enum."N/A", "Data Processing Delay (FHD 15sec, UEF 5 Sec)"=15.0, "Test Complete"=TRUE}] {"Time" format="%<%H:%M:%S>t"}
  in  "Heat-Up Audit Test (80 Gallon)":T21[](array[typedef])=[{"Sequence #"=1.0, "Cycles"=1, "Mode Setting"="Heat Pump", "Flow Rate (GPM)"=3.0, "Temperature (F)"=120.0, "Reset Timer"=FALSE, "Use Temp Decline Method"=FALSE, "Terminate Condition"=enum."C1-Terminate Draw @ Gallon Mark", "Condition Value #1"=100.0, "UE"=FALSE, "LE"=FALSE, "Comp"=FALSE, "Fan"=FALSE, "Test End Time (Sec)"=0.0, "Purge Until Cutout"=FALSE, "Start Conditions"=enum."Heat Source Cutout", "Condition Value #2"=0.0, "Remove Power"=FALSE, "Time"=0.0, "Check Special Cond."=enum."SC1-Do Nothing", "Condition#"=enum."N/A", "Draw Flags"=enum."N/A", "Data Processing Delay (FHD 15sec, UEF 5 Sec)"=15.0, "Test Complete"=FALSE}, {"Sequence #"=2.0, "Cycles"=1, "Mode Setting"="Hybrid", "Flow Rate (GPM)"=3.0, "Temperature (F)"=58.0, "Reset Timer"=TRUE, "Use Temp Decline Method"=TRUE, "Terminate Condition"=enum."C1-Terminate Draw @ Gallon Mark", "Condition Value #1"=27.0, "UE"=FALSE, "LE"=FALSE, "Comp"=FALSE, "Fan"=FALSE, "Test End Time (Sec)"=0.0, "Purge Until Cutout"=FALSE, "Start Conditions"=enum."At Time (Seconds)", "Condition Value #2"=0.0, "Remove Power"=FALSE, "Time"=0.0, "Check Special Cond."=enum."SC1-Do Nothing", "Condition#"=enum."N/A", "Draw Flags"=enum."N/A", "Data Processing Delay (FHD 15sec, UEF 5 Sec)"=15.0, "Test Complete"=FALSE}, {"Sequence #"=3.0, "Cycles"=1, "Mode Setting"="", "Flow Rate (GPM)"=1.0, "Temperature (F)"=58.0, "Reset Timer"=FALSE, "Use Temp Decline Method"=FALSE, "Terminate Condition"=enum."C1-Terminate Draw @ Gallon Mark", "Condition Value #1"=2.0, "UE"=FALSE, "LE"=FALSE, "Comp"=FALSE, "Fan"=FALSE, "Test End Time (Sec)"=0.0, "Purge Until Cutout"=FALSE, "Start Conditions"=enum."At Time (Seconds)", "Condition Value #2"=1800.0, "Remove Power"=FALSE, "Time"=0.0, "Check Special Cond."=enum."SC1-Do Nothing", "Condition#"=enum."N/A", "Draw Flags"=enum."N/A", "Data Processing Delay (FHD 15sec, UEF 5 Sec)"=15.0, "Test Complete"=FALSE}, {"Sequence #"=4.0, "Cycles"=1, "Mode Setting"="", "Flow Rate (GPM)"=1.0, "Temperature (F)"=58.0, "Reset Timer"=FALSE, "Use Temp Decline Method"=FALSE, "Terminate Condition"=enum."C1-Terminate Draw @ Gallon Mark", "Condition Value #1"=1.0, "UE"=FALSE, "LE"=FALSE, "Comp"=FALSE, "Fan"=FALSE, "Test End Time (Sec)"=0.0, "Purge Until Cutout"=FALSE, "Start Conditions"=enum."At Time (Seconds)", "Condition Value #2"=2400.0, "Remove Power"=FALSE, "Time"=0.0, "Check Special Cond."=enum."SC1-Do Nothing", "Condition#"=enum."N/A", "Draw Flags"=enum."N/A", "Data Processing Delay (FHD 15sec, UEF 5 Sec)"=15.0, "Test Complete"=FALSE}, {"Sequence #"=5.0, "Cycles"=1, "Mode Setting"="", "Flow Rate (GPM)"=1.7, "Temperature (F)"=58.0, "Reset Timer"=FALSE, "Use Temp Decline Method"=FALSE, "Terminate Condition"=enum."C1-Terminate Draw @ Gallon Mark", "Condition Value #1"=9.0, "UE"=FALSE, "LE"=FALSE, "Comp"=FALSE, "Fan"=FALSE, "Test End Time (Sec)"=0.0, "Purge Until Cutout"=FALSE, "Start Conditions"=enum."At Time (Seconds)", "Condition Value #2"=6000.0, "Remove Power"=FALSE, "Time"=0.0, "Check Special Cond."=enum."SC1-Do Nothing", "Condition#"=enum."N/A", "Draw Flags"=enum."N/A", "Data Processing Delay (FHD 15sec, UEF 5 Sec)"=15.0, "Test Complete"=FALSE}, {"Sequence #"=6.0, "Cycles"=1, "Mode Setting"="", "Flow Rate (GPM)"=3.0, "Temperature (F)"=58.0, "Reset Timer"=FALSE, "Use Temp Decline Method"=FALSE, "Terminate Condition"=enum."C9-Do Nothing", "Condition Value #1"=0.0, "UE"=FALSE, "LE"=FALSE, "Comp"=FALSE, "Fan"=FALSE, "Test End Time (Sec)"=0.0, "Purge Until Cutout"=FALSE, "Start Conditions"=enum."Heat Source Cutout", "Condition Value #2"=0.0, "Remove Power"=FALSE, "Time"=0.0, "Check Special Cond."=enum."SC1-Do Nothing", "Condition#"=enum."N/A", "Draw Flags"=enum."N/A", "Data Processing Delay (FHD 15sec, UEF 5 Sec)"=15.0, "Test Complete"=FALSE}, {"Sequence #"=7.0, "Cycles"=1, "Mode Setting"="", "Flow Rate (GPM)"=3.0, "Temperature (F)"=58.0, "Reset Timer"=FALSE, "Use Temp Decline Method"=FALSE, "Terminate Condition"=enum."C8-Specific Heat Source", "Condition Value #1"=0.0, "UE"=TRUE, "LE"=FALSE, "Comp"=FALSE, "Fan"=FALSE, "Test End Time (Sec)"=0.0, "Purge Until Cutout"=FALSE, "Start Conditions"=enum."Every X (Seconds)", "Condition Value #2"=600.0, "Remove Power"=FALSE, "Time"=0.0, "Check Special Cond."=enum."SC1-Do Nothing", "Condition#"=enum."N/A", "Draw Flags"=enum."SmlMedLrg(7)", "Data Processing Delay (FHD 15sec, UEF 5 Sec)"=15.0, "Test Complete"=FALSE}, {"Sequence #"=8.0, "Cycles"=1, "Mode Setting"="", "Flow Rate (GPM)"=3.0, "Temperature (F)"=58.0, "Reset Timer"=FALSE, "Use Temp Decline Method"=FALSE, "Terminate Condition"=enum."C9-Do Nothing", "Condition Value #1"=0.0, "UE"=FALSE, "LE"=FALSE, "Comp"=FALSE, "Fan"=FALSE, "Test End Time (Sec)"=0.0, "Purge Until Cutout"=FALSE, "Start Conditions"=enum."Wait for UE Cutout", "Condition Value #2"=0.0, "Remove Power"=FALSE, "Time"=0.0, "Check Special Cond."=enum."SC1-Do Nothing", "Condition#"=enum."N/A", "Draw Flags"=enum."N/A", "Data Processing Delay (FHD 15sec, UEF 5 Sec)"=15.0, "Test Complete"=FALSE}, {"Sequence #"=9.0, "Cycles"=1, "Mode Setting"="", "Flow Rate (GPM)"=3.0, "Temperature (F)"=58.0, "Reset Timer"=FALSE, "Use Temp Decline Method"=FALSE, "Terminate Condition"=enum."C9-Do Nothing", "Condition Value #1"=0.0, "UE"=FALSE, "LE"=FALSE, "Comp"=FALSE, "Fan"=FALSE, "Test End Time (Sec)"=0.0, "Purge Until Cutout"=FALSE, "Start Conditions"=enum."Every X (Seconds)", "Condition Value #2"=300.0, "Remove Power"=FALSE, "Time"=0.0, "Check Special Cond."=enum."SC1-Do Nothing", "Condition#"=enum."N/A", "Draw Flags"=enum."N/A", "Data Processing Delay (FHD 15sec, UEF 5 Sec)"=15.0, "Test Complete"=FALSE}, {"Sequence #"=10.0, "Cycles"=1, "Mode Setting"="", "Flow Rate (GPM)"=3.0, "Temperature (F)"=58.0, "Reset Timer"=FALSE, "Use Temp Decline Method"=FALSE, "Terminate Condition"=enum."C8-Specific Heat Source", "Condition Value #1"=0.0, "UE"=FALSE, "LE"=FALSE, "Comp"=FALSE, "Fan"=FALSE, "Test End Time (Sec)"=0.0, "Purge Until Cutout"=FALSE, "Start Conditions"=enum."Heat Source Cutout", "Condition Value #2"=0.0, "Remove Power"=FALSE, "Time"=0.0, "Check Special Cond."=enum."SC1-Do Nothing", "Condition#"=enum."N/A", "Draw Flags"=enum."N/A", "Data Processing Delay (FHD 15sec, UEF 5 Sec)"=15.0, "Test Complete"=FALSE}, {"Sequence #"=11.0, "Cycles"=1, "Mode Setting"="", "Flow Rate (GPM)"=3.0, "Temperature (F)"=58.0, "Reset Timer"=FALSE, "Use Temp Decline Method"=FALSE, "Terminate Condition"=enum."C9-Do Nothing", "Condition Value #1"=0.0, "UE"=FALSE, "LE"=FALSE, "Comp"=FALSE, "Fan"=FALSE, "Test End Time (Sec)"=0.0, "Purge Until Cutout"=FALSE, "Start Conditions"=enum."Every X (Seconds)", "Condition Value #2"=1800.0, "Remove Power"=FALSE, "Time"=0.0, "Check Special Cond."=enum."SC1-Do Nothing", "Condition#"=enum."N/A", "Draw Flags"=enum."N/A", "Data Processing Delay (FHD 15sec, UEF 5 Sec)"=15.0, "Test Complete"=FALSE}, {"Sequence #"=12.0, "Cycles"=1, "Mode Setting"="", "Flow Rate (GPM)"=3.0, "Temperature (F)"=58.0, "Reset Timer"=FALSE, "Use Temp Decline Method"=FALSE, "Terminate Condition"=enum."C9-Do Nothing", "Condition Value #1"=0.0, "UE"=FALSE, "LE"=FALSE, "Comp"=FALSE, "Fan"=FALSE, "Test End Time (Sec)"=0.0, "Purge Until Cutout"=FALSE, "Start Conditions"=enum."Heat Source Cutout", "Condition Value #2"=0.0, "Remove Power"=FALSE, "Time"=0.0, "Check Special Cond."=enum."SC1-Do Nothing", "Condition#"=enum."N/A", "Draw Flags"=enum."N/A", "Data Processing Delay (FHD 15sec, UEF 5 Sec)"=15.0, "Test Complete"=TRUE}] {"Time" format="%<%H:%M:%S>t"}
  in  "Heat-Up Audit Test - Heat Pump (80 Gallon)":T21[](array[typedef])=[{"Sequence #"=1.0, "Cycles"=1, "Mode Setting"="Heat Pump", "Flow Rate (GPM)"=3.0, "Temperature (F)"=120.0, "Reset Timer"=FALSE, "Use Temp Decline Method"=FALSE, "Terminate Condition"=enum."C1-Terminate Draw @ Gallon Mark", "Condition Value #1"=100.0, "UE"=FALSE, "LE"=FALSE, "Comp"=FALSE, "Fan"=FALSE, "Test End Time (Sec)"=0.0, "Purge Until Cutout"=FALSE, "Start Conditions"=enum."Heat Source Cutout", "Condition Value #2"=0.0, "Remove Power"=FALSE, "Time"=0.0, "Check Special Cond."=enum."SC1-Do Nothing", "Condition#"=enum."N/A", "Draw Flags"=enum."N/A", "Data Processing Delay (FHD 15sec, UEF 5 Sec)"=15.0, "Test Complete"=FALSE}, {"Sequence #"=2.0, "Cycles"=1, "Mode Setting"="Hybrid", "Flow Rate (GPM)"=3.0, "Temperature (F)"=58.0, "Reset Timer"=TRUE, "Use Temp Decline Method"=TRUE, "Terminate Condition"=enum."C1-Terminate Draw @ Gallon Mark", "Condition Value #1"=27.0, "UE"=FALSE, "LE"=FALSE, "Comp"=FALSE, "Fan"=FALSE, "Test End Time (Sec)"=0.0, "Purge Until Cutout"=FALSE, "Start Conditions"=enum."At Time (Seconds)", "Condition Value #2"=0.0, "Remove Power"=FALSE, "Time"=0.0, "Check Special Cond."=enum."SC1-Do Nothing", "Condition#"=enum."N/A", "Draw Flags"=enum."N/A", "Data Processing Delay (FHD 15sec, UEF 5 Sec)"=15.0, "Test Complete"=FALSE}, {"Sequence #"=3.0, "Cycles"=1, "Mode Setting"="", "Flow Rate (GPM)"=1.0, "Temperature (F)"=58.0, "Reset Timer"=FALSE, "Use Temp Decline Method"=FALSE, "Terminate Condition"=enum."C1-Terminate Draw @ Gallon Mark", "Condition Value #1"=2.0, "UE"=FALSE, "LE"=FALSE, "Comp"=FALSE, "Fan"=FALSE, "Test End Time (Sec)"=0.0, "Purge Until Cutout"=FALSE, "Start Conditions"=enum."At Time (Seconds)", "Condition Value #2"=1800.0, "Remove Power"=FALSE, "Time"=0.0, "Check Special Cond."=enum."SC1-Do Nothing", "Condition#"=enum."N/A", "Draw Flags"=enum."N/A", "Data Processing Delay (FHD 15sec, UEF 5 Sec)"=15.0, "Test Complete"=FALSE}, {"Sequence #"=4.0, "Cycles"=1, "Mode Setting"="", "Flow Rate (GPM)"=1.0, "Temperature (F)"=58.0, "Reset Timer"=FALSE, "Use Temp Decline Method"=FALSE, "Terminate Condition"=enum."C1-Terminate Draw @ Gallon Mark", "Condition Value #1"=1.0, "UE"=FALSE, "LE"=FALSE, "Comp"=FALSE, "Fan"=FALSE, "Test End Time (Sec)"=0.0, "Purge Until Cutout"=FALSE, "Start Conditions"=enum."At Time (Seconds)", "Condition Value #2"=2400.0, "Remove Power"=FALSE, "Time"=0.0, "Check Special Cond."=enum."SC1-Do Nothing", "Condition#"=enum."N/A", "Draw Flags"=enum."N/A", "Data Processing Delay (FHD 15sec, UEF 5 Sec)"=15.0, "Test Complete"=FALSE}, {"Sequence #"=5.0, "Cycles"=1, "Mode Setting"="", "Flow Rate (GPM)"=1.7, "Temperature (F)"=58.0, "Reset Timer"=FALSE, "Use Temp Decline Method"=FALSE, "Terminate Condition"=enum."C1-Terminate Draw @ Gallon Mark", "Condition Value #1"=9.0, "UE"=FALSE, "LE"=FALSE, "Comp"=FALSE, "Fan"=FALSE, "Test End Time (Sec)"=0.0, "Purge Until Cutout"=FALSE, "Start Conditions"=enum."At Time (Seconds)", "Condition Value #2"=6000.0, "Remove Power"=FALSE, "Time"=0.0, "Check Special Cond."=enum."SC1-Do Nothing", "Condition#"=enum."N/A", "Draw Flags"=enum."N/A", "Data Processing Delay (FHD 15sec, UEF 5 Sec)"=15.0, "Test Complete"=FALSE}, {"Sequence #"=6.0, "Cycles"=1, "Mode Setting"="", "Flow Rate (GPM)"=3.0, "Temperature (F)"=58.0, "Reset Timer"=FALSE, "Use Temp Decline Method"=FALSE, "Terminate Condition"=enum."C9-Do Nothing", "Condition Value #1"=0.0, "UE"=FALSE, "LE"=FALSE, "Comp"=FALSE, "Fan"=FALSE, "Test End Time (Sec)"=0.0, "Purge Until Cutout"=FALSE, "Start Conditions"=enum."Heat Source Cutout", "Condition Value #2"=0.0, "Remove Power"=FALSE, "Time"=0.0, "Check Special Cond."=enum."SC1-Do Nothing", "Condition#"=enum."N/A", "Draw Flags"=enum."N/A", "Data Processing Delay (FHD 15sec, UEF 5 Sec)"=15.0, "Test Complete"=FALSE}, {"Sequence #"=7.0, "Cycles"=1, "Mode Setting"="", "Flow Rate (GPM)"=3.0, "Temperature (F)"=58.0, "Reset Timer"=FALSE, "Use Temp Decline Method"=FALSE, "Terminate Condition"=enum."C1-Terminate Draw @ Gallon Mark", "Condition Value #1"=40.0, "UE"=FALSE, "LE"=FALSE, "Comp"=FALSE, "Fan"=FALSE, "Test End Time (Sec)"=0.0, "Purge Until Cutout"=FALSE, "Start Conditions"=enum."Every X (Seconds)", "Condition Value #2"=600.0, "Remove Power"=FALSE, "Time"=0.0, "Check Special Cond."=enum."SC1-Do Nothing", "Condition#"=enum."N/A", "Draw Flags"=enum."SmlMedLrg(7)", "Data Processing Delay (FHD 15sec, UEF 5 Sec)"=15.0, "Test Complete"=FALSE}, {"Sequence #"=8.0, "Cycles"=1, "Mode Setting"="", "Flow Rate (GPM)"=3.0, "Temperature (F)"=58.0, "Reset Timer"=FALSE, "Use Temp Decline Method"=FALSE, "Terminate Condition"=enum."C9-Do Nothing", "Condition Value #1"=0.0, "UE"=FALSE, "LE"=FALSE, "Comp"=FALSE, "Fan"=FALSE, "Test End Time (Sec)"=0.0, "Purge Until Cutout"=FALSE, "Start Conditions"=enum."Heat Source Cutout", "Condition Value #2"=0.0, "Remove Power"=FALSE, "Time"=0.0, "Check Special Cond."=enum."SC1-Do Nothing", "Condition#"=enum."N/A", "Draw Flags"=enum."N/A", "Data Processing Delay (FHD 15sec, UEF 5 Sec)"=15.0, "Test Complete"=FALSE}, {"Sequence #"=9.0, "Cycles"=1, "Mode Setting"="", "Flow Rate (GPM)"=3.0, "Temperature (F)"=58.0, "Reset Timer"=FALSE, "Use Temp Decline Method"=FALSE, "Terminate Condition"=enum."C9-Do Nothing", "Condition Value #1"=0.0, "UE"=FALSE, "LE"=FALSE, "Comp"=FALSE, "Fan"=FALSE, "Test End Time (Sec)"=0.0, "Purge Until Cutout"=FALSE, "Start Conditions"=enum."Every X (Seconds)", "Condition Value #2"=300.0, "Remove Power"=FALSE, "Time"=0.0, "Check Special Cond."=enum."SC1-Do Nothing", "Condition#"=enum."N/A", "Draw Flags"=enum."N/A", "Data Processing Delay (FHD 15sec, UEF 5 Sec)"=15.0, "Test Complete"=FALSE}, {"Sequence #"=10.0, "Cycles"=1, "Mode Setting"="", "Flow Rate (GPM)"=3.0, "Temperature (F)"=58.0, "Reset Timer"=FALSE, "Use Temp Decline Method"=FALSE, "Terminate Condition"=enum."C9-Do Nothing", "Condition Value #1"=0.0, "UE"=FALSE, "LE"=FALSE, "Comp"=FALSE, "Fan"=FALSE, "Test End Time (Sec)"=0.0, "Purge Until Cutout"=FALSE, "Start Conditions"=enum."Every X (Seconds)", "Condition Value #2"=1800.0, "Remove Power"=FALSE, "Time"=0.0, "Check Special Cond."=enum."SC1-Do Nothing", "Condition#"=enum."N/A", "Draw Flags"=enum."N/A", "Data Processing Delay (FHD 15sec, UEF 5 Sec)"=15.0, "Test Complete"=FALSE}, {"Sequence #"=11.0, "Cycles"=1, "Mode Setting"="", "Flow Rate (GPM)"=3.0, "Temperature (F)"=58.0, "Reset Timer"=FALSE, "Use Temp Decline Method"=FALSE, "Terminate Condition"=enum."C9-Do Nothing", "Condition Value #1"=0.0, "UE"=FALSE, "LE"=FALSE, "Comp"=FALSE, "Fan"=FALSE, "Test End Time (Sec)"=0.0, "Purge Until Cutout"=FALSE, "Start Conditions"=enum."Heat Source Cutout", "Condition Value #2"=0.0, "Remove Power"=FALSE, "Time"=0.0, "Check Special Cond."=enum."SC1-Do Nothing", "Condition#"=enum."N/A", "Draw Flags"=enum."N/A", "Data Processing Delay (FHD 15sec, UEF 5 Sec)"=15.0, "Test Complete"=TRUE}] {"Time" format="%<%H:%M:%S>t"}
  in  "RLT":T21[](array[typedef])=[{"Sequence #"=1.0, "Cycles"=1000, "Mode Setting"="Hybrid", "Flow Rate (GPM)"=3.0, "Temperature (F)"=58.0, "Reset Timer"=FALSE, "Use Temp Decline Method"=FALSE, "Terminate Condition"=enum."C1-Terminate Draw @ Gallon Mark", "Condition Value #1"=35.0, "UE"=FALSE, "LE"=FALSE, "Comp"=FALSE, "Fan"=FALSE, "Test End Time (Sec)"=0.0, "Purge Until Cutout"=FALSE, "Start Conditions"=enum."Heat Source Cutout", "Condition Value #2"=0.0, "Remove Power"=FALSE, "Time"=0.0, "Check Special Cond."=enum."SC1-Do Nothing", "Condition#"=enum."N/A", "Draw Flags"=enum."N/A", "Data Processing Delay (FHD 15sec, UEF 5 Sec)"=15.0, "Test Complete"=FALSE}, {"Sequence #"=2.0, "Cycles"=1000, "Mode Setting"="Standard", "Flow Rate (GPM)"=3.0, "Temperature (F)"=58.0, "Reset Timer"=FALSE, "Use Temp Decline Method"=FALSE, "Terminate Condition"=enum."C1-Terminate Draw @ Gallon Mark", "Condition Value #1"=35.0, "UE"=FALSE, "LE"=FALSE, "Comp"=FALSE, "Fan"=FALSE, "Test End Time (Sec)"=0.0, "Purge Until Cutout"=FALSE, "Start Conditions"=enum."Heat Source Cutout", "Condition Value #2"=0.0, "Remove Power"=FALSE, "Time"=0.0, "Check Special Cond."=enum."SC1-Do Nothing", "Condition#"=enum."N/A", "Draw Flags"=enum."N/A", "Data Processing Delay (FHD 15sec, UEF 5 Sec)"=15.0, "Test Complete"=FALSE}, {"Sequence #"=3.0, "Cycles"=1, "Mode Setting"="", "Flow Rate (GPM)"=3.0, "Temperature (F)"=58.0, "Reset Timer"=FALSE, "Use Temp Decline Method"=FALSE, "Terminate Condition"=enum."C9-Do Nothing", "Condition Value #1"=0.0, "UE"=FALSE, "LE"=FALSE, "Comp"=FALSE, "Fan"=FALSE, "Test End Time (Sec)"=0.0, "Purge Until Cutout"=FALSE, "Start Conditions"=enum."Heat Source Cutout", "Condition Value #2"=0.0, "Remove Power"=FALSE, "Time"=0.0, "Check Special Cond."=enum."SC1-Do Nothing", "Condition#"=enum."N/A", "Draw Flags"=enum."N/A", "Data Processing Delay (FHD 15sec, UEF 5 Sec)"=0.0, "Test Complete"=TRUE}] {"Time" format="%<%H:%M:%S>t"}
  in  "2.5 Years Standard":T21[](array[typedef])=[{"Sequence #"=1.0, "Cycles"=4, "Mode Setting"="Hybrid", "Flow Rate (GPM)"=3.0, "Temperature (F)"=58.0, "Reset Timer"=FALSE, "Use Temp Decline Method"=FALSE, "Terminate Condition"=enum."C1-Terminate Draw @ Gallon Mark", "Condition Value #1"=35.0, "UE"=FALSE, "LE"=FALSE, "Comp"=FALSE, "Fan"=FALSE, "Test End Time (Sec)"=0.0, "Purge Until Cutout"=FALSE, "Start Conditions"=enum."Heat Source Cutout", "Condition Value #2"=0.0, "Remove Power"=FALSE, "Time"=0.0, "Check Special Cond."=enum."SC1-Do Nothing", "Condition#"=enum."N/A", "Draw Flags"=enum."N/A", "Data Processing Delay (FHD 15sec, UEF 5 Sec)"=15.0, "Test Complete"=FALSE}, {"Sequence #"=2.0, "Cycles"=9, "Mode Setting"="Hybrid", "Flow Rate (GPM)"=3.0, "Temperature (F)"=58.0, "Reset Timer"=FALSE, "Use Temp Decline Method"=FALSE, "Terminate Condition"=enum."C1-Terminate Draw @ Gallon Mark", "Condition Value #1"=15.0, "UE"=FALSE, "LE"=FALSE, "Comp"=FALSE, "Fan"=FALSE, "Test End Time (Sec)"=0.0, "Purge Until Cutout"=FALSE, "Start Conditions"=enum."Heat Source Cutout", "Condition Value #2"=0.0, "Remove Power"=FALSE, "Time"=0.0, "Check Special Cond."=enum."SC1-Do Nothing", "Condition#"=enum."N/A", "Draw Flags"=enum."N/A", "Data Processing Delay (FHD 15sec, UEF 5 Sec)"=15.0, "Test Complete"=FALSE}, {"Sequence #"=3.0, "Cycles"=2, "Mode Setting"="Heat Pump", "Flow Rate (GPM)"=3.0, "Temperature (F)"=58.0, "Reset Timer"=FALSE, "Use Temp Decline Method"=FALSE, "Terminate Condition"=enum."C1-Terminate Draw @ Gallon Mark", "Condition Value #1"=35.0, "UE"=FALSE, "LE"=FALSE, "Comp"=FALSE, "Fan"=FALSE, "Test End Time (Sec)"=0.0, "Purge Until Cutout"=FALSE, "Start Conditions"=enum."Heat Source Cutout", "Condition Value #2"=0.0, "Remove Power"=FALSE, "Time"=0.0, "Check Special Cond."=enum."SC1-Do Nothing", "Condition#"=enum."N/A", "Draw Flags"=enum."N/A", "Data Processing Delay (FHD 15sec, UEF 5 Sec)"=15.0, "Test Complete"=FALSE}, {"Sequence #"=4.0, "Cycles"=5, "Mode Setting"="Heat Pump", "Flow Rate (GPM)"=3.0, "Temperature (F)"=58.0, "Reset Timer"=FALSE, "Use Temp Decline Method"=FALSE, "Terminate Condition"=enum."C1-Terminate Draw @ Gallon Mark", "Condition Value #1"=15.0, "UE"=FALSE, "LE"=FALSE, "Comp"=FALSE, "Fan"=FALSE, "Test End Time (Sec)"=0.0, "Purge Until Cutout"=FALSE, "Start Conditions"=enum."Heat Source Cutout", "Condition Value #2"=0.0, "Remove Power"=FALSE, "Time"=0.0, "Check Special Cond."=enum."SC1-Do Nothing", "Condition#"=enum."N/A", "Draw Flags"=enum."N/A", "Data Processing Delay (FHD 15sec, UEF 5 Sec)"=15.0, "Test Complete"=FALSE}, {"Sequence #"=5.0, "Cycles"=2, "Mode Setting"="Standard", "Flow Rate (GPM)"=3.0, "Temperature (F)"=58.0, "Reset Timer"=FALSE, "Use Temp Decline Method"=FALSE, "Terminate Condition"=enum."C1-Terminate Draw @ Gallon Mark", "Condition Value #1"=35.0, "UE"=FALSE, "LE"=FALSE, "Comp"=FALSE, "Fan"=FALSE, "Test End Time (Sec)"=0.0, "Purge Until Cutout"=FALSE, "Start Conditions"=enum."Heat Source Cutout", "Condition Value #2"=0.0, "Remove Power"=FALSE, "Time"=0.0, "Check Special Cond."=enum."SC1-Do Nothing", "Condition#"=enum."N/A", "Draw Flags"=enum."N/A", "Data Processing Delay (FHD 15sec, UEF 5 Sec)"=15.0, "Test Complete"=FALSE}, {"Sequence #"=6.0, "Cycles"=5, "Mode Setting"="Standard", "Flow Rate (GPM)"=3.0, "Temperature (F)"=58.0, "Reset Timer"=FALSE, "Use Temp Decline Method"=FALSE, "Terminate Condition"=enum."C1-Terminate Draw @ Gallon Mark", "Condition Value #1"=15.0, "UE"=FALSE, "LE"=FALSE, "Comp"=FALSE, "Fan"=FALSE, "Test End Time (Sec)"=0.0, "Purge Until Cutout"=FALSE, "Start Conditions"=enum."Heat Source Cutout", "Condition Value #2"=0.0, "Remove Power"=FALSE, "Time"=0.0, "Check Special Cond."=enum."SC1-Do Nothing", "Condition#"=enum."N/A", "Draw Flags"=enum."N/A", "Data Processing Delay (FHD 15sec, UEF 5 Sec)"=15.0, "Test Complete"=FALSE}, {"Sequence #"=7.0, "Cycles"=2, "Mode Setting"="Hybrid", "Flow Rate (GPM)"=3.0, "Temperature (F)"=58.0, "Reset Timer"=FALSE, "Use Temp Decline Method"=FALSE, "Terminate Condition"=enum."C1-Terminate Draw @ Gallon Mark", "Condition Value #1"=35.0, "UE"=FALSE, "LE"=FALSE, "Comp"=FALSE, "Fan"=FALSE, "Test End Time (Sec)"=0.0, "Purge Until Cutout"=FALSE, "Start Conditions"=enum."Heat Source Cutout", "Condition Value #2"=0.0, "Remove Power"=FALSE, "Time"=0.0, "Check Special Cond."=enum."SC1-Do Nothing", "Condition#"=enum."N/A", "Draw Flags"=enum."N/A", "Data Processing Delay (FHD 15sec, UEF 5 Sec)"=15.0, "Test Complete"=FALSE}, {"Sequence #"=8.0, "Cycles"=5, "Mode Setting"="Hybrid", "Flow Rate (GPM)"=3.0, "Temperature (F)"=58.0, "Reset Timer"=FALSE, "Use Temp Decline Method"=FALSE, "Terminate Condition"=enum."C1-Terminate Draw @ Gallon Mark", "Condition Value #1"=15.0, "UE"=FALSE, "LE"=FALSE, "Comp"=FALSE, "Fan"=FALSE, "Test End Time (Sec)"=0.0, "Purge Until Cutout"=FALSE, "Start Conditions"=enum."Heat Source Cutout", "Condition Value #2"=0.0, "Remove Power"=FALSE, "Time"=0.0, "Check Special Cond."=enum."SC1-Do Nothing", "Condition#"=enum."N/A", "Draw Flags"=enum."N/A", "Data Processing Delay (FHD 15sec, UEF 5 Sec)"=15.0, "Test Complete"=FALSE}, {"Sequence #"=9.0, "Cycles"=3, "Mode Setting"="Hybrid", "Flow Rate (GPM)"=3.0, "Temperature (F)"=58.0, "Reset Timer"=FALSE, "Use Temp Decline Method"=FALSE, "Terminate Condition"=enum."C1-Terminate Draw @ Gallon Mark", "Condition Value #1"=35.0, "UE"=FALSE, "LE"=FALSE, "Comp"=FALSE, "Fan"=FALSE, "Test End Time (Sec)"=0.0, "Purge Until Cutout"=FALSE, "Start Conditions"=enum."Heat Source Cutout", "Condition Value #2"=0.0, "Remove Power"=FALSE, "Time"=0.0, "Check Special Cond."=enum."SC1-Do Nothing", "Condition#"=enum."N/A", "Draw Flags"=enum."N/A", "Data Processing Delay (FHD 15sec, UEF 5 Sec)"=15.0, "Test Complete"=FALSE}, {"Sequence #"=10.0, "Cycles"=16, "Mode Setting"="Hybrid", "Flow Rate (GPM)"=3.0, "Temperature (F)"=58.0, "Reset Timer"=FALSE, "Use Temp Decline Method"=FALSE, "Terminate Condition"=enum."C1-Terminate Draw @ Gallon Mark", "Condition Value #1"=15.0, "UE"=FALSE, "LE"=FALSE, "Comp"=FALSE, "Fan"=FALSE, "Test End Time (Sec)"=0.0, "Purge Until Cutout"=FALSE, "Start Conditions"=enum."Heat Source Cutout", "Condition Value #2"=0.0, "Remove Power"=FALSE, "Time"=0.0, "Check Special Cond."=enum."SC1-Do Nothing", "Condition#"=enum."N/A", "Draw Flags"=enum."N/A", "Data Processing Delay (FHD 15sec, UEF 5 Sec)"=15.0, "Test Complete"=FALSE}, {"Sequence #"=11.0, "Cycles"=3, "Mode Setting"="Heat Pump", "Flow Rate (GPM)"=3.0, "Temperature (F)"=58.0, "Reset Timer"=FALSE, "Use Temp Decline Method"=FALSE, "Terminate Condition"=enum."C1-Terminate Draw @ Gallon Mark", "Condition Value #1"=35.0, "UE"=FALSE, "LE"=FALSE, "Comp"=FALSE, "Fan"=FALSE, "Test End Time (Sec)"=0.0, "Purge Until Cutout"=FALSE, "Start Conditions"=enum."Heat Source Cutout", "Condition Value #2"=0.0, "Remove Power"=FALSE, "Time"=0.0, "Check Special Cond."=enum."SC1-Do Nothing", "Condition#"=enum."N/A", "Draw Flags"=enum."N/A", "Data Processing Delay (FHD 15sec, UEF 5 Sec)"=15.0, "Test Complete"=FALSE}, {"Sequence #"=12.0, "Cycles"=16, "Mode Setting"="Heat Pump", "Flow Rate (GPM)"=3.0, "Temperature (F)"=58.0, "Reset Timer"=FALSE, "Use Temp Decline Method"=FALSE, "Terminate Condition"=enum."C1-Terminate Draw @ Gallon Mark", "Condition Value #1"=15.0, "UE"=FALSE, "LE"=FALSE, "Comp"=FALSE, "Fan"=FALSE, "Test End Time (Sec)"=0.0, "Purge Until Cutout"=FALSE, "Start Conditions"=enum."Heat Source Cutout", "Condition Value #2"=0.0, "Remove Power"=FALSE, "Time"=0.0, "Check Special Cond."=enum."SC1-Do Nothing", "Condition#"=enum."N/A", "Draw Flags"=enum."N/A", "Data Processing Delay (FHD 15sec, UEF 5 Sec)"=15.0, "Test Complete"=FALSE}, {"Sequence #"=13.0, "Cycles"=3, "Mode Setting"="Standard", "Flow Rate (GPM)"=3.0, "Temperature (F)"=58.0, "Reset Timer"=FALSE, "Use Temp Decline Method"=FALSE, "Terminate Condition"=enum."C1-Terminate Draw @ Gallon Mark", "Condition Value #1"=35.0, "UE"=FALSE, "LE"=FALSE, "Comp"=FALSE, "Fan"=FALSE, "Test End Time (Sec)"=0.0, "Purge Until Cutout"=FALSE, "Start Conditions"=enum."Heat Source Cutout", "Condition Value #2"=0.0, "Remove Power"=FALSE, "Time"=0.0, "Check Special Cond."=enum."SC1-Do Nothing", "Condition#"=enum."N/A", "Draw Flags"=enum."N/A", "Data Processing Delay (FHD 15sec, UEF 5 Sec)"=15.0, "Test Complete"=FALSE}, {"Sequence #"=14.0, "Cycles"=16, "Mode Setting"="Standard", "Flow Rate (GPM)"=3.0, "Temperature (F)"=58.0, "Reset Timer"=FALSE, "Use Temp Decline Method"=FALSE, "Terminate Condition"=enum."C1-Terminate Draw @ Gallon Mark", "Condition Value #1"=15.0, "UE"=FALSE, "LE"=FALSE, "Comp"=FALSE, "Fan"=FALSE, "Test End Time (Sec)"=0.0, "Purge Until Cutout"=FALSE, "Start Conditions"=enum."Heat Source Cutout", "Condition Value #2"=0.0, "Remove Power"=FALSE, "Time"=0.0, "Check Special Cond."=enum."SC1-Do Nothing", "Condition#"=enum."N/A", "Draw Flags"=enum."N/A", "Data Processing Delay (FHD 15sec, UEF 5 Sec)"=15.0, "Test Complete"=FALSE}, {"Sequence #"=15.0, "Cycles"=141, "Mode Setting"="Hybrid", "Flow Rate (GPM)"=3.0, "Temperature (F)"=58.0, "Reset Timer"=FALSE, "Use Temp Decline Method"=FALSE, "Terminate Condition"=enum."C1-Terminate Draw @ Gallon Mark", "Condition Value #1"=35.0, "UE"=FALSE, "LE"=FALSE, "Comp"=FALSE, "Fan"=FALSE, "Test End Time (Sec)"=0.0, "Purge Until Cutout"=FALSE, "Start Conditions"=enum."Heat Source Cutout", "Condition Value #2"=0.0, "Remove Power"=FALSE, "Time"=0.0, "Check Special Cond."=enum."SC1-Do Nothing", "Condition#"=enum."N/A", "Draw Flags"=enum."N/A", "Data Processing Delay (FHD 15sec, UEF 5 Sec)"=15.0, "Test Complete"=FALSE}, {"Sequence #"=16.0, "Cycles"=767, "Mode Setting"="Hybrid", "Flow Rate (GPM)"=3.0, "Temperature (F)"=58.0, "Reset Timer"=FALSE, "Use Temp Decline Method"=FALSE, "Terminate Condition"=enum."C1-Terminate Draw @ Gallon Mark", "Condition Value #1"=15.0, "UE"=FALSE, "LE"=FALSE, "Comp"=FALSE, "Fan"=FALSE, "Test End Time (Sec)"=0.0, "Purge Until Cutout"=FALSE, "Start Conditions"=enum."Heat Source Cutout", "Condition Value #2"=0.0, "Remove Power"=FALSE, "Time"=0.0, "Check Special Cond."=enum."SC1-Do Nothing", "Condition#"=enum."N/A", "Draw Flags"=enum."N/A", "Data Processing Delay (FHD 15sec, UEF 5 Sec)"=15.0, "Test Complete"=FALSE}, {"Sequence #"=17.0, "Cycles"=3, "Mode Setting"="Hybrid", "Flow Rate (GPM)"=3.0, "Temperature (F)"=58.0, "Reset Timer"=FALSE, "Use Temp Decline Method"=FALSE, "Terminate Condition"=enum."C1-Terminate Draw @ Gallon Mark", "Condition Value #1"=35.0, "UE"=FALSE, "LE"=FALSE, "Comp"=FALSE, "Fan"=FALSE, "Test End Time (Sec)"=0.0, "Purge Until Cutout"=FALSE, "Start Conditions"=enum."Heat Source Cutout", "Condition Value #2"=0.0, "Remove Power"=FALSE, "Time"=0.0, "Check Special Cond."=enum."SC1-Do Nothing", "Condition#"=enum."N/A", "Draw Flags"=enum."N/A", "Data Processing Delay (FHD 15sec, UEF 5 Sec)"=15.0, "Test Complete"=FALSE}, {"Sequence #"=18.0, "Cycles"=16, "Mode Setting"="Hybrid", "Flow Rate (GPM)"=3.0, "Temperature (F)"=58.0, "Reset Timer"=FALSE, "Use Temp Decline Method"=FALSE, "Terminate Condition"=enum."C1-Terminate Draw @ Gallon Mark", "Condition Value #1"=15.0, "UE"=FALSE, "LE"=FALSE, "Comp"=FALSE, "Fan"=FALSE, "Test End Time (Sec)"=0.0, "Purge Until Cutout"=FALSE, "Start Conditions"=enum."Heat Source Cutout", "Condition Value #2"=0.0, "Remove Power"=FALSE, "Time"=0.0, "Check Special Cond."=enum."SC1-Do Nothing", "Condition#"=enum."N/A", "Draw Flags"=enum."N/A", "Data Processing Delay (FHD 15sec, UEF 5 Sec)"=15.0, "Test Complete"=FALSE}, {"Sequence #"=19.0, "Cycles"=3, "Mode Setting"="Heat Pump", "Flow Rate (GPM)"=3.0, "Temperature (F)"=58.0, "Reset Timer"=FALSE, "Use Temp Decline Method"=FALSE, "Terminate Condition"=enum."C1-Terminate Draw @ Gallon Mark", "Condition Value #1"=35.0, "UE"=FALSE, "LE"=FALSE, "Comp"=FALSE, "Fan"=FALSE, "Test End Time (Sec)"=0.0, "Purge Until Cutout"=FALSE, "Start Conditions"=enum."Heat Source Cutout", "Condition Value #2"=0.0, "Remove Power"=FALSE, "Time"=0.0, "Check Special Cond."=enum."SC1-Do Nothing", "Condition#"=enum."N/A", "Draw Flags"=enum."N/A", "Data Processing Delay (FHD 15sec, UEF 5 Sec)"=15.0, "Test Complete"=FALSE}, {"Sequence #"=20.0, "Cycles"=16, "Mode Setting"="Heat Pump", "Flow Rate (GPM)"=3.0, "Temperature (F)"=58.0, "Reset Timer"=FALSE, "Use Temp Decline Method"=FALSE, "Terminate Condition"=enum."C1-Terminate Draw @ Gallon Mark", "Condition Value #1"=15.0, "UE"=FALSE, "LE"=FALSE, "Comp"=FALSE, "Fan"=FALSE, "Test End Time (Sec)"=0.0, "Purge Until Cutout"=FALSE, "Start Conditions"=enum."Heat Source Cutout", "Condition Value #2"=0.0, "Remove Power"=FALSE, "Time"=0.0, "Check Special Cond."=enum."SC1-Do Nothing", "Condition#"=enum."N/A", "Draw Flags"=enum."N/A", "Data Processing Delay (FHD 15sec, UEF 5 Sec)"=15.0, "Test Complete"=FALSE}, {"Sequence #"=21.0, "Cycles"=3, "Mode Setting"="Standard", "Flow Rate (GPM)"=3.0, "Temperature (F)"=58.0, "Reset Timer"=FALSE, "Use Temp Decline Method"=FALSE, "Terminate Condition"=enum."C1-Terminate Draw @ Gallon Mark", "Condition Value #1"=35.0, "UE"=FALSE, "LE"=FALSE, "Comp"=FALSE, "Fan"=FALSE, "Test End Time (Sec)"=0.0, "Purge Until Cutout"=FALSE, "Start Conditions"=enum."Heat Source Cutout", "Condition Value #2"=0.0, "Remove Power"=FALSE, "Time"=0.0, "Check Special Cond."=enum."SC1-Do Nothing", "Condition#"=enum."N/A", "Draw Flags"=enum."N/A", "Data Processing Delay (FHD 15sec, UEF 5 Sec)"=15.0, "Test Complete"=FALSE}, {"Sequence #"=22.0, "Cycles"=16, "Mode Setting"="Standard", "Flow Rate (GPM)"=3.0, "Temperature (F)"=58.0, "Reset Timer"=FALSE, "Use Temp Decline Method"=FALSE, "Terminate Condition"=enum."C1-Terminate Draw @ Gallon Mark", "Condition Value #1"=15.0, "UE"=FALSE, "LE"=FALSE, "Comp"=FALSE, "Fan"=FALSE, "Test End Time (Sec)"=0.0, "Purge Until Cutout"=FALSE, "Start Conditions"=enum."Heat Source Cutout", "Condition Value #2"=0.0, "Remove Power"=FALSE, "Time"=0.0, "Check Special Cond."=enum."SC1-Do Nothing", "Condition#"=enum."N/A", "Draw Flags"=enum."N/A", "Data Processing Delay (FHD 15sec, UEF 5 Sec)"=15.0, "Test Complete"=FALSE}, {"Sequence #"=23.0, "Cycles"=147, "Mode Setting"="Hybrid", "Flow Rate (GPM)"=3.0, "Temperature (F)"=58.0, "Reset Timer"=FALSE, "Use Temp Decline Method"=FALSE, "Terminate Condition"=enum."C1-Terminate Draw @ Gallon Mark", "Condition Value #1"=35.0, "UE"=FALSE, "LE"=FALSE, "Comp"=FALSE, "Fan"=FALSE, "Test End Time (Sec)"=0.0, "Purge Until Cutout"=FALSE, "Start Conditions"=enum."Heat Source Cutout", "Condition Value #2"=0.0, "Remove Power"=FALSE, "Time"=0.0, "Check Special Cond."=enum."SC1-Do Nothing", "Condition#"=enum."N/A", "Draw Flags"=enum."N/A", "Data Processing Delay (FHD 15sec, UEF 5 Sec)"=15.0, "Test Complete"=FALSE}, {"Sequence #"=24.0, "Cycles"=817, "Mode Setting"="Hybrid", "Flow Rate (GPM)"=3.0, "Temperature (F)"=58.0, "Reset Timer"=FALSE, "Use Temp Decline Method"=FALSE, "Terminate Condition"=enum."C1-Terminate Draw @ Gallon Mark", "Condition Value #1"=15.0, "UE"=FALSE, "LE"=FALSE, "Comp"=FALSE, "Fan"=FALSE, "Test End Time (Sec)"=0.0, "Purge Until Cutout"=FALSE, "Start Conditions"=enum."Heat Source Cutout", "Condition Value #2"=0.0, "Remove Power"=FALSE, "Time"=0.0, "Check Special Cond."=enum."SC1-Do Nothing", "Condition#"=enum."N/A", "Draw Flags"=enum."N/A", "Data Processing Delay (FHD 15sec, UEF 5 Sec)"=15.0, "Test Complete"=FALSE}, {"Sequence #"=25.0, "Cycles"=3, "Mode Setting"="Heat Pump", "Flow Rate (GPM)"=3.0, "Temperature (F)"=58.0, "Reset Timer"=FALSE, "Use Temp Decline Method"=FALSE, "Terminate Condition"=enum."C1-Terminate Draw @ Gallon Mark", "Condition Value #1"=35.0, "UE"=FALSE, "LE"=FALSE, "Comp"=FALSE, "Fan"=FALSE, "Test End Time (Sec)"=0.0, "Purge Until Cutout"=FALSE, "Start Conditions"=enum."Heat Source Cutout", "Condition Value #2"=0.0, "Remove Power"=FALSE, "Time"=0.0, "Check Special Cond."=enum."SC1-Do Nothing", "Condition#"=enum."N/A", "Draw Flags"=enum."N/A", "Data Processing Delay (FHD 15sec, UEF 5 Sec)"=15.0, "Test Complete"=FALSE}, {"Sequence #"=26.0, "Cycles"=16, "Mode Setting"="Heat Pump", "Flow Rate (GPM)"=3.0, "Temperature (F)"=58.0, "Reset Timer"=FALSE, "Use Temp Decline Method"=FALSE, "Terminate Condition"=enum."C1-Terminate Draw @ Gallon Mark", "Condition Value #1"=15.0, "UE"=FALSE, "LE"=FALSE, "Comp"=FALSE, "Fan"=FALSE, "Test End Time (Sec)"=0.0, "Purge Until Cutout"=FALSE, "Start Conditions"=enum."Heat Source Cutout", "Condition Value #2"=0.0, "Remove Power"=FALSE, "Time"=0.0, "Check Special Cond."=enum."SC1-Do Nothing", "Condition#"=enum."N/A", "Draw Flags"=enum."N/A", "Data Processing Delay (FHD 15sec, UEF 5 Sec)"=15.0, "Test Complete"=FALSE}, {"Sequence #"=27.0, "Cycles"=3, "Mode Setting"="Standard", "Flow Rate (GPM)"=3.0, "Temperature (F)"=58.0, "Reset Timer"=FALSE, "Use Temp Decline Method"=FALSE, "Terminate Condition"=enum."C1-Terminate Draw @ Gallon Mark", "Condition Value #1"=35.0, "UE"=FALSE, "LE"=FALSE, "Comp"=FALSE, "Fan"=FALSE, "Test End Time (Sec)"=0.0, "Purge Until Cutout"=FALSE, "Start Conditions"=enum."Heat Source Cutout", "Condition Value #2"=0.0, "Remove Power"=FALSE, "Time"=0.0, "Check Special Cond."=enum."SC1-Do Nothing", "Condition#"=enum."N/A", "Draw Flags"=enum."N/A", "Data Processing Delay (FHD 15sec, UEF 5 Sec)"=15.0, "Test Complete"=FALSE}, {"Sequence #"=28.0, "Cycles"=16, "Mode Setting"="Standard", "Flow Rate (GPM)"=3.0, "Temperature (F)"=58.0, "Reset Timer"=FALSE, "Use Temp Decline Method"=FALSE, "Terminate Condition"=enum."C1-Terminate Draw @ Gallon Mark", "Condition Value #1"=15.0, "UE"=FALSE, "LE"=FALSE, "Comp"=FALSE, "Fan"=FALSE, "Test End Time (Sec)"=0.0, "Purge Until Cutout"=FALSE, "Start Conditions"=enum."Heat Source Cutout", "Condition Value #2"=0.0, "Remove Power"=FALSE, "Time"=0.0, "Check Special Cond."=enum."SC1-Do Nothing", "Condition#"=enum."N/A", "Draw Flags"=enum."N/A", "Data Processing Delay (FHD 15sec, UEF 5 Sec)"=15.0, "Test Complete"=FALSE}, {"Sequence #"=29.0, "Cycles"=138, "Mode Setting"="Hybrid", "Flow Rate (GPM)"=3.0, "Temperature (F)"=58.0, "Reset Timer"=FALSE, "Use Temp Decline Method"=FALSE, "Terminate Condition"=enum."C1-Terminate Draw @ Gallon Mark", "Condition Value #1"=35.0, "UE"=FALSE, "LE"=FALSE, "Comp"=FALSE, "Fan"=FALSE, "Test End Time (Sec)"=0.0, "Purge Until Cutout"=FALSE, "Start Conditions"=enum."Heat Source Cutout", "Condition Value #2"=0.0, "Remove Power"=FALSE, "Time"=0.0, "Check Special Cond."=enum."SC1-Do Nothing", "Condition#"=enum."N/A", "Draw Flags"=enum."N/A", "Data Processing Delay (FHD 15sec, UEF 5 Sec)"=15.0, "Test Complete"=FALSE}, {"Sequence #"=30.0, "Cycles"=302, "Mode Setting"="Hybrid", "Flow Rate (GPM)"=3.0, "Temperature (F)"=58.0, "Reset Timer"=FALSE, "Use Temp Decline Method"=FALSE, "Terminate Condition"=enum."C1-Terminate Draw @ Gallon Mark", "Condition Value #1"=15.0, "UE"=FALSE, "LE"=FALSE, "Comp"=FALSE, "Fan"=FALSE, "Test End Time (Sec)"=0.0, "Purge Until Cutout"=FALSE, "Start Conditions"=enum."Heat Source Cutout", "Condition Value #2"=0.0, "Remove Power"=FALSE, "Time"=0.0, "Check Special Cond."=enum."SC1-Do Nothing", "Condition#"=enum."N/A", "Draw Flags"=enum."N/A", "Data Processing Delay (FHD 15sec, UEF 5 Sec)"=15.0, "Test Complete"=FALSE}, {"Sequence #"=31.0, "Cycles"=1, "Mode Setting"="", "Flow Rate (GPM)"=3.0, "Temperature (F)"=58.0, "Reset Timer"=FALSE, "Use Temp Decline Method"=FALSE, "Terminate Condition"=enum."C9-Do Nothing", "Condition Value #1"=0.0, "UE"=FALSE, "LE"=FALSE, "Comp"=FALSE, "Fan"=FALSE, "Test End Time (Sec)"=0.0, "Purge Until Cutout"=FALSE, "Start Conditions"=enum."Heat Source Cutout", "Condition Value #2"=0.0, "Remove Power"=FALSE, "Time"=0.0, "Check Special Cond."=enum."SC1-Do Nothing", "Condition#"=enum."N/A", "Draw Flags"=enum."N/A", "Data Processing Delay (FHD 15sec, UEF 5 Sec)"=15.0, "Test Complete"=TRUE}] {"Time" format="%<%H:%M:%S>t"}
  in  "1 Year Standard":T21[](array[typedef])=[{"Sequence #"=1.0, "Cycles"=4, "Mode Setting"="Hybrid", "Flow Rate (GPM)"=3.0, "Temperature (F)"=58.0, "Reset Timer"=FALSE, "Use Temp Decline Method"=FALSE, "Terminate Condition"=enum."C1-Terminate Draw @ Gallon Mark", "Condition Value #1"=35.0, "UE"=FALSE, "LE"=FALSE, "Comp"=FALSE, "Fan"=FALSE, "Test End Time (Sec)"=0.0, "Purge Until Cutout"=FALSE, "Start Conditions"=enum."Heat Source Cutout", "Condition Value #2"=0.0, "Remove Power"=FALSE, "Time"=0.0, "Check Special Cond."=enum."SC1-Do Nothing", "Condition#"=enum."N/A", "Draw Flags"=enum."N/A", "Data Processing Delay (FHD 15sec, UEF 5 Sec)"=15.0, "Test Complete"=FALSE}, {"Sequence #"=2.0, "Cycles"=9, "Mode Setting"="Hybrid", "Flow Rate (GPM)"=3.0, "Temperature (F)"=58.0, "Reset Timer"=FALSE, "Use Temp Decline Method"=FALSE, "Terminate Condition"=enum."C1-Terminate Draw @ Gallon Mark", "Condition Value #1"=15.0, "UE"=FALSE, "LE"=FALSE, "Comp"=FALSE, "Fan"=FALSE, "Test End Time (Sec)"=0.0, "Purge Until Cutout"=FALSE, "Start Conditions"=enum."Heat Source Cutout", "Condition Value #2"=0.0, "Remove Power"=FALSE, "Time"=0.0, "Check Special Cond."=enum."SC1-Do Nothing", "Condition#"=enum."N/A", "Draw Flags"=enum."N/A", "Data Processing Delay (FHD 15sec, UEF 5 Sec)"=15.0, "Test Complete"=FALSE}, {"Sequence #"=3.0, "Cycles"=2, "Mode Setting"="Heat Pump", "Flow Rate (GPM)"=3.0, "Temperature (F)"=58.0, "Reset Timer"=FALSE, "Use Temp Decline Method"=FALSE, "Terminate Condition"=enum."C1-Terminate Draw @ Gallon Mark", "Condition Value #1"=35.0, "UE"=FALSE, "LE"=FALSE, "Comp"=FALSE, "Fan"=FALSE, "Test End Time (Sec)"=0.0, "Purge Until Cutout"=FALSE, "Start Conditions"=enum."Heat Source Cutout", "Condition Value #2"=0.0, "Remove Power"=FALSE, "Time"=0.0, "Check Special Cond."=enum."SC1-Do Nothing", "Condition#"=enum."N/A", "Draw Flags"=enum."N/A", "Data Processing Delay (FHD 15sec, UEF 5 Sec)"=15.0, "Test Complete"=FALSE}, {"Sequence #"=4.0, "Cycles"=5, "Mode Setting"="Heat Pump", "Flow Rate (GPM)"=3.0, "Temperature (F)"=58.0, "Reset Timer"=FALSE, "Use Temp Decline Method"=FALSE, "Terminate Condition"=enum."C1-Terminate Draw @ Gallon Mark", "Condition Value #1"=15.0, "UE"=FALSE, "LE"=FALSE, "Comp"=FALSE, "Fan"=FALSE, "Test End Time (Sec)"=0.0, "Purge Until Cutout"=FALSE, "Start Conditions"=enum."Heat Source Cutout", "Condition Value #2"=0.0, "Remove Power"=FALSE, "Time"=0.0, "Check Special Cond."=enum."SC1-Do Nothing", "Condition#"=enum."N/A", "Draw Flags"=enum."N/A", "Data Processing Delay (FHD 15sec, UEF 5 Sec)"=15.0, "Test Complete"=FALSE}, {"Sequence #"=5.0, "Cycles"=2, "Mode Setting"="Standard", "Flow Rate (GPM)"=3.0, "Temperature (F)"=58.0, "Reset Timer"=FALSE, "Use Temp Decline Method"=FALSE, "Terminate Condition"=enum."C1-Terminate Draw @ Gallon Mark", "Condition Value #1"=35.0, "UE"=FALSE, "LE"=FALSE, "Comp"=FALSE, "Fan"=FALSE, "Test End Time (Sec)"=0.0, "Purge Until Cutout"=FALSE, "Start Conditions"=enum."Heat Source Cutout", "Condition Value #2"=0.0, "Remove Power"=FALSE, "Time"=0.0, "Check Special Cond."=enum."SC1-Do Nothing", "Condition#"=enum."N/A", "Draw Flags"=enum."N/A", "Data Processing Delay (FHD 15sec, UEF 5 Sec)"=15.0, "Test Complete"=FALSE}, {"Sequence #"=6.0, "Cycles"=5, "Mode Setting"="Standard", "Flow Rate (GPM)"=3.0, "Temperature (F)"=58.0, "Reset Timer"=FALSE, "Use Temp Decline Method"=FALSE, "Terminate Condition"=enum."C1-Terminate Draw @ Gallon Mark", "Condition Value #1"=15.0, "UE"=FALSE, "LE"=FALSE, "Comp"=FALSE, "Fan"=FALSE, "Test End Time (Sec)"=0.0, "Purge Until Cutout"=FALSE, "Start Conditions"=enum."Heat Source Cutout", "Condition Value #2"=0.0, "Remove Power"=FALSE, "Time"=0.0, "Check Special Cond."=enum."SC1-Do Nothing", "Condition#"=enum."N/A", "Draw Flags"=enum."N/A", "Data Processing Delay (FHD 15sec, UEF 5 Sec)"=15.0, "Test Complete"=FALSE}, {"Sequence #"=7.0, "Cycles"=2, "Mode Setting"="Hybrid", "Flow Rate (GPM)"=3.0, "Temperature (F)"=58.0, "Reset Timer"=FALSE, "Use Temp Decline Method"=FALSE, "Terminate Condition"=enum."C1-Terminate Draw @ Gallon Mark", "Condition Value #1"=35.0, "UE"=FALSE, "LE"=FALSE, "Comp"=FALSE, "Fan"=FALSE, "Test End Time (Sec)"=0.0, "Purge Until Cutout"=FALSE, "Start Conditions"=enum."Heat Source Cutout", "Condition Value #2"=0.0, "Remove Power"=FALSE, "Time"=0.0, "Check Special Cond."=enum."SC1-Do Nothing", "Condition#"=enum."N/A", "Draw Flags"=enum."N/A", "Data Processing Delay (FHD 15sec, UEF 5 Sec)"=15.0, "Test Complete"=FALSE}, {"Sequence #"=8.0, "Cycles"=5, "Mode Setting"="Hybrid", "Flow Rate (GPM)"=3.0, "Temperature (F)"=58.0, "Reset Timer"=FALSE, "Use Temp Decline Method"=FALSE, "Terminate Condition"=enum."C1-Terminate Draw @ Gallon Mark", "Condition Value #1"=15.0, "UE"=FALSE, "LE"=FALSE, "Comp"=FALSE, "Fan"=FALSE, "Test End Time (Sec)"=0.0, "Purge Until Cutout"=FALSE, "Start Conditions"=enum."Heat Source Cutout", "Condition Value #2"=0.0, "Remove Power"=FALSE, "Time"=0.0, "Check Special Cond."=enum."SC1-Do Nothing", "Condition#"=enum."N/A", "Draw Flags"=enum."N/A", "Data Processing Delay (FHD 15sec, UEF 5 Sec)"=15.0, "Test Complete"=FALSE}, {"Sequence #"=9.0, "Cycles"=3, "Mode Setting"="Hybrid", "Flow Rate (GPM)"=3.0, "Temperature (F)"=58.0, "Reset Timer"=FALSE, "Use Temp Decline Method"=FALSE, "Terminate Condition"=enum."C1-Terminate Draw @ Gallon Mark", "Condition Value #1"=35.0, "UE"=FALSE, "LE"=FALSE, "Comp"=FALSE, "Fan"=FALSE, "Test End Time (Sec)"=0.0, "Purge Until Cutout"=FALSE, "Start Conditions"=enum."Heat Source Cutout", "Condition Value #2"=0.0, "Remove Power"=FALSE, "Time"=0.0, "Check Special Cond."=enum."SC1-Do Nothing", "Condition#"=enum."N/A", "Draw Flags"=enum."N/A", "Data Processing Delay (FHD 15sec, UEF 5 Sec)"=15.0, "Test Complete"=FALSE}, {"Sequence #"=10.0, "Cycles"=16, "Mode Setting"="Hybrid", "Flow Rate (GPM)"=3.0, "Temperature (F)"=58.0, "Reset Timer"=FALSE, "Use Temp Decline Method"=FALSE, "Terminate Condition"=enum."C1-Terminate Draw @ Gallon Mark", "Condition Value #1"=15.0, "UE"=FALSE, "LE"=FALSE, "Comp"=FALSE, "Fan"=FALSE, "Test End Time (Sec)"=0.0, "Purge Until Cutout"=FALSE, "Start Conditions"=enum."Heat Source Cutout", "Condition Value #2"=0.0, "Remove Power"=FALSE, "Time"=0.0, "Check Special Cond."=enum."SC1-Do Nothing", "Condition#"=enum."N/A", "Draw Flags"=enum."N/A", "Data Processing Delay (FHD 15sec, UEF 5 Sec)"=15.0, "Test Complete"=FALSE}, {"Sequence #"=11.0, "Cycles"=3, "Mode Setting"="Heat Pump", "Flow Rate (GPM)"=3.0, "Temperature (F)"=58.0, "Reset Timer"=FALSE, "Use Temp Decline Method"=FALSE, "Terminate Condition"=enum."C1-Terminate Draw @ Gallon Mark", "Condition Value #1"=35.0, "UE"=FALSE, "LE"=FALSE, "Comp"=FALSE, "Fan"=FALSE, "Test End Time (Sec)"=0.0, "Purge Until Cutout"=FALSE, "Start Conditions"=enum."Heat Source Cutout", "Condition Value #2"=0.0, "Remove Power"=FALSE, "Time"=0.0, "Check Special Cond."=enum."SC1-Do Nothing", "Condition#"=enum."N/A", "Draw Flags"=enum."N/A", "Data Processing Delay (FHD 15sec, UEF 5 Sec)"=15.0, "Test Complete"=FALSE}, {"Sequence #"=12.0, "Cycles"=16, "Mode Setting"="Heat Pump", "Flow Rate (GPM)"=3.0, "Temperature (F)"=58.0, "Reset Timer"=FALSE, "Use Temp Decline Method"=FALSE, "Terminate Condition"=enum."C1-Terminate Draw @ Gallon Mark", "Condition Value #1"=15.0, "UE"=FALSE, "LE"=FALSE, "Comp"=FALSE, "Fan"=FALSE, "Test End Time (Sec)"=0.0, "Purge Until Cutout"=FALSE, "Start Conditions"=enum."Heat Source Cutout", "Condition Value #2"=0.0, "Remove Power"=FALSE, "Time"=0.0, "Check Special Cond."=enum."SC1-Do Nothing", "Condition#"=enum."N/A", "Draw Flags"=enum."N/A", "Data Processing Delay (FHD 15sec, UEF 5 Sec)"=15.0, "Test Complete"=FALSE}, {"Sequence #"=13.0, "Cycles"=3, "Mode Setting"="Standard", "Flow Rate (GPM)"=3.0, "Temperature (F)"=58.0, "Reset Timer"=FALSE, "Use Temp Decline Method"=FALSE, "Terminate Condition"=enum."C1-Terminate Draw @ Gallon Mark", "Condition Value #1"=35.0, "UE"=FALSE, "LE"=FALSE, "Comp"=FALSE, "Fan"=FALSE, "Test End Time (Sec)"=0.0, "Purge Until Cutout"=FALSE, "Start Conditions"=enum."Heat Source Cutout", "Condition Value #2"=0.0, "Remove Power"=FALSE, "Time"=0.0, "Check Special Cond."=enum."SC1-Do Nothing", "Condition#"=enum."N/A", "Draw Flags"=enum."N/A", "Data Processing Delay (FHD 15sec, UEF 5 Sec)"=15.0, "Test Complete"=FALSE}, {"Sequence #"=14.0, "Cycles"=16, "Mode Setting"="Standard", "Flow Rate (GPM)"=3.0, "Temperature (F)"=58.0, "Reset Timer"=FALSE, "Use Temp Decline Method"=FALSE, "Terminate Condition"=enum."C1-Terminate Draw @ Gallon Mark", "Condition Value #1"=15.0, "UE"=FALSE, "LE"=FALSE, "Comp"=FALSE, "Fan"=FALSE, "Test End Time (Sec)"=0.0, "Purge Until Cutout"=FALSE, "Start Conditions"=enum."Heat Source Cutout", "Condition Value #2"=0.0, "Remove Power"=FALSE, "Time"=0.0, "Check Special Cond."=enum."SC1-Do Nothing", "Condition#"=enum."N/A", "Draw Flags"=enum."N/A", "Data Processing Delay (FHD 15sec, UEF 5 Sec)"=15.0, "Test Complete"=FALSE}, {"Sequence #"=15.0, "Cycles"=141, "Mode Setting"="Hybrid", "Flow Rate (GPM)"=3.0, "Temperature (F)"=58.0, "Reset Timer"=FALSE, "Use Temp Decline Method"=FALSE, "Terminate Condition"=enum."C1-Terminate Draw @ Gallon Mark", "Condition Value #1"=35.0, "UE"=FALSE, "LE"=FALSE, "Comp"=FALSE, "Fan"=FALSE, "Test End Time (Sec)"=0.0, "Purge Until Cutout"=FALSE, "Start Conditions"=enum."Heat Source Cutout", "Condition Value #2"=0.0, "Remove Power"=FALSE, "Time"=0.0, "Check Special Cond."=enum."SC1-Do Nothing", "Condition#"=enum."N/A", "Draw Flags"=enum."N/A", "Data Processing Delay (FHD 15sec, UEF 5 Sec)"=15.0, "Test Complete"=FALSE}, {"Sequence #"=16.0, "Cycles"=767, "Mode Setting"="Hybrid", "Flow Rate (GPM)"=3.0, "Temperature (F)"=58.0, "Reset Timer"=FALSE, "Use Temp Decline Method"=FALSE, "Terminate Condition"=enum."C1-Terminate Draw @ Gallon Mark", "Condition Value #1"=15.0, "UE"=FALSE, "LE"=FALSE, "Comp"=FALSE, "Fan"=FALSE, "Test End Time (Sec)"=0.0, "Purge Until Cutout"=FALSE, "Start Conditions"=enum."Heat Source Cutout", "Condition Value #2"=0.0, "Remove Power"=FALSE, "Time"=0.0, "Check Special Cond."=enum."SC1-Do Nothing", "Condition#"=enum."N/A", "Draw Flags"=enum."N/A", "Data Processing Delay (FHD 15sec, UEF 5 Sec)"=15.0, "Test Complete"=FALSE}, {"Sequence #"=17.0, "Cycles"=1, "Mode Setting"="", "Flow Rate (GPM)"=3.0, "Temperature (F)"=58.0, "Reset Timer"=FALSE, "Use Temp Decline Method"=FALSE, "Terminate Condition"=enum."C9-Do Nothing", "Condition Value #1"=0.0, "UE"=FALSE, "LE"=FALSE, "Comp"=FALSE, "Fan"=FALSE, "Test End Time (Sec)"=0.0, "Purge Until Cutout"=FALSE, "Start Conditions"=enum."Heat Source Cutout", "Condition Value #2"=0.0, "Remove Power"=FALSE, "Time"=0.0, "Check Special Cond."=enum."SC1-Do Nothing", "Condition#"=enum."N/A", "Draw Flags"=enum."N/A", "Data Processing Delay (FHD 15sec, UEF 5 Sec)"=15.0, "Test Complete"=TRUE}] {"Time" format="%<%H:%M:%S>t"}
  # "(Pre 2015) Standard Test 140°F Setpoint, 25°F Temperature Decrease (Unit setpoint is REQUIRED for test)"
  # "(Post 2015) Standard Test 125°F Setpoint, 15°F Temperature Decrease (Unit setpoint is REQUIRED for test)"
  # "The default:\nSubtract 180 seconds for Purge\nSubtract 12 second valve switch\nSubtract 30 seconds for tank pressurization"
  # "The default:\nSubtract 180 seconds for Purge\nSubtract 12 second valve switch\nSubtract 30 seconds for tank pressurization"
  # "The default:\nSubtract 180 seconds for Purge\nSubtract 12 second valve switch\nSubtract 30 seconds for tank pressurization"
  # "Need to reset time after purge (index 1)"
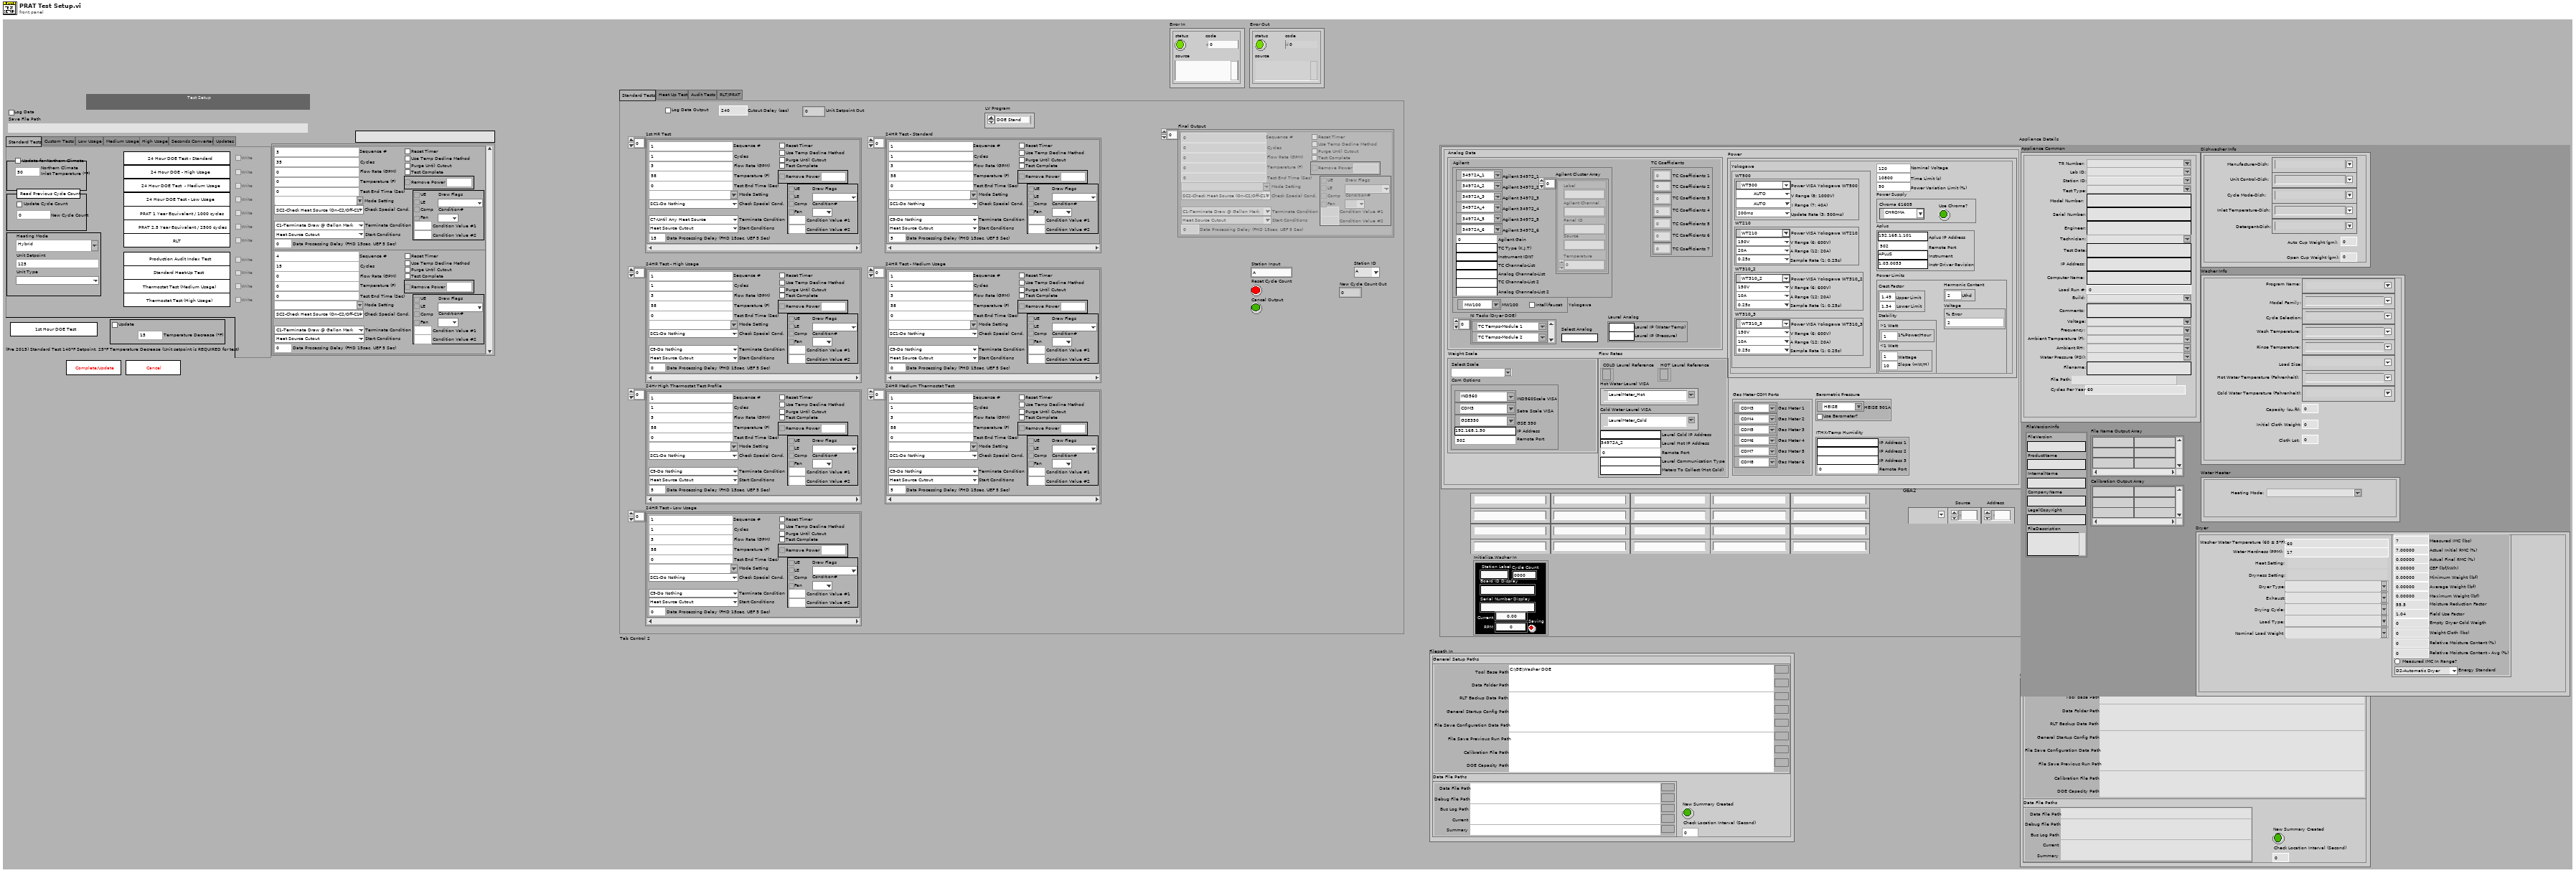
[diagram p1: front panel]
types:
  T1 = typedef "File Setup.lvlib/Save File DISH Dishwasher Details.ctl" = cluster{"FileVersionInfo":T2, "Dishwasher Info":cluster{"Open Cup Weight (gm):":dbl, "Auto Cup Weight (gm):":dbl, "Detergent-Dish:":string, "Inlet Temperature-Dish:":string, "Cycle Mode-Dish:":string, "Unit Control-Dish:":string, "Manufacturer-Dish:":string}, "Washer Info":cluster{"Hot Water Temperature (Fahrenheit):":string, "Cold Water Temperature (Fahrenheit):":string, "Capacity (cu.ft):":dbl, "Initial Cloth Weight:":dbl, "Cloth Lot:":i32, "Model Family:":string, "Program Name:":string, "Cycle Selection:":string, "Wash Temperature:":string, "Rinse Temperature:":string, "Load Size:":string}, "File Name Output Array":string[][], "Calibration Output Array":string[][], "Appliance Common":T3, "Water Heater":cluster{"Heating Mode:":string}, "Dryer":cluster{"Heat Setting:":T4, "Washer Water Temperature (60 ± 5°F):":u16, "Water Hardness (PPM):":u16, "Dryness Setting:":T4, "Dryer Type:":string, "Exhaust:":string, "Drying Cycle:":string, "Load Type:":string, "Nominal Load Weight":string, "Dryer Initial IMC Data":T5}}
  T2 = typedef "FileVersionInformation.ctl" = cluster{"FileVersion":string, "ProductName":string, "InternalName":string, "CompanyName":string, "LegalCopyright":string, "FileDescription":string}
  T3 = typedef "DOE Appliance Common.ctl" = cluster{"Engineer:":string, "Model Number:":string, "Serial Number:":string, "Comments:":string, "Station ID:":string, "Technician:":string, "TR Number:":string, "Lab ID:":string, "Voltage:":string, "Water Pressure (PSI):":string, "Test Date:":string, "Computer Name:":string, "IP Address:":string, "Ambient RH:":string, "Frequency:":string, "Build:":string, "Filename:":string, "Test Type:":string, "Load Run #:":i32, "Ambient Temperature (F):":string, "File Path:":path, "Cycles Per Year":u32}
  T4 = typedef "Custom Pallet String.ctl" = string
  T5 = typedef "DPT IMC Data.ctl" = cluster{"Measured IMC (lbs)":dbl, "Actual Initial RMC (%)":dbl, "RMC (Desired %)":dbl, "Bone Dry Wt(lbs)":dbl, "Tolerance(%)":dbl, "Actual Final RMC (%)":dbl, "CEF (lbf/kWh)":dbl, "Minimum Weight (lbf)":dbl, "Average Weight (lbf)":dbl, "Maximum Weight (lbf)":dbl, "Measured IMC In Range?":bool, "Moisture Reduction Factor":dbl, "Field Use Factor":dbl, "Empty Dryer Cold Weigth":dbl, "Energy Standard":T6, "Weight Cloth (lbs)":dbl, "Relative Moisture Content (%)":dbl, "Relative Moisture Content - Avg (%)":dbl}
  T6 = typedef "DOE Dryer Standard.ctl" = enum16{"D2-Automatic Dryer", "D2-Timer Dryer", "D1-Automatic Dryer", "D1-Timer Dryer", "Other"}
  T7 = typedef "File Setup.lvlib/Save File DOE File Path Control.ctl" = cluster{"General Setup Paths":cluster{"Calibration File Path":path, "DOE Capacity Path":path, "Data Folder Path":path, "RLT Backup Data Path":path, "Tool Base Path":path, "General Startup Config Path":path, "File Save Previous Run Path":path, "File Save Configuration Data Path":path}, "Data File Paths":T8, "New Summary Created":bool, "Check Location Interval (Second)":i32}
  T8 = typedef "File Setup.lvlib/Save File DOE Data Save Filepaths.ctl" = cluster{"Data File Path":path, "Debug File Path":path, "Bus Log Path":path, "Current":path, "Summary":path}
  T9 = typedef "DOE Main Control.ctl" = cluster{"Test Fixture Hardware":T10, "GEA2":T16, "DOE Capacity Measurments":T17, "Initialize.Washer In":T18}
  T10 = typedef "DOE Test Fixture Hardware.ctl" = cluster{"Power ":T11, "Weight Scale":cluster{"Com Options":T12, "Select Scale":string}, "Flow Rates":cluster{"Laurel Cold IP Address":string, "Laurel Hot IP Address":string, "Hot Water Laurel VISA":refnum<visa-resource-name>, "Cold Water Laurel VISA":refnum<visa-resource-name>, "Remote Port":u16, "Laurel Communication Type":string, "Meters To Collect (Hot Cold)":string, "HOT Laurel Reference":refnum<k5>, "COLD Laurel Reference":refnum<k5>}, "Analog Data":cluster{"Agilent":cluster{"Agilent 34972_1":refnum<visa-resource-name>, "Agilent 34972_2":refnum<visa-resource-name>, "Agilent 34972_3":refnum<visa-resource-name>, "Agilent 34972_4":refnum<visa-resource-name>, "Agilent 34972_5":refnum<visa-resource-name>, "Agilent 34972_6":refnum<visa-resource-name>, "Agilent Gain":dbl, "TC Type (K,J,T)":string, "Instrument IDN?":string, "TC Channels-List":string, "Analog Channels-List":string, "Agilent Cluster Array":T13[], "TC Channels-List 2":string, "Analog Channels-List 2":string}, "Yokogawa":cluster{"MW100":refnum<visa-resource-name>, "Intellifaucet":bool}, "Select Analog":string, "TC Coefficients":T14, "NI Tasks (Dryer DOE)":refnum<k21>[], "Laurel Analog":cluster{"Laurel IP (Water Temp)":string, "Laurel IP (Pressure)":string}}, "ITHX-Temp Humidity":cluster{"IP Address 1":string, "Remote Port":u16, "IP Address 2":string, "IP Address 3":string}, "Gas Meter COM Ports":T15, "Barometric Pressure":cluster{"HEISE 901A":refnum<visa-resource-name>, "Use Barometer?":bool}}
  T11 = typedef "UTILITY Power Inputs Control.ctl" = cluster{"Yokogawa":cluster{"WT210":cluster{"Sample Rate (1: 0.25s)":i32, "A Range (12: 20A)":i32, "V Range (6: 600V)":i32, "Power VISA Yokogawa WT210":refnum<visa-resource-name>}, "WT500":cluster{"Power VISA Yokogawa WT500":refnum<visa-resource-name>, "V Range (8: 1000V)":i32, "I Range (7: 40A)":i32, "Update Rate (3: 500ms)":i32}, "WT310_2":cluster{"Sample Rate (1: 0.25s)":i32, "A Range (12: 20A)":i32, "V Range (6: 600V)":i32, "Power VISA Yokogawa WT310_2":refnum<visa-resource-name>}, "WT310_3":cluster{"Sample Rate (1: 0.25s)":i32, "A Range (12: 20A)":i32, "V Range (6: 600V)":i32, "Power VISA Yokogawa WT310_3":refnum<visa-resource-name>}}, "Aplus":cluster{"Aplus IP Address":string, "Remote Port":i32, "Instrument":string, "Instr Driver Revision":string}, "Power Limits":cluster{"Crest Factor":cluster{"Upper Limit":dbl, "Lower Limit":dbl}, "Harmonic Content":cluster{"Uthd":dbl}, "Voltage":cluster{"% Error":dbl}, "Stability":cluster{"<1 Watt ":cluster{"Wattage":dbl, "Slope (mW/H)":dbl}, ">1 Watt":cluster{"1%Power/Hour":dbl}}}, "Nominal Voltage":i32, "Time Limit (s)":dbl, "Power Variation Limit (%)":dbl, "Power Supply":cluster{"Chroma 61605":refnum<visa-resource-name>, "Use Chroma?":bool}}
  T12 = typedef "IND560 Configuration.ctl" = cluster{"IND560Scale VISA":refnum<visa-resource-name>, "IP Address":string, "Remote Port":u16, "Setra Scale VISA":refnum<visa-resource-name>, "GSE 350":refnum<visa-resource-name>}
  T13 = typedef "HEWH Agilent Cluster.ctl" = cluster{"Label":string, "Agilent Channel":string, "Panel ID":string, "Source":string, "Temperature":dbl}
  T14 = typedef "UTILITY TC Coefficients.ctl" = cluster{"TC Coefficients 1":dbl[], "TC Coefficients 2":dbl[], "TC Coefficients 3":dbl[], "TC Coefficients 4":dbl[], "TC Coefficients 5":dbl[], "TC Coefficients 6":dbl[], "TC Coefficients 7":dbl[]}
  T15 = typedef "FMA1600A COM Ports.ctl" = cluster{"Gas Meter 1":refnum<visa-resource-name>, "Gas Meter 2":refnum<visa-resource-name>, "Gas Meter 3":refnum<visa-resource-name>, "Gas Meter 4":refnum<visa-resource-name>, "Gas Meter 5":refnum<visa-resource-name>, "Gas Meter 6":refnum<visa-resource-name>}
  T16 = typedef "GEA2.ctl" = cluster{"Address":u8, "Source":u8, "Viper/Hawk":u8}
  T17 = typedef "DOE Capacity Measurments.ctl" = cluster{"Weight 1":dbl, "Model Number 1":string, "Temp 1":dbl, "Serial Number 1":string, "Lab Number 1":string, "Lab Number 2":string, "Serial Number 2":string, "Temp 2":dbl, "Model Number 2":string, "Weight 2":dbl, "Lab Number 3":string, "Serial Number 3":string, "Temp 3":dbl, "Model Number 3":string, "Weight 3":dbl, "Lab Number 4":string, "Serial Number 4":string, "Temp 4":dbl, "Model Number 4":string, "Weight 4":dbl, "Capacity Measurment Output String":string[][]}
  T18 = typedef "Save File.lvlib/Save File Washer.ctl" = cluster{"Appliance Details":T1, "Display Data (RLT)":T19}
  T19 = typedef "Save File Appliance Display.ctl" = cluster{"Status Color":u32, "Serial Number Display":string, "Cycle Count Display":i32, "Station Label Display":string, "Current Run Start Time Display":dbl, "Board ID Display":string, "RPM Display":u32, "Current Display":dbl, "Current Path Display":path, "Saving Display":bool, "Unit Type Display":T20, "Total Time On Display":dbl, "UI Button":bool}
  T20 = typedef "Save File.lvlib/Save File Unit Type.ctl" = enum32{"", "Viper", "Hawk", "2015"}
  T21 = typedef "PRAT Test.ctl" = cluster{"Sequence #":dbl, "Cycles":i32, "Mode Setting":T22, "Flow Rate (GPM)":dbl, "Temperature (F)":dbl, "Reset Timer":bool, "Use Temp Decline Method":bool, "Terminate Condition":T23, "Condition Value #1":dbl, "UE":bool, "LE":bool, "Comp":bool, "Fan":bool, "Test End Time (Sec)":dbl, "Purge Until Cutout":bool, "Start Conditions":T24, "Condition Value #2":dbl, "Remove Power":bool, "Time":dbl, "Check Special Cond.":T25, "Condition#":T26, "Draw Flags":T27, "Data Processing Delay (FHD 15sec, UEF 5 Sec)":dbl, "Test Complete":bool}
  T22 = typedef "File Setup.lvlib/Save File HEWH Heating Control Mode.ctl" = string
  T23 = typedef "Terminate Draw Conditions.ctl" = enum16{"C1-Terminate Draw @ Gallon Mark", "C2-Special Last Draw (HU Test)", "C3-RTD Out <=", "C4-Mean Tank Temp <=", "C5-Decrease RTD Out (Deg F)", "C6-Time (Seconds)", "C7-Until Any Heat Source", "C8-Specific Heat Source", "C9-Do Nothing"}
  T24 = typedef "HEWH Start Conditions.ctl" = enum16{"Heat Source Cutout", "At Time (Seconds)", "Every X (Seconds)", "T2 >= X° Below Setpoint", "Seconds From Complete", "Wait for LE & Comp Cutout", "Wait for Comp Cutout", "Wait for LE Cutout", "Wait for UE Cutout"}
  T25 = typedef "Check Special Condtions.ctl" = enum16{"SC1-Do Nothing", "SC2-Check Heat Source (On-C2/Off-C1)", "SC3-Check Skip Condition", "SC4-Check Heat Source ON/Fail"}
  T26 = typedef "HEWH Special Condition Check.ctl" = enum16{"N/A", "C1", "C2", "Reset/Fail", "Skip Draw Sequence"}
  T27 = typedef "HEWH Draw Flag ENUM.ctl" = enum16{"N/A", "None(0)", "Sml(1)", "Med(2)", "SmlMed(3)", "Lrg(4)", "SmlLrg(5)", "MedLrg(6)", "SmlMedLrg(7)"}
  T28 = enum32{"Standard Tests", "Custom Tests", "Low Usage", "Medium Usage", "High Usage", "Seconds Converter", "Updates"}
  T29 = typedef "Unit Type.ctl" = enum16{"", "50 Gallon", "80 Gallon"}
  T30 = enum32{"Standard Tests", "Heat Up Test", "Audit Tests", "RLT/PRAT"}
  T31 = typedef "Station ID Selector.ctl" = enum16{"", "A", "B", "C", "D", "Global"}
  T32 = typedef "File Setup.lvlib/Save File DOE LabView Program.ctl" = enum16{"No Name Found", "DOE Stand", "Dishwasher Kitchen", "Portable Stand", "HEWH", "Dryer", "Dryer WILT", "HCC", "PRAT", "HEWH RLT", "Refrigeration"}
  T33 = enum8{"Enabled", "Disabled", "Disabled and Grayed Out"}
  T34 = typedef "File Setup.lvlib/Save File DOE Configuration State.ctl" = enum16{"Open Front Panel", "Load Config"}
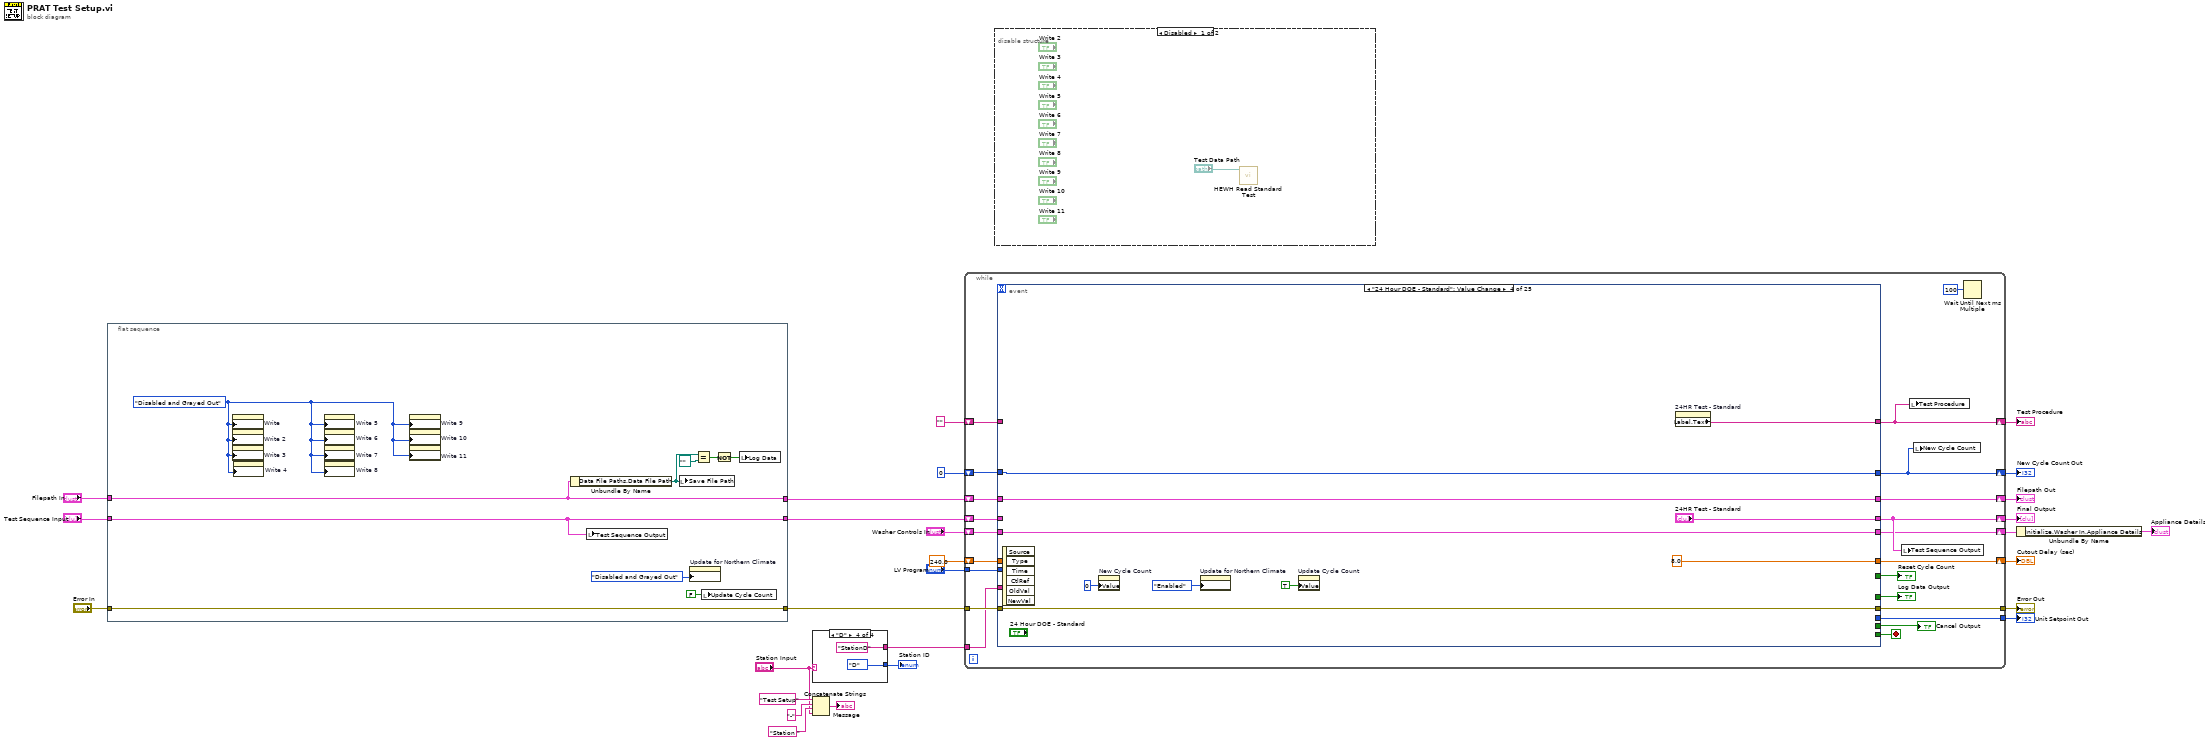
[diagram p0: block diagram]
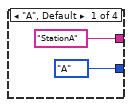
[diagram p3: hidden frame]
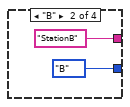
[diagram p4: hidden frame]
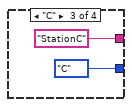
[diagram p5: hidden frame]
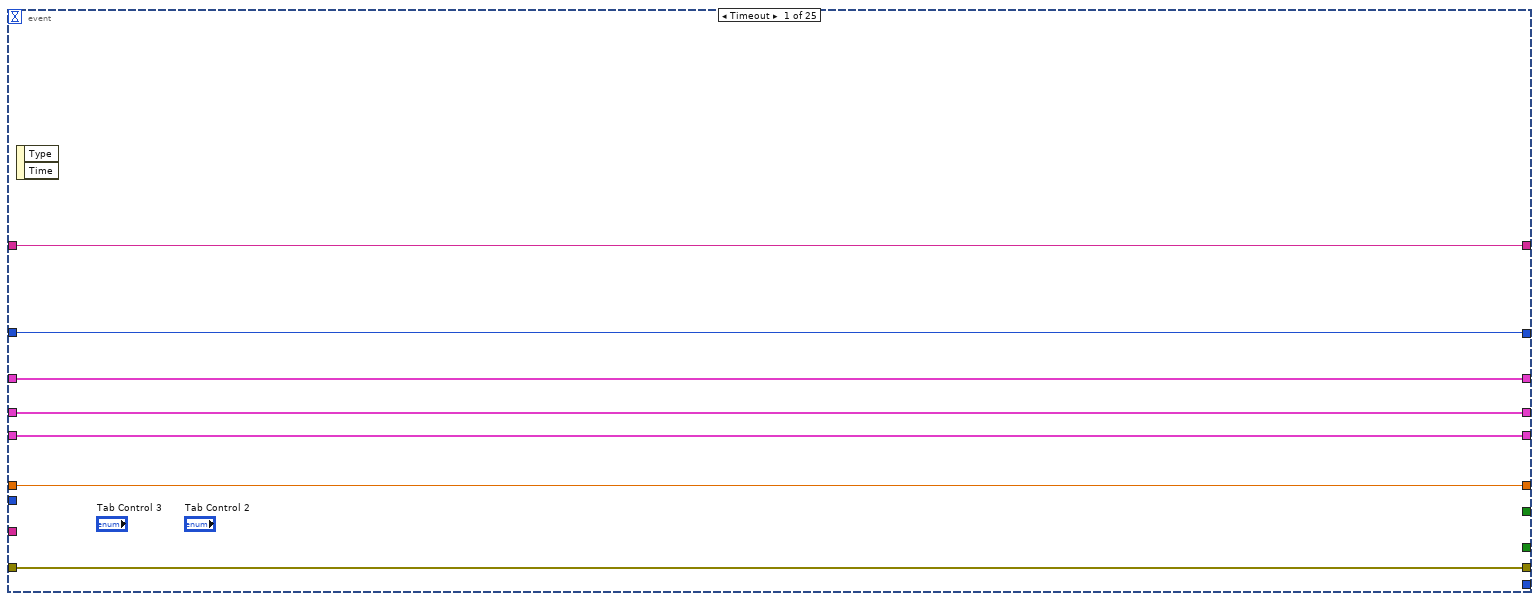
[diagram p6: hidden frame]
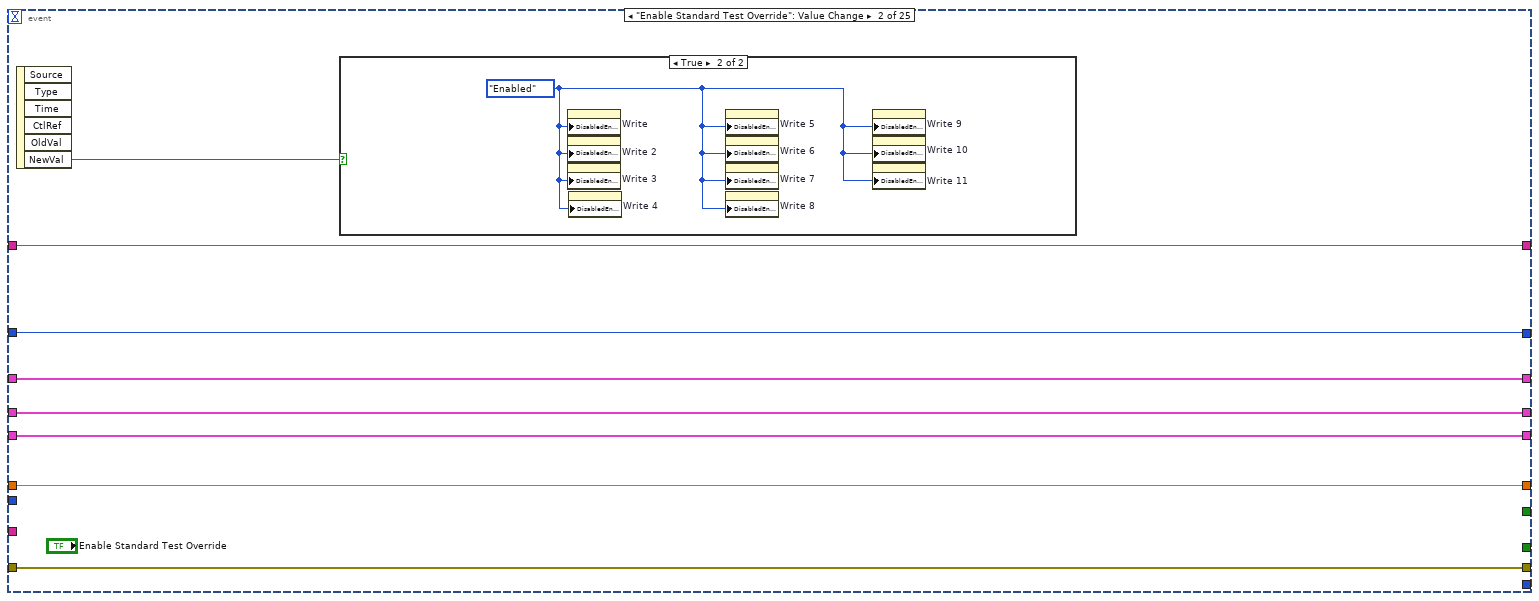
[diagram p7: hidden frame]
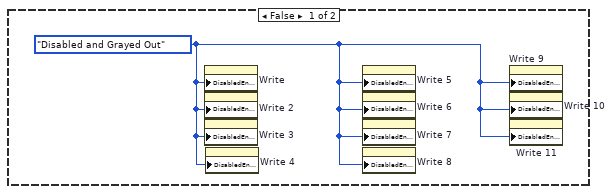
[diagram p8: hidden frame]
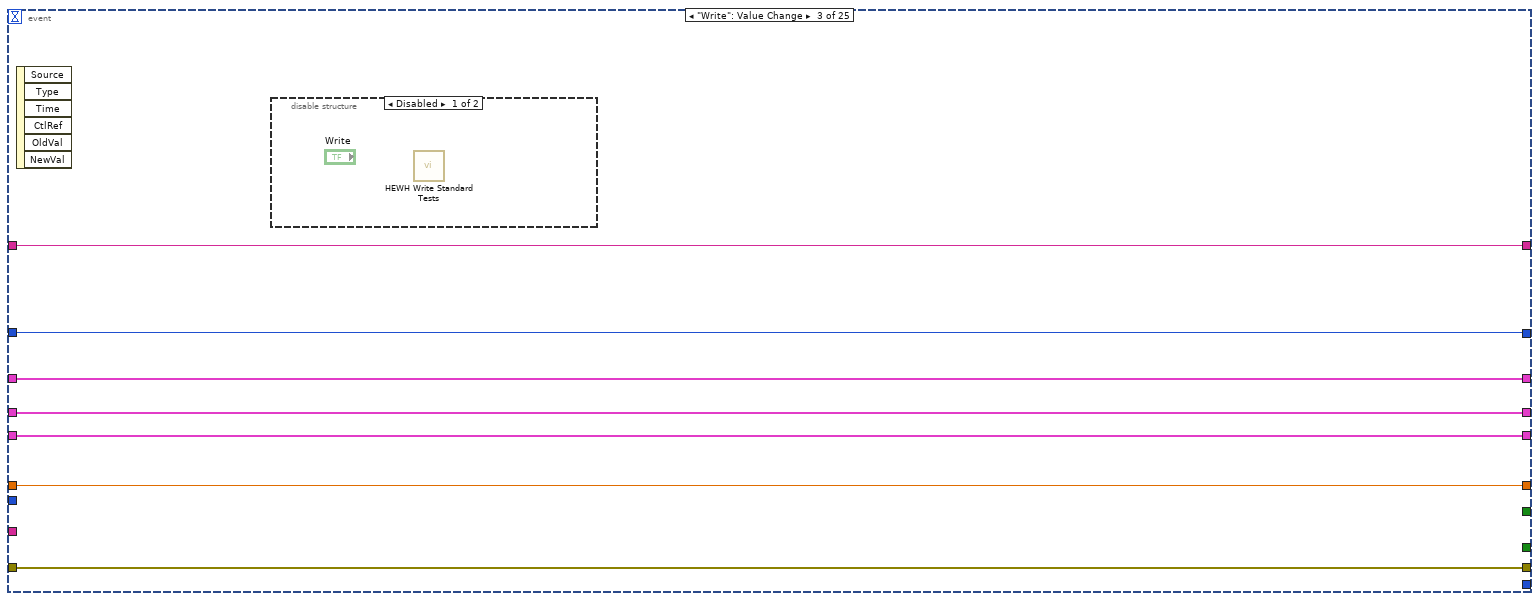
[diagram p9: hidden frame]
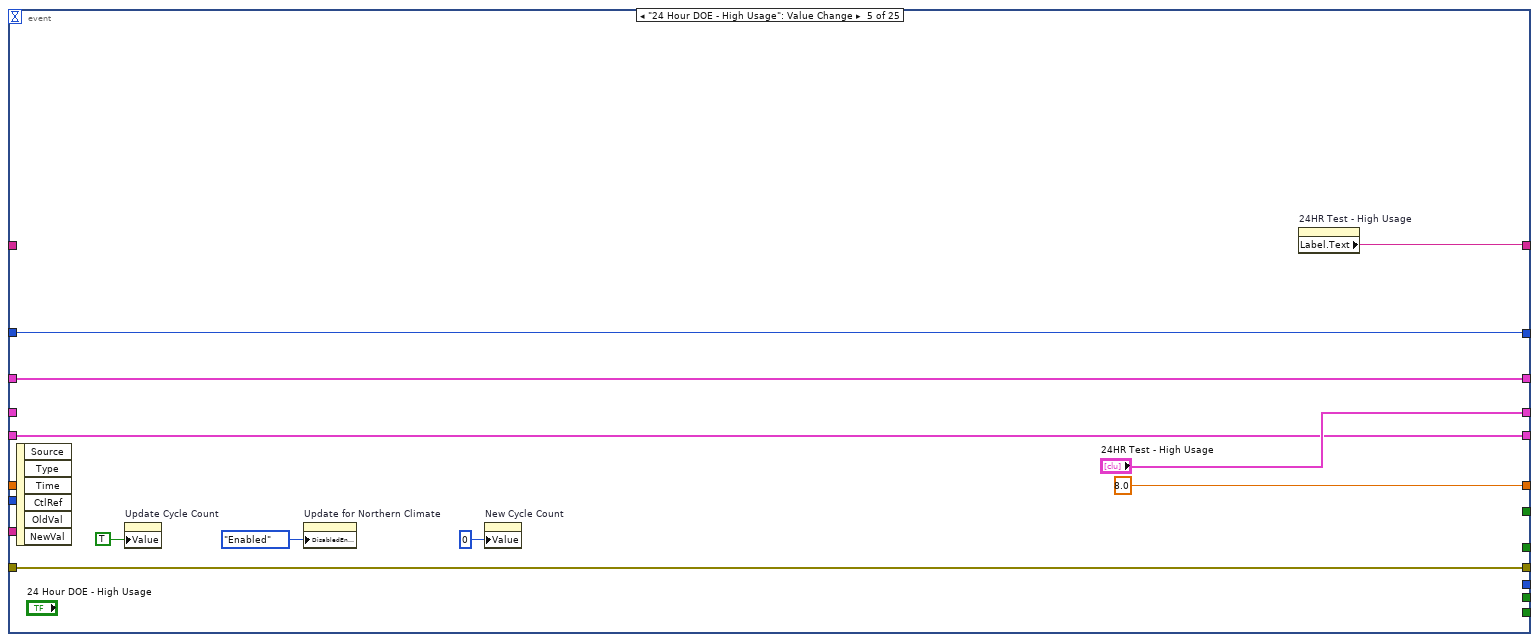
[diagram p11: hidden frame]
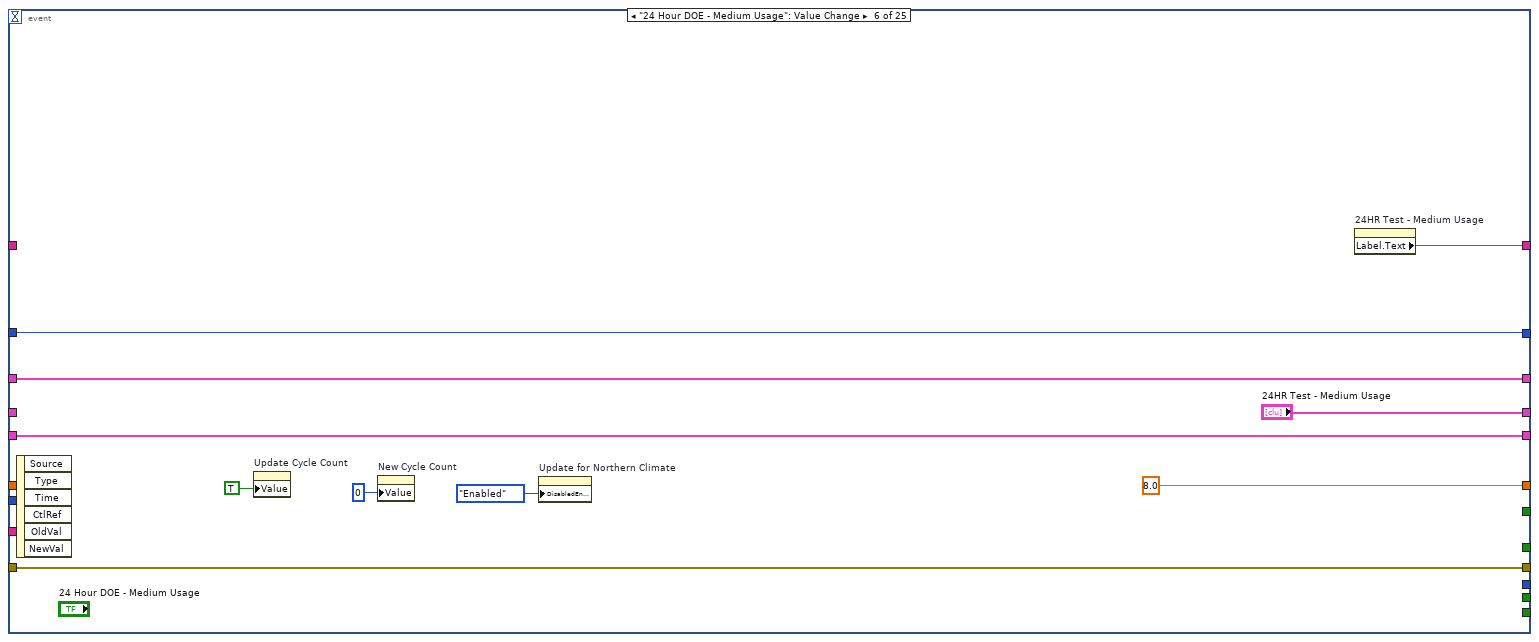
[diagram p12: hidden frame]
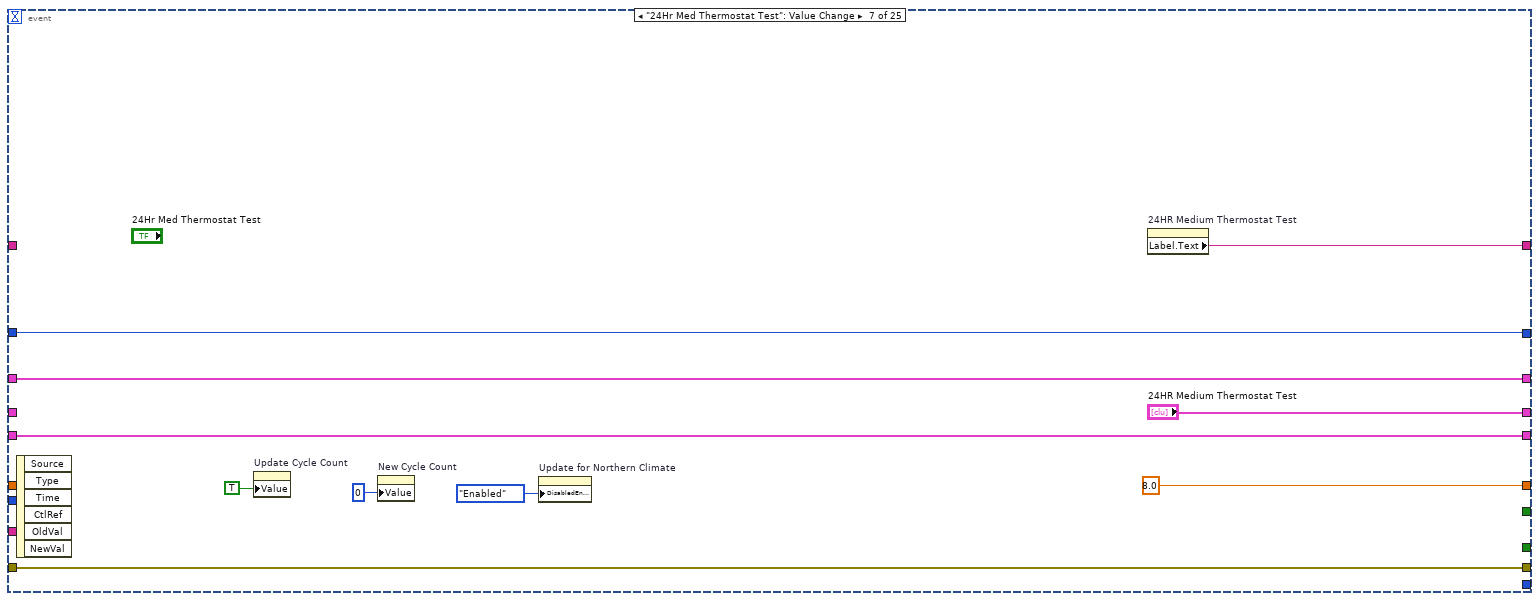
[diagram p13: hidden frame]
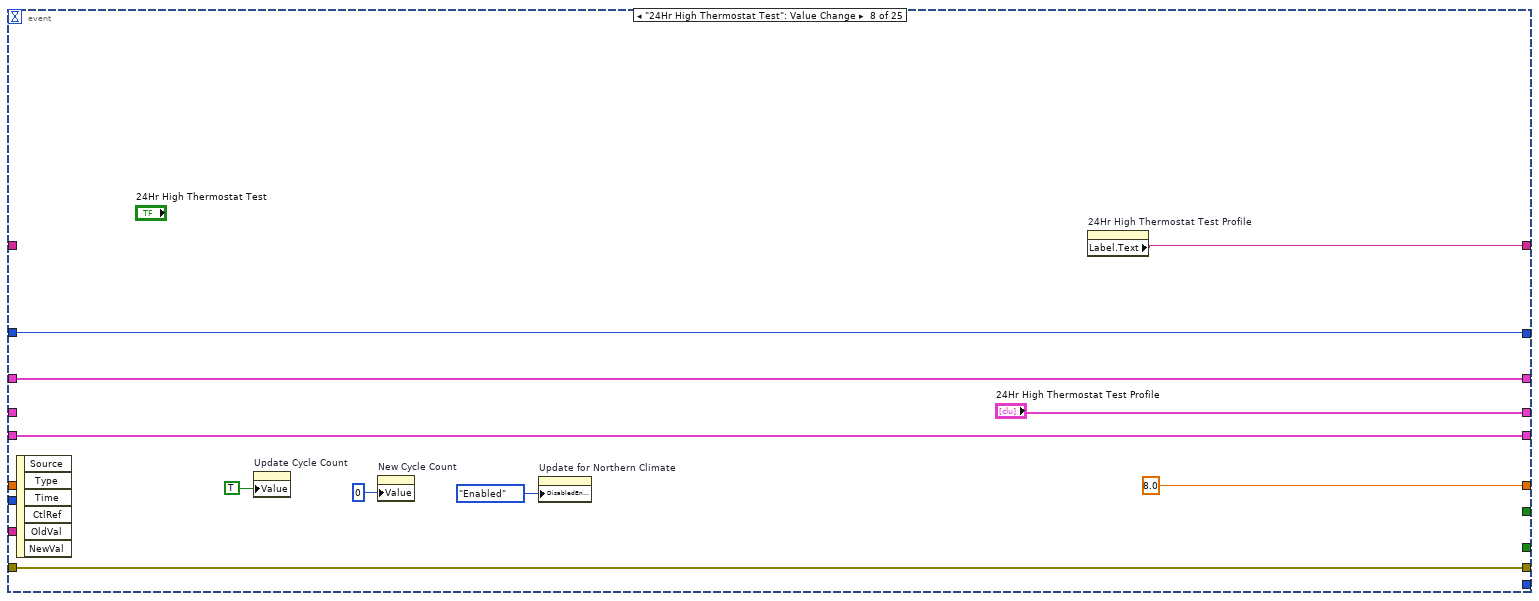
[diagram p14: hidden frame]
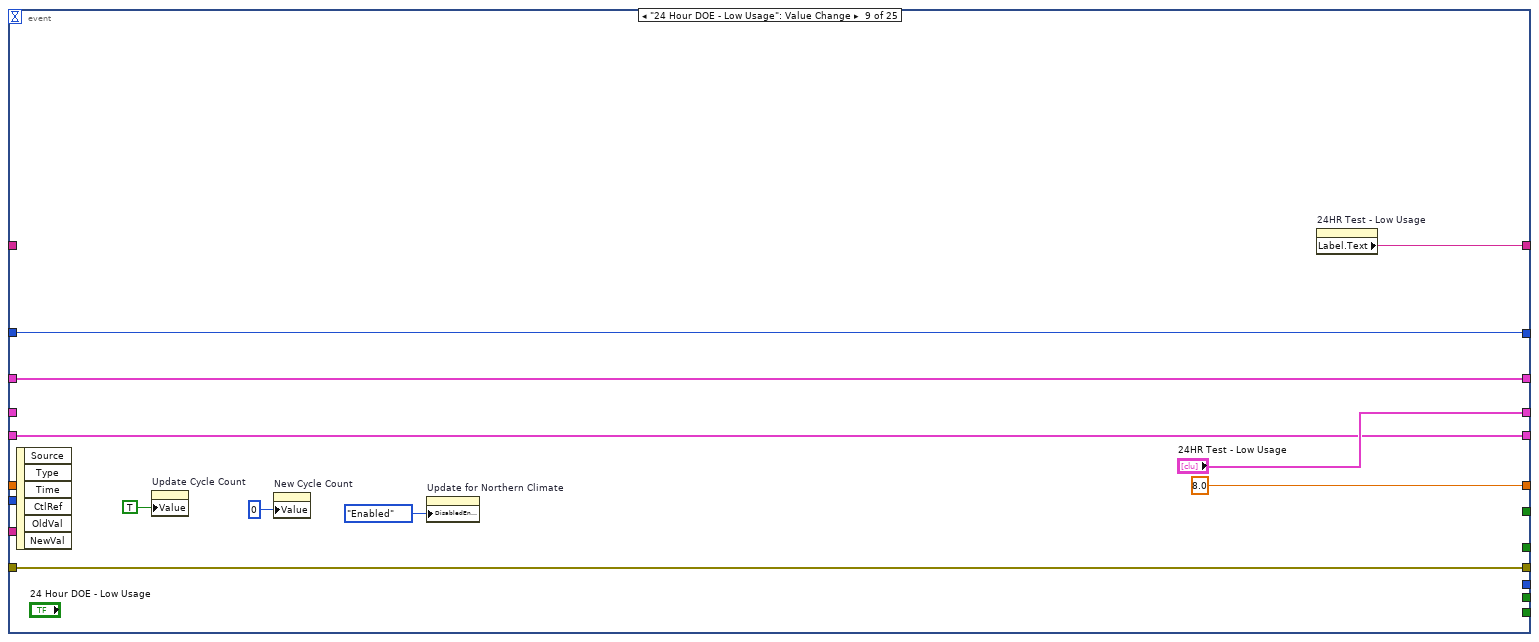
[diagram p15: hidden frame]
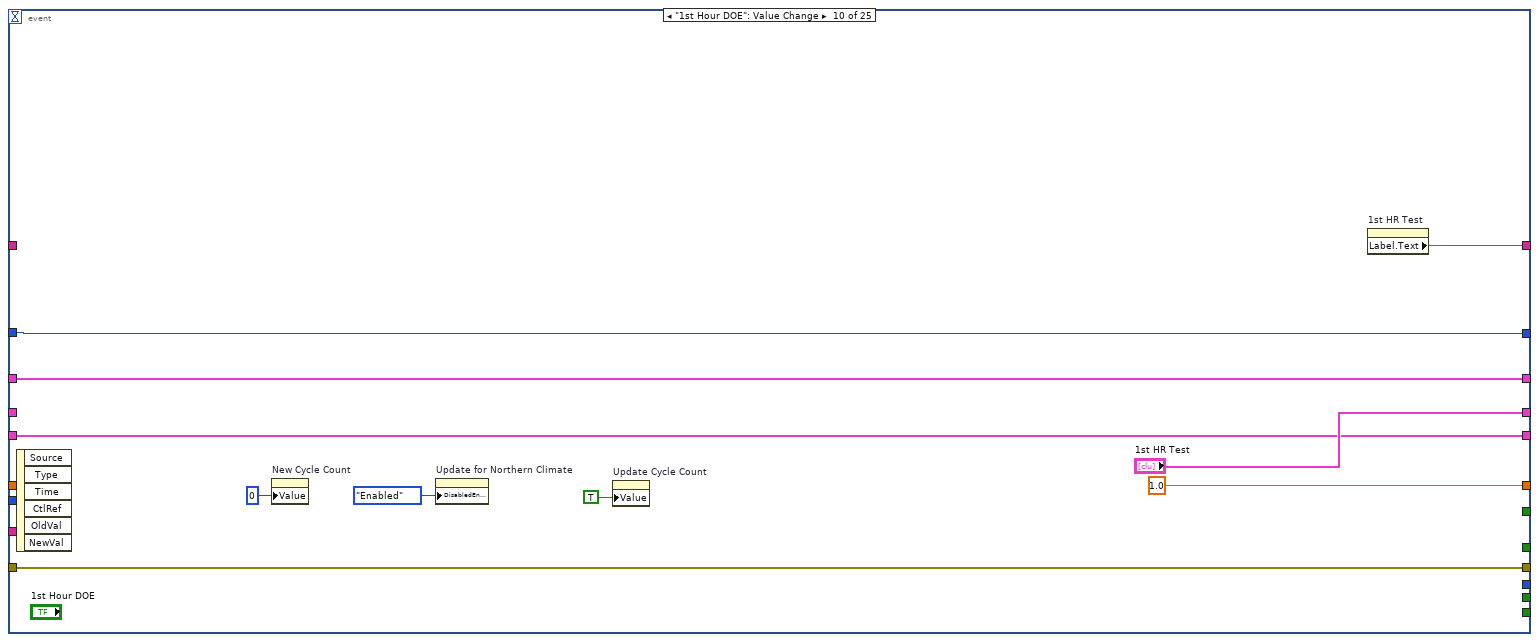
[diagram p16: hidden frame]
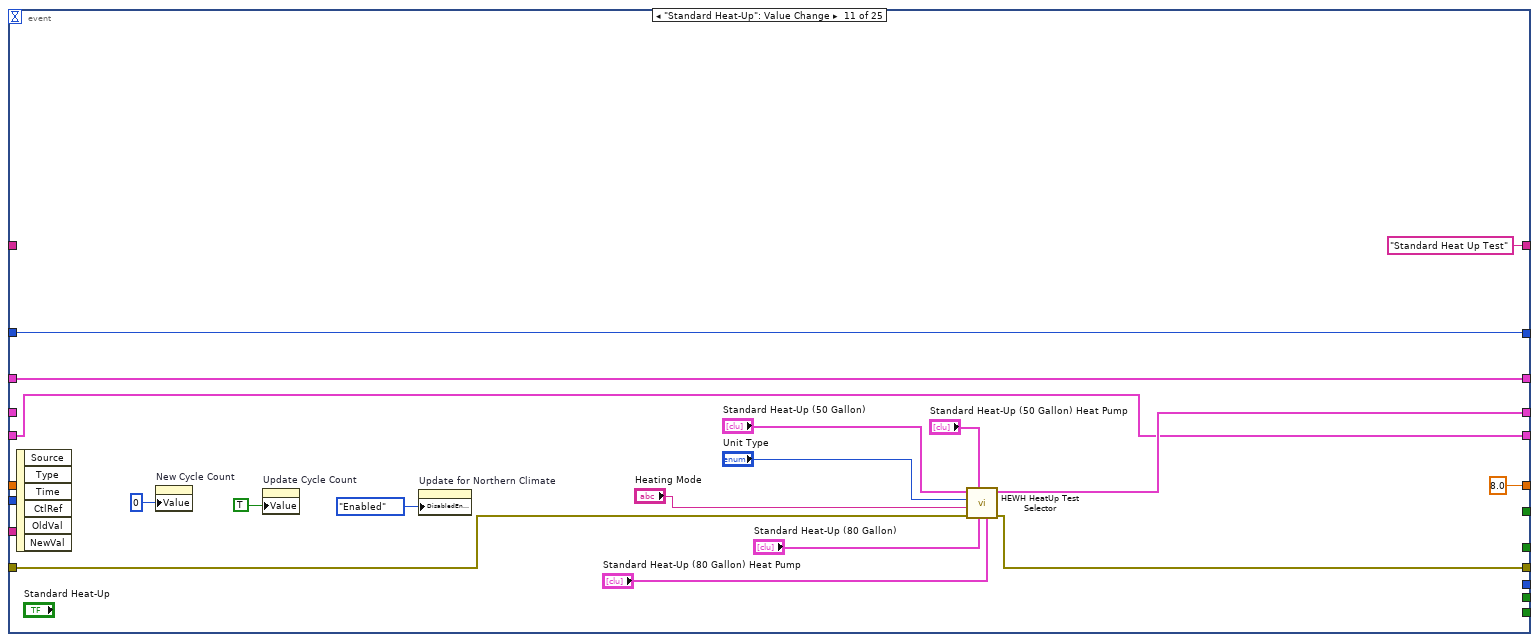
[diagram p17: hidden frame]
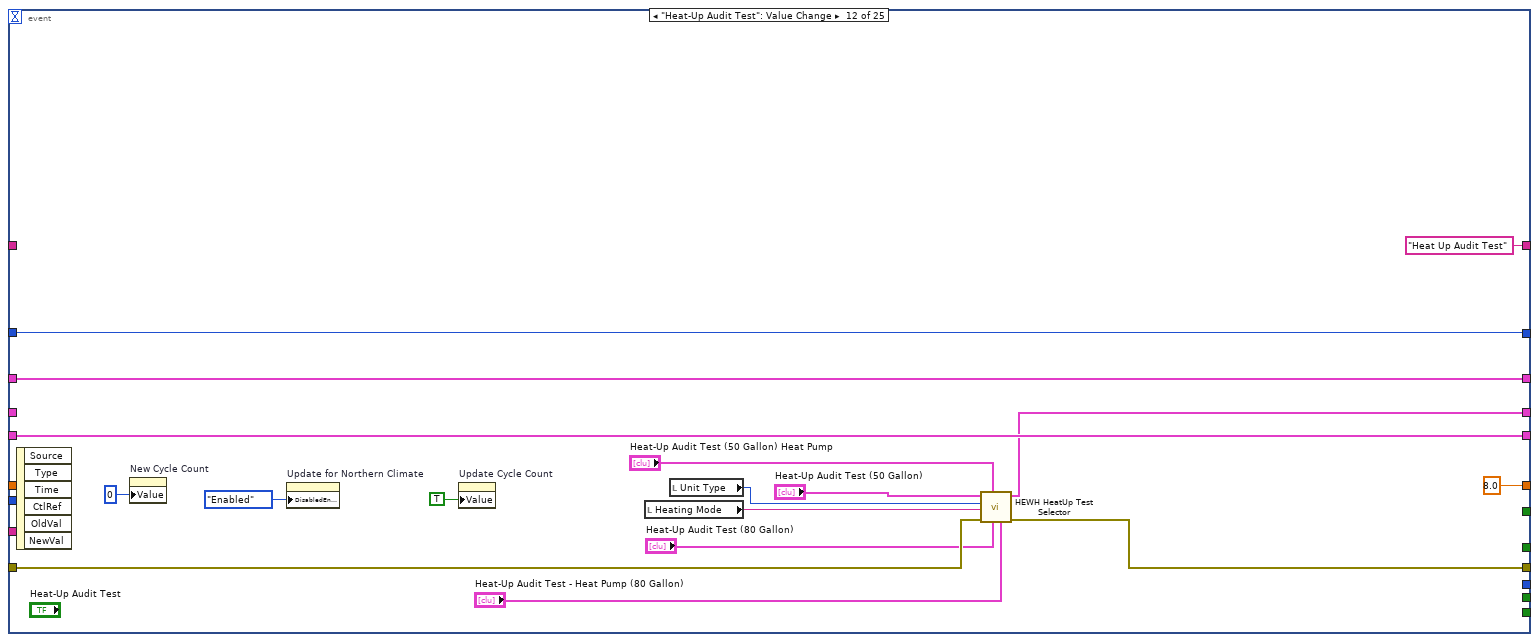
[diagram p18: hidden frame]
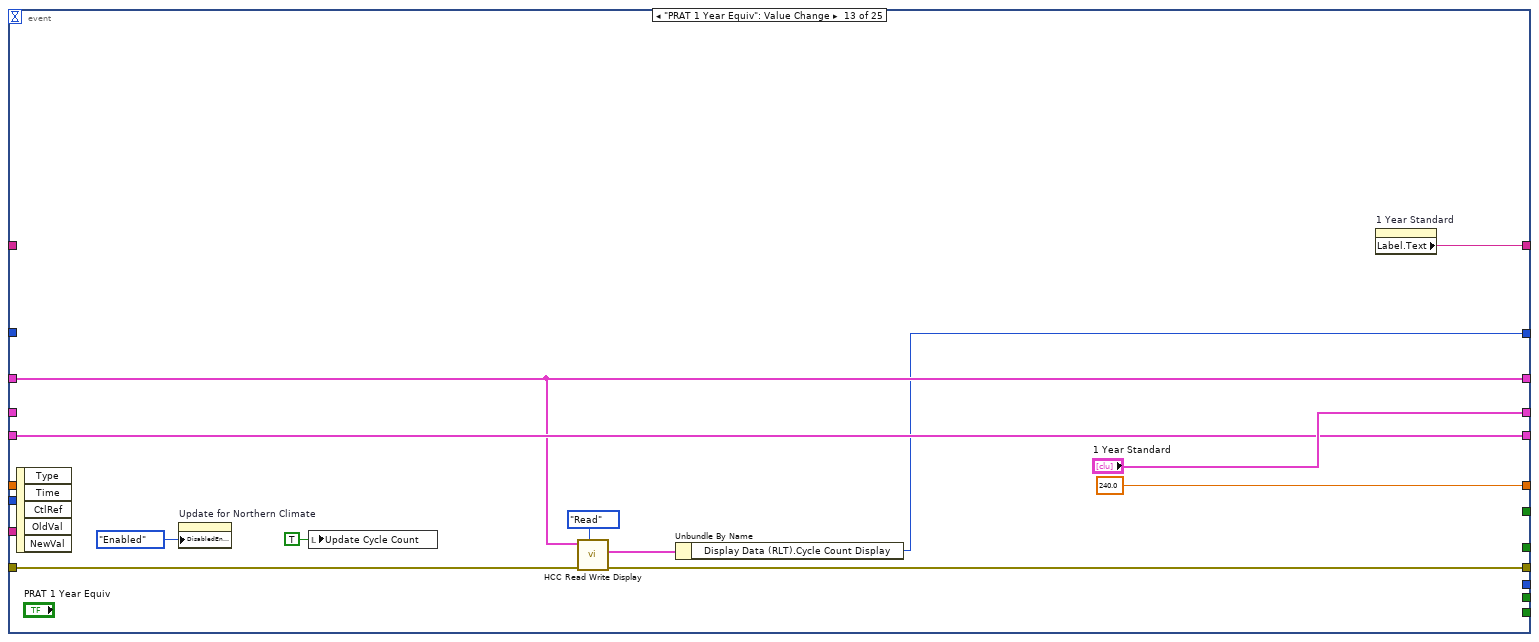
[diagram p19: hidden frame]
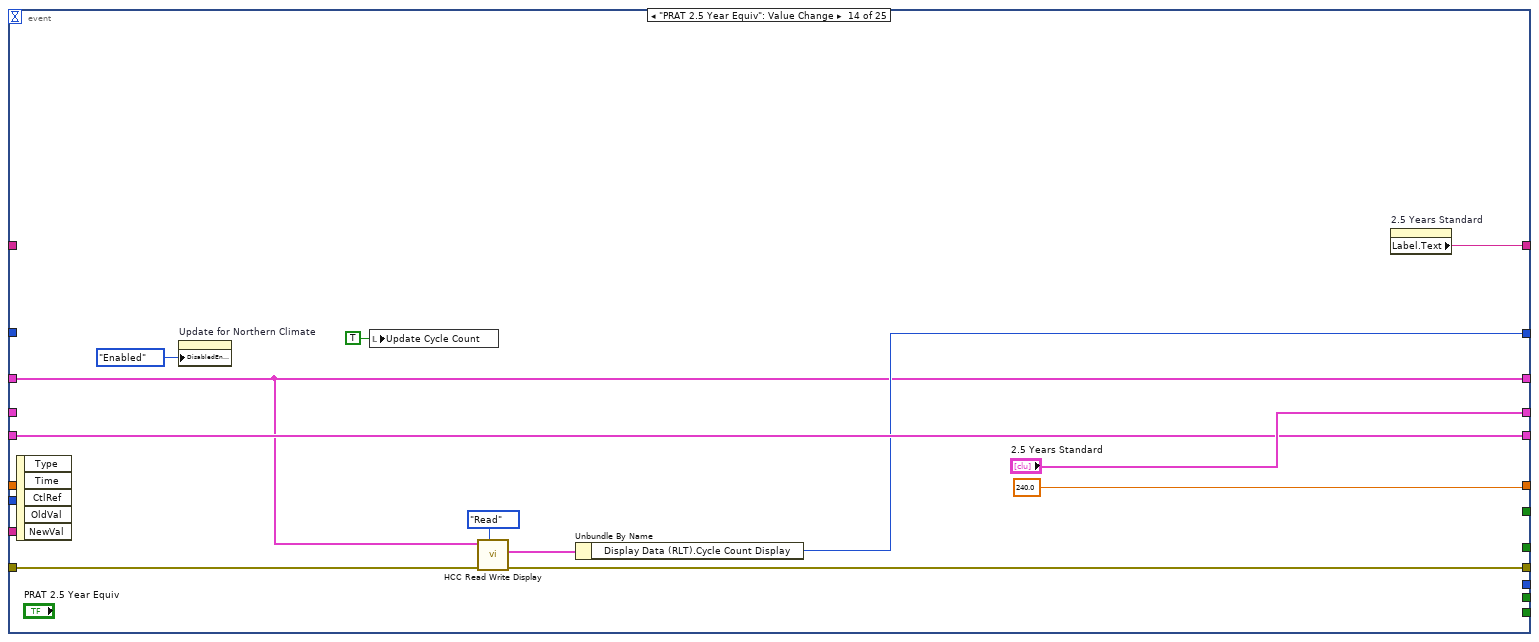
[diagram p20: hidden frame]
diagram:
  n1 = flat-sequence {
    tunnel: "Error In" -> [w37]
    tunnel: [w37] -> w19
    tunnel: "Test Sequence Input" -> [w35]
    tunnel: [w35] -> w17
    tunnel: "Filepath In" -> [w33]
    tunnel: [w33] -> w12
    frame #0 {
      w28 = T33."Disabled and Grayed Out" ("Disabled")
      n2 = property on="Write" class="Bool"("DisabledEnum"=w28) -> ()  [unwired: 2 in, 2 out]
      n3 = property on="Write 2" class="Bool"("DisabledEnum"=w28) -> ()  [unwired: 2 in, 2 out]
      n4 = property on="Write 3" class="Bool"("DisabledEnum"=w28) -> ()  [unwired: 2 in, 2 out]
      n5 = property on="Write 4" class="Bool"("DisabledEnum"=w28) -> ()  [unwired: 2 in, 2 out]
      n6 = property on="Write 5" class="Bool"("DisabledEnum"=w28) -> ()  [unwired: 2 in, 2 out]
      n7 = property on="Write 6" class="Bool"("DisabledEnum"=w28) -> ()  [unwired: 2 in, 2 out]
      n8 = property on="Write 7" class="Bool"("DisabledEnum"=w28) -> ()  [unwired: 2 in, 2 out]
      n9 = property on="Write 8" class="Bool"("DisabledEnum"=w28) -> ()  [unwired: 2 in, 2 out]
      n10 = property on="Write 9" class="Bool"("DisabledEnum"=w28) -> ()  [unwired: 2 in, 2 out]
      n11 = property on="Write 10" class="Bool"("DisabledEnum"=w28) -> ()  [unwired: 2 in, 2 out]
      n12 = property on="Write 11" class="Bool"("DisabledEnum"=w28) -> ()  [unwired: 2 in, 2 out]
      n13 = Unbundle By Name(w33) -> ("Data File Paths.Data File Path"=w32:path)
      n14 = local write "Test Sequence Output"(w35) -> ()
      n15 = local write "Save File Path"(w32) -> ()
      n16 = property on="Update for Northern Climate" class="Bool"("DisabledEnum"=T33."Disabled and Grayed Out" ("Disabled")) -> ()  [unwired: 2 in, 2 out]
      n17 = Equal?(x=w32, y=path "") -> (x = y?=w30:bool)
      n18 = local write "Update Cycle Count"(FALSE ("Update Cycle Count")) -> ()
      n19 = Not(x=w30) -> (.not. x?=w29:bool)
      n20 = local write "Log Data"(w29) -> ()
    }
  }
  n21 = case shown="\"D\"" "Station Input" {
    tunnel: [Station_ID_Selector."A" ("Station ID") Station_ID_Selector."B" ("Station ID") Station_ID_Selector."C" ("Station ID") Station_ID_Selector."D" ("Station ID")] -> w22
    tunnel: ["StationA" "StationB" "StationC" "StationD"] -> w8
    frame "A", Default {
    }
    frame "B" {
    }
    frame "C" {
    }
    frame "D" {
    }
  }
  "Station ID" <- w22
  n22 = Concatenate Strings("Test Setup" ("string"), "-" ("string"), "Station " ("string"), "Station Input") -> (→"Message":string)
  n23 = while {
    tunnel: w19 -> [w60]
    tunnel: [w59] -> w27
    shift-right: [w62] -> w16
    shift-left: w17 -> [w65]
    tunnel: "LV Program" -> [w57]
    tunnel: w8 -> [w53]
    shift-right: [w54] -> w11
    shift-left: w12 -> [w58]
    shift-right: [w55] -> w10
    shift-left: "Washer Controls In" -> [w56]
    shift-right: [w52] -> w6
    shift-left: 240.0 ("Cutout Delay (sec)") -> [w51]
    tunnel: [w50] -> w5
    shift-right: [w49] -> w4
    shift-left: 0 ("New Cycle Count 2") -> [w48]
    shift-right: [w46] -> w1
    shift-left: "" -> [w47]
    stop <- w66 stop-if-true
    n24 = event shown="[3] \"24 Hour DOE - Standard\": Value Change" {
      selector: _ -> [_ _ _ _ _ _ _ _ _ _ _ _ _ _ _ _ _ _ _ _ _ _ _ _ _]
      dyn-events: _ -> [_ _ _ _ _ _ _ _ _ _ _ _ _ _ _ _ _ _ _ _ _ _ _ _ _]
      timeout: _ -> [_ _ _ _ _ _ _ _ _ _ _ _ _ _ _ _ _ _ _ _ _ _ _ _ _]
      tunnel: [_ _ _ _ _ _ _ _ _ _ _ _ _ _ _ _ TRUE w260 _ _ _ _ _ _ _] -> w66
      tunnel: [w74 w79 w88 "24HR Test - Standard" "24HR Test - High Usage" "24HR Test - Medium Usage" "24HR Medium Thermostat Test" "24Hr High Thermostat Test Profile" "24HR Test - Low Usage" "1st HR Test" w177 w183 "1 Year Standard" "2.5 Years Standard" "RLT" "Custom Test" w251 w259 w268 "Test Sequence Output" w293 w317 w328 _ _] -> w62
      tunnel: w65 -> [w74 w79 w88 _ _ _ _ _ _ _ _ _ _ _ _ _ w251 w259 w269 _ w293 w317 w329 _ _]
      tunnel: [_ _ _ _ _ _ _ _ _ _ _ _ _ _ _ _ "Update Cycle Count" FALSE ("Update Cycle Count") _ _ _ _ _ _ _] -> w64
      tunnel: [_ _ _ _ _ _ _ _ _ _ _ _ _ _ _ _ FALSE w260 _ _ _ _ _ _ _] -> w63
      tunnel: [w69 w81 w91 w93 w103 w113 w124 w134 w143 w153 w171 w189 w198 w212 w222 w233 "New Cycle Count" w253 w262 w277 w284 w318 w324 _ _] -> w49
      tunnel: [_ _ _ _ _ _ _ _ _ _ _ _ _ _ _ _ "Log Data" _ _ _ _ _ _ _ _] -> w61
      tunnel: w60 -> [w73 w77 w85 w97 w107 w117 w128 w138 w147 w157 w168 w188 w200 w211 w224 w237 w246 w258 w266 w281 w295 w322 w330 w341 w345]
      tunnel: [w73 w77 w85 w97 w107 w117 w128 w138 w147 w157 w167 w187 w199 w210 w223 w237 w246 w258 w266 w281 w294 w321 w330 w340 w345] -> w59
      tunnel: w58 -> [w72 w80 w89 w96 w106 w116 w127 w137 w146 w156 w174 w192 w201 w209 w221 w236 w245 w257 w265 w280 w292 w316 w326 _ _]
      tunnel: w57 -> [_ _ _ _ _ _ _ _ _ _ _ _ _ _ _ _ _ _ _ _ w291 _ _ _ _]
      tunnel: w56 -> [w71 w78 w87 w95 w105 w115 w126 w136 w145 w155 w173 w191 w205 w217 w229 w235 w244 w256 w264 w279 w290 w315 w327 _ _]
      tunnel: [w71 w78 w87 w95 w105 w115 w126 w136 w145 w155 w173 w191 w205 w217 w229 w235 w244 w256 w264 w279 w289 w315 w327 _ _] -> w55
      tunnel: [w72 w80 w89 w96 w106 w116 w127 w137 w146 w156 w174 w192 w201 w209 w221 w236 w245 w257 w265 w280 w288 w316 w326 _ _] -> w54
      tunnel: w53 -> [_ _ _ _ _ _ _ _ _ _ _ _ _ _ _ _ _ _ _ _ _ _ _ _ _]
      tunnel: [w70 w76 w86 8.0 ("Cutout Delay (sec)") 8.0 ("Cutout Delay (sec)") 8.0 ("Cutout Delay (sec)") 8.0 ("Cutout Delay (sec)") 8.0 ("Cutout Delay (sec)") 8.0 ("Cutout Delay (sec)") 1.0 ("Cutout Delay (sec)") 8.0 ("Cutout Delay (sec)") 8.0 ("Cutout Delay (sec)") 240.0 ("Cutout Delay (sec)") 240.0 ("Cutout Delay (sec)") 240.0 ("Cutout Delay (sec)") 8.0 ("Cutout Delay (sec)") w242 w255 w263 w278 w285 w314 8.0 ("Cutout Delay (sec)") _ _] -> w52
      tunnel: w51 -> [w70 w76 w86 _ _ _ _ _ _ _ _ _ _ _ _ _ w242 w255 w263 w278 w285 w314 _ _ _]
      tunnel: [_ _ _ _ _ _ _ _ _ _ _ _ _ _ _ _ "Unit Setpoint" _ _ _ _ _ _ _ _] -> w50
      tunnel: w48 -> [w69 w81 w91 w93 w103 w113 w124 w134 w143 w153 w171 w189 _ _ _ w233 _ w253 w262 w277 w284 _ w324 _ _]
      tunnel: [w68 w82 w90 w92 w102 w112 w123 w132 w142 w152 "Standard Heat Up Test" ("Label.Text") "Heat Up Audit Test" ("Label.Text") w196 w208 w220 w232 w240 w252 w261 "Custom Test" ("Label.Text") w283 w313 w323 _ _] -> w46
      tunnel: w47 -> [w68 w82 w90 _ _ _ _ _ _ _ _ _ _ _ _ _ w240 w252 w261 _ w283 w313 w323 _ _]
      event Timeout {
        n25 = event-data() -> ()  [unwired: 1 in, 2 out]
      }
      event "Enable Standard Test Override": Value Change {
        n26 = event-data() -> ("NewVal"=w75:bool)  [unwired: 1 in, 5 out]
        n27 = case shown="True" w75 {
          frame False {
            w83 = T33."Disabled and Grayed Out" ("Disabled")
            n28 = property on="Write" class="Bool"("DisabledEnum"=w83) -> ()  [unwired: 2 in, 2 out]
            n29 = property on="Write 2" class="Bool"("DisabledEnum"=w83) -> ()  [unwired: 2 in, 2 out]
            n30 = property on="Write 3" class="Bool"("DisabledEnum"=w83) -> ()  [unwired: 2 in, 2 out]
            n31 = property on="Write 4" class="Bool"("DisabledEnum"=w83) -> ()  [unwired: 2 in, 2 out]
            n32 = property on="Write 5" class="Bool"("DisabledEnum"=w83) -> ()  [unwired: 2 in, 2 out]
            n33 = property on="Write 6" class="Bool"("DisabledEnum"=w83) -> ()  [unwired: 2 in, 2 out]
            n34 = property on="Write 7" class="Bool"("DisabledEnum"=w83) -> ()  [unwired: 2 in, 2 out]
            n35 = property on="Write 8" class="Bool"("DisabledEnum"=w83) -> ()  [unwired: 2 in, 2 out]
            n36 = property on="Write 9" class="Bool"("DisabledEnum"=w83) -> ()  [unwired: 2 in, 2 out]
            n37 = property on="Write 10" class="Bool"("DisabledEnum"=w83) -> ()  [unwired: 2 in, 2 out]
            n38 = property on="Write 11" class="Bool"("DisabledEnum"=w83) -> ()  [unwired: 2 in, 2 out]
          }
          frame True {
            w84 = T33."Enabled" ("Disabled")
            n39 = property on="Write" class="Bool"("DisabledEnum"=w84) -> ()  [unwired: 2 in, 2 out]
            n40 = property on="Write 2" class="Bool"("DisabledEnum"=w84) -> ()  [unwired: 2 in, 2 out]
            n41 = property on="Write 3" class="Bool"("DisabledEnum"=w84) -> ()  [unwired: 2 in, 2 out]
            n42 = property on="Write 4" class="Bool"("DisabledEnum"=w84) -> ()  [unwired: 2 in, 2 out]
            n43 = property on="Write 5" class="Bool"("DisabledEnum"=w84) -> ()  [unwired: 2 in, 2 out]
            n44 = property on="Write 6" class="Bool"("DisabledEnum"=w84) -> ()  [unwired: 2 in, 2 out]
            n45 = property on="Write 7" class="Bool"("DisabledEnum"=w84) -> ()  [unwired: 2 in, 2 out]
            n46 = property on="Write 8" class="Bool"("DisabledEnum"=w84) -> ()  [unwired: 2 in, 2 out]
            n47 = property on="Write 9" class="Bool"("DisabledEnum"=w84) -> ()  [unwired: 2 in, 2 out]
            n48 = property on="Write 10" class="Bool"("DisabledEnum"=w84) -> ()  [unwired: 2 in, 2 out]
            n49 = property on="Write 11" class="Bool"("DisabledEnum"=w84) -> ()  [unwired: 2 in, 2 out]
          }
        }
      }
      event "Write": Value Change {
        n50 = event-data() -> ()  [unwired: 1 in, 6 out]
        n51 = disable-structure shown="Disabled" {
          frame Disabled {
            n52 = call "HEWH Write Standard Tests.vi"() -> ()  [unwired: 10 in, 2 out]
          }
          frame Enabled {
          }
        }
      }
      event "24 Hour DOE - Standard": Value Change {
        n53 = event-data() -> ()  [unwired: 1 in, 6 out]
        n54 = property on="New Cycle Count" class="DigNum (strict)"("Value"=0 ("New Cycle Count")) -> ()  [unwired: 2 in, 2 out]
        n55 = property on="Update for Northern Climate" class="Bool"("DisabledEnum"=T33."Enabled" ("Disabled")) -> ()  [unwired: 2 in, 2 out]
        n56 = property on="Update Cycle Count" class="Bool (strict)"("Value"=TRUE ("Update Cycle Count")) -> ()  [unwired: 2 in, 2 out]
        n57 = property on="24HR Test - Standard" class="Arr (strict)"() -> ("Label.Text"=w92:string)  [unwired: 2 in, 2 out]
      }
      event "24 Hour DOE - High Usage": Value Change {
        n58 = event-data() -> ()  [unwired: 1 in, 6 out]
        n59 = property on="Update Cycle Count" class="Bool (strict)"("Value"=TRUE ("Update Cycle Count")) -> ()  [unwired: 2 in, 2 out]
        n60 = property on="Update for Northern Climate" class="Bool"("DisabledEnum"=T33."Enabled" ("Disabled")) -> ()  [unwired: 2 in, 2 out]
        n61 = property on="New Cycle Count" class="DigNum (strict)"("Value"=0 ("New Cycle Count")) -> ()  [unwired: 2 in, 2 out]
        n62 = property on="24HR Test - High Usage" class="Arr (strict)"() -> ("Label.Text"=w102:string)  [unwired: 2 in, 2 out]
      }
      event "24 Hour DOE - Medium Usage": Value Change {
        n63 = event-data() -> ()  [unwired: 1 in, 6 out]
        n64 = property on="Update Cycle Count" class="Bool (strict)"("Value"=TRUE ("Update Cycle Count")) -> ()  [unwired: 2 in, 2 out]
        n65 = property on="New Cycle Count" class="DigNum (strict)"("Value"=0 ("New Cycle Count")) -> ()  [unwired: 2 in, 2 out]
        n66 = property on="Update for Northern Climate" class="Bool"("DisabledEnum"=T33."Enabled" ("Disabled")) -> ()  [unwired: 2 in, 2 out]
        n67 = property on="24HR Test - Medium Usage" class="Arr (strict)"() -> ("Label.Text"=w112:string)  [unwired: 2 in, 2 out]
      }
      event "24Hr Med Thermostat Test": Value Change {
        n68 = event-data() -> ()  [unwired: 1 in, 6 out]
        n69 = property on="Update Cycle Count" class="Bool (strict)"("Value"=TRUE ("Update Cycle Count")) -> ()  [unwired: 2 in, 2 out]
        n70 = property on="New Cycle Count" class="DigNum (strict)"("Value"=0 ("New Cycle Count")) -> ()  [unwired: 2 in, 2 out]
        n71 = property on="Update for Northern Climate" class="Bool"("DisabledEnum"=T33."Enabled" ("Disabled")) -> ()  [unwired: 2 in, 2 out]
        n72 = property on="24HR Medium Thermostat Test" class="Arr (strict)"() -> ("Label.Text"=w123:string)  [unwired: 2 in, 2 out]
      }
      event "24Hr High Thermostat Test": Value Change {
        n73 = event-data() -> ()  [unwired: 1 in, 6 out]
        n74 = property on="Update Cycle Count" class="Bool (strict)"("Value"=TRUE ("Update Cycle Count")) -> ()  [unwired: 2 in, 2 out]
        n75 = property on="New Cycle Count" class="DigNum (strict)"("Value"=0 ("New Cycle Count")) -> ()  [unwired: 2 in, 2 out]
        n76 = property on="Update for Northern Climate" class="Bool"("DisabledEnum"=T33."Enabled" ("Disabled")) -> ()  [unwired: 2 in, 2 out]
        n77 = property on="24Hr High Thermostat Test Profile" class="Arr (strict)"() -> ("Label.Text"=w132:string)  [unwired: 2 in, 2 out]
      }
      event "24 Hour DOE - Low Usage": Value Change {
        n78 = event-data() -> ()  [unwired: 1 in, 6 out]
        n79 = property on="Update Cycle Count" class="Bool (strict)"("Value"=TRUE ("Update Cycle Count")) -> ()  [unwired: 2 in, 2 out]
        n80 = property on="New Cycle Count" class="DigNum (strict)"("Value"=0 ("New Cycle Count")) -> ()  [unwired: 2 in, 2 out]
        n81 = property on="Update for Northern Climate" class="Bool"("DisabledEnum"=T33."Enabled" ("Disabled")) -> ()  [unwired: 2 in, 2 out]
        n82 = property on="24HR Test - Low Usage" class="Arr (strict)"() -> ("Label.Text"=w142:string)  [unwired: 2 in, 2 out]
      }
      event "1st Hour DOE": Value Change {
        n83 = event-data() -> ()  [unwired: 1 in, 6 out]
        n84 = property on="New Cycle Count" class="DigNum (strict)"("Value"=0 ("New Cycle Count")) -> ()  [unwired: 2 in, 2 out]
        n85 = property on="Update for Northern Climate" class="Bool"("DisabledEnum"=T33."Enabled" ("Disabled")) -> ()  [unwired: 2 in, 2 out]
        n86 = property on="Update Cycle Count" class="Bool (strict)"("Value"=TRUE ("Update Cycle Count")) -> ()  [unwired: 2 in, 2 out]
        n87 = property on="1st HR Test" class="Arr (strict)"() -> ("Label.Text"=w152:string)  [unwired: 2 in, 2 out]
      }
      event "Standard Heat-Up": Value Change {
        n88 = event-data() -> ()  [unwired: 1 in, 6 out]
        n89 = property on="New Cycle Count" class="DigNum (strict)"("Value"=0 ("New Cycle Count")) -> ()  [unwired: 2 in, 2 out]
        n90 = property on="Update Cycle Count" class="Bool (strict)"("Value"=TRUE ("Update Cycle Count")) -> ()  [unwired: 2 in, 2 out]
        n91 = property on="Update for Northern Climate" class="Bool"("DisabledEnum"=T33."Enabled" ("Disabled")) -> ()  [unwired: 2 in, 2 out]
        n92 = call "HEWH HeatUp Test Selector.vi"("Standard Heat-Up (80 Gallon) Heat Pump"="Standard Heat-Up (80 Gallon) Heat Pump", "Standard Heat-Up (80 Gallon)"="Standard Heat-Up (80 Gallon)", "Standard Heat-Up (50 Gallon) Heat Pump in"="Standard Heat-Up (50 Gallon) Heat Pump", "Error In"=w168, "Heating Mode"="Heating Mode", "Unit Type"="Unit Type", "Standard Heat-Up (50 Gallon)"="Standard Heat-Up (50 Gallon)") -> ("Error Out"=w167:errorcluster, "Standard Heat-Up (50 Gallon) Heat Pump out"=w177:T21[])  [unwired: 3 in]
      }
      event "Heat-Up Audit Test": Value Change {
        n93 = event-data() -> ()  [unwired: 1 in, 6 out]
        n94 = property on="New Cycle Count" class="DigNum (strict)"("Value"=0 ("New Cycle Count")) -> ()  [unwired: 2 in, 2 out]
        n95 = property on="Update for Northern Climate" class="Bool"("DisabledEnum"=T33."Enabled" ("Disabled")) -> ()  [unwired: 2 in, 2 out]
        n96 = property on="Update Cycle Count" class="Bool (strict)"("Value"=TRUE ("Update Cycle Count")) -> ()  [unwired: 2 in, 2 out]
        n97 = local read "Heating Mode"() -> (w184:string)
        n98 = local read "Unit Type"() -> (w185:T29)
        n99 = call "HEWH HeatUp Test Selector.vi"("Standard Heat-Up (80 Gallon) Heat Pump"="Heat-Up Audit Test - Heat Pump (80 Gallon)", "Standard Heat-Up (80 Gallon)"="Heat-Up Audit Test (80 Gallon)", "Standard Heat-Up (50 Gallon) Heat Pump in"="Heat-Up Audit Test (50 Gallon) Heat Pump", "Error In"=w188, "Heating Mode"=w184, "Unit Type"=w185, "Standard Heat-Up (50 Gallon)"="Heat-Up Audit Test (50 Gallon)") -> ("Error Out"=w187:errorcluster, "Standard Heat-Up (50 Gallon) Heat Pump out"=w183:T21[])  [unwired: 3 in]
      }
      event "PRAT 1 Year Equiv": Value Change {
        n100 = event-data() -> ()  [unwired: 1 in, 5 out]
        n101 = property on="Update for Northern Climate" class="Bool"("DisabledEnum"=T33."Enabled" ("Disabled")) -> ()  [unwired: 2 in, 2 out]
        n102 = local write "Update Cycle Count"(TRUE ("Update Cycle Count")) -> ()
        n103 = call "HCC Read Write Display.vi"("Read Write Control"=enum16{"Read", "Write"}."Read", "error in (no error)"=w200, "File Locations In"=w201) -> ("error out"=w199:errorcluster, "Washer Output"=w202:T18)  [unwired: 7 in]
        n104 = Unbundle By Name(w202) -> ("Display Data (RLT).Cycle Count Display"=w198:i32)
        n105 = property on="1 Year Standard" class="Arr (strict)"() -> ("Label.Text"=w196:string)  [unwired: 2 in, 2 out]
      }
      event "PRAT 2.5 Year Equiv": Value Change {
        n106 = event-data() -> ()  [unwired: 1 in, 5 out]
        n107 = property on="Update for Northern Climate" class="Bool"("DisabledEnum"=T33."Enabled" ("Disabled")) -> ()  [unwired: 2 in, 2 out]
        n108 = local write "Update Cycle Count"(TRUE ("Update Cycle Count")) -> ()
        n109 = call "HCC Read Write Display.vi"("Read Write Control"=enum16{"Read", "Write"}."Read", "error in (no error)"=w211, "File Locations In"=w209) -> ("error out"=w210:errorcluster, "Washer Output"=w214:T18)  [unwired: 7 in]
        n110 = Unbundle By Name(w214) -> ("Display Data (RLT).Cycle Count Display"=w212:i32)
        n111 = property on="2.5 Years Standard" class="Arr (strict)"() -> ("Label.Text"=w208:string)  [unwired: 2 in, 2 out]
      }
      event "RLT": Value Change {
        n112 = event-data() -> ()  [unwired: 1 in, 5 out]
        n113 = property on="Update for Northern Climate" class="Bool"("DisabledEnum"=T33."Enabled" ("Disabled")) -> ()  [unwired: 2 in, 2 out]
        n114 = local write "Update Cycle Count"(TRUE ("Update Cycle Count")) -> ()
        n115 = call "HCC Read Write Display.vi"("Read Write Control"=enum16{"Read", "Write"}."Read", "error in (no error)"=w224, "File Locations In"=w221) -> ("error out"=w223:errorcluster, "Washer Output"=w226:T18)  [unwired: 7 in]
        n116 = Unbundle By Name(w226) -> ("Display Data (RLT).Cycle Count Display"=w222:i32)
        n117 = property on="RLT" class="Arr (strict)"() -> ("Label.Text"=w220:string)  [unwired: 2 in, 2 out]
      }
      event "Custom Test": Value Change {
        n118 = event-data() -> ()  [unwired: 1 in, 5 out]
        n119 = property on="Update for Northern Climate" class="Bool"("DisabledEnum"=T33."Enabled" ("Disabled")) -> ()  [unwired: 2 in, 2 out]
        n120 = property on="Custom Test" class="Arr (strict)"() -> ("Label.Text"=w232:string)  [unwired: 2 in, 2 out]
      }
      event "Complete/Update": Value Change {
        n121 = event-data() -> ()  [unwired: 1 in, 5 out]
      }
      event Panel Close; "Cancel": Value Change {
        w260 = TRUE
        n122 = event-data() -> ()  [unwired: 1 in, 3 out]
      }
      event "Update for Northern Climate": Value Change {
        n123 = event-data() -> ("NewVal"=w267:bool)  [unwired: 1 in, 5 out]
        n124 = for {
          tunnel: w269 -> [w273] mode=indexing
          tunnel: [w272] -> w268 mode=indexing
          tunnel: w267 -> [w270]
          n125 = case shown="False" w270 {
            tunnel: [58.0 "Northern Climate\nInlet Temperature (°F)"] -> w271
            frame False {
            }
            frame True {
            }
          }
          n126 = Bundle By Name(cluster=w273, "Temperature (F)"=w271) -> (w272:T21)
        }
      }
      event "Test Sequence Output": Value Change {
        # "If you just want to update the sequence directly. You can"
        n127 = event-data() -> ()  [unwired: 1 in, 6 out]
      }
      event "Log Data": Value Change {
        n128 = event-data() -> ("NewVal"=w287:bool)  [unwired: 1 in, 5 out]
        n129 = case shown="True" w287 {
          tunnel: w295 -> [w300 w312]
          tunnel: [w300 w311] -> w294
          tunnel: w292 -> [w298 w310]
          tunnel: w291 -> [_ w305]
          tunnel: w290 -> [w301 w309]
          tunnel: [w301 w307] -> w289
          tunnel: [w297 w303] -> w288
          tunnel: [path "" ("Data File Path") w306] -> w286
          frame False {
            n130 = Bundle By Name(cluster=w298, "New Summary Created"=FALSE) -> (w297:T7)
          }
          frame True {
            n131 = call "Save File DOE File Setup.vi"("Filepath In"=w310, "Washer Controls In"=w309, "error in (no error)"=w312, "Config State"=Save_File_DOE_Configuration_State."Open Front Panel", "LV Program"=w305) -> ("Washer Controls Out"=w307:T9, "Filepath Out"=w304:T7, "error out"=w311:errorcluster)  [unwired: 12 in]
            n132 = Unbundle By Name(w304) -> ("Data File Paths.Data File Path"=w306:path)
            n133 = Bundle By Name(cluster=w304, "New Summary Created"=TRUE) -> (w303:T7)
          }
        }
        "Save File Path" <- w286
      }
      event "Read Previous Cycle Count": Value Change {
        n134 = event-data() -> ()  [unwired: 1 in, 6 out]
        n135 = call "HCC Read Write Display.vi"("Read Write Control"=enum16{"Read", "Write"}."Read", "error in (no error)"=w322, "File Locations In"=w316) -> ("error out"=w321:errorcluster, "Washer Output"=w319:T18)  [unwired: 7 in]
        n136 = Unbundle By Name(w319) -> ("Display Data (RLT).Cycle Count Display"=w318:i32)
      }
      event "Update": Value Change {
        n137 = event-data() -> ()  [unwired: 1 in, 6 out]
        n138 = for {
          tunnel: w329 -> [w333] mode=indexing
          tunnel: [w331] -> w328 mode=indexing
          n139 = Unbundle By Name(w333) -> ("Terminate Condition"=w335:T23)
          n140 = Equal?(x=w335, y=Terminate_Draw_Conditions."C5-Decrease RTD Out (Deg F)") -> (x = y?=w332:bool)
          n141 = case shown="True" w332 {
            tunnel: w333 -> [w336 w339]
            tunnel: [w336 w337] -> w331
            frame False {
            }
            frame True {
              n142 = Bundle By Name(cluster=w339, "Condition Value #1"="Temperature Decrease (°F)") -> (w337:T21)
            }
          }
        }
      }
      event "Seconds": Value Change {
        n143 = event-data() -> ()  [unwired: 1 in, 6 out]
        n144 = call "UTILITY Seconds To Time.vi"("Error In"=w341, "Time in Seconds"="Seconds") -> ("Error Out"=w340:errorcluster, "Time"=→"Time":string)  [unwired: 8 in]
      }
      event "Time Conv2": Value Change {
        n145 = event-data() -> ()  [unwired: 1 in, 6 out]
        "Seconds Conv2" <- "Time Conv2"
      }
    }
    "Reset Cycle Count" <- w64
    "Cancel Output" <- w63
    "Log Data Output" <- w61
    n146 = local write "Test Sequence Output"(w62) -> ()
    n147 = local write "Test Procedure"(w46) -> ()
    n148 = local write "New Cycle Count"(w49) -> ()
    n149 = Wait Until Next ms Multiple(millisecond multiple=u32 100) -> ()  [unwired: 1 out]
  }
  "Error Out" <- w27
  "Final Output" <- w16
  "Filepath Out" <- w11
  "Cutout Delay (sec)" <- w6
  "Unit Setpoint Out" <- w5
  "New Cycle Count Out" <- w4
  "Test Procedure" <- w1
  n150 = disable-structure shown="Disabled" {
    frame Disabled {
      n151 = call "HEWH Read Standard Test.vi"("Test Data Path"="Test Data Path") -> ()  [unwired: 10 in, 1 out]
    }
    frame Enabled {
    }
  }
  n152 = Unbundle By Name(w10) -> ("Initialize.Washer In.Appliance Details"=→"Appliance Details":T1)
